vi "Main.vi"(11 "Module Admin":refnum<class "Delacor_lib_QMH_Module Admin.lvclass">) -> ()   [LabVIEW 2019, in "CML UI.lvlib"]
doc: "This template is based off of the Queued Message Handler design pattern and the Queued Message Handler project template that ships with LabVIEW.\n\nThe main difference is that the queue is private to this module and communication between modules is performed via Broadcast and Request events.\n\nRequest events are wrapped in public API methods and are handled in the Event Handling Loop (EHL) of this VI. Any module can register for Broadcast events sent by this module. The EHL generates messages based on user interface actions.\n\nThe Message Handling Loop (MHL) processes messages generated by the EHL, or by other messages. The messages are string values, so new messages can be added easily to the Message Cases case structure in the MHL. Each message cluster can also provide an optional value for Message Data, which is a variant that can be converted to whatever message-specific data is required.\n_____\nBased on Delacor QMH Project Template 4.0.0.47.\n_____\nBased on DQMH Project Template 6.1.0.94.\n\n<b>Note:</b> This VI was modified by the <b>Validate DQMH Module</b> tool to add a call to the Error Reported VI at the end of the 'Exit' MHL frame."
uses:
  CML UI.lvlib
  <vilib>/Delacor/Delacor QMH/Libraries/Module Admin_class/Delacor_lib_QMH_Module Admin.lvclass
  Module Data--cluster.ctl
  Acquisition State.ctl
  Measurement UI Displays.ctl
  CNV demo Helper Loop Data--cluster.ctl
  Stop Argument--cluster.ctl
  <vilib>/Delacor/Delacor QMH/Libraries/Message Queue_class/Delacor_lib_QMH_Message Queue.lvclass/Delacor_lib_QMH_Message Queue.ctl
  <vilib>/event_ctls.llb/eventvkey.ctl
  STOP_GUI Argument--cluster.ctl
  Clear All Charts Argument--cluster.ctl
  Update Data Status UI Argument--cluster.ctl
  Update Packet Loss (%) Argument--cluster.ctl
  <vilib>/Utility/sysdir.llb/System Directory Type.ctl
  <vilib>/Delacor/Delacor QMH/Libraries/Module Admin_class/Delacor_lib_QMH_Module Admin.lvclass/Delacor_lib_QMH_Module Admin.ctl
  UI Tab Select.ctl
  Acquisition/WiBCI16T_Data.ctl
  Acquisition/WiBCI16T_Status.ctl
  Acquisition/Reg_Map.ctl
  <vilib>/Analysis/3filter.llb/Filter Passband Type.ctl
  Settings Editor/Settings--cluster.ctl
  Acquisition/Signal Type--enum.ctl
  Acquisition/Calibration Values--cluster.ctl
  CML Shared/EEG Channel Settings.ctl
  <vilib>/Delacor/Delacor QMH/Libraries/Message Queue_class/Delacor_lib_QMH_Enqueue Message (Single).vi
  <vilib>/Delacor/Delacor QMH/Libraries/Module Admin_class/Delacor_lib_QMH_Get External Launch.vi
  <vilib>/Analysis/baseanly.llb/Mean (DBL).vi
  <userlib>/_MGI/Timing/MGI Wait/MGI Wait (U32).vi
  <vilib>/addons/Biomedical/Biosignal Measurements/EEG/EEG FFT Spectrum (Waveform).vi
  <vilib>/Utility/error.llb/Error Cluster From Error Code.vi
  <vilib>/ErrorRing/Error Ring.xnode
  <vilib>/Delacor/Delacor QMH/Libraries/Message Queue_class/Delacor_lib_QMH_Message Queue.lvclass
  Settings Editor/Settings Editor.lvlib
  Acquisition/Acquisition.lvlib
  Logger/Logger.lvlib
  CML Shared/CML Shared.lvlib
  <vilib>/Analysis/NI_AALBase.lvlib
  <vilib>/addons/Biomedical/NI_BMTK_Measurements.lvlib
  DemoData Generator/DemoData Generator.lvlib
  Lab Streaming Layer/Lab Streaming Layer.lvlib
  <vilib>/ptbypt/NI_PtbyPt.lvlib
panel:
  out "Packet Loss (%)":dbl format="%#_3g"
  out "LSL Listeners":string
  out "En/Dis Trig":string
  in  "Settings":bool
  in  "Ref":bool
  out "Data Status":bool=TRUE
  out "Battery":u8(slide) scale=0.0..100.0
  in  "UI Page":T1(tab)
  out "Data Trig":i8(graph)
  out "Data 16":dbl(graph)
  out "Data 15":dbl(graph)
  out "Data 14":dbl(graph)
  out "Data 13":dbl(graph)
  out "Data 12":dbl(graph)
  out "Data 11":dbl(graph)
  out "Data 10":dbl(graph)
  out "Data 9":dbl(graph)
  out "Data 8":dbl(graph)
  out "Data 7":dbl(graph)
  out "Data 6":dbl(graph)
  out "Data 5":dbl(graph)
  out "Data 4":dbl(graph)
  out "Data 3":dbl(graph)
  out "Data 2":dbl(graph)
  out "Data 1":dbl(graph)
  in  "Stop":bool
  in  "Start":bool
  in  "Record Button":bool
  in  "Data Select":string(combo)="Live Data"
  out "Status":string
  out "G.Ch Name 1":string
  out "G.Ch Name 2":string
  out "G.Ch Name 3":string
  out "G.Ch Name 4":string
  out "G.Ch Name 5":string
  out "G.Ch Name 6":string
  out "G.Ch Name 7":string
  out "G.Ch Name 8":string
  out "G.Ch Name 9":string
  out "G.Ch Name 10":string
  out "G.Ch Name 11":string
  out "G.Ch Name 12":string
  out "G.Ch Name 13":string
  out "G.Ch Name 14":string
  out "G.Ch Name 15":string
  out "G.Ch Name 16":string
  in  "imp mode":bool
  out "ch 11":string
  out "ch 12":string
  out "ch 13":string
  out "ch 14":string
  out "ch 15":string
  out "ch 16":string
  out "ch 10":string
  out "ch 9":string
  out "ch 8":string
  out "ch 7":string
  out "ch 6":string
  out "ch 5":string
  out "ch 4":string
  out "ch 3":string
  out "ch 2":string
  out "ch 1":string
  in  "Stop Imped":bool
  in  "Start Imped":bool
  out "Imp Ch 16":bool
  out "Imp Ch 15":bool
  out "Imp Ch 14":bool
  out "Imp Ch 13":bool
  out "Imp Ch 12":bool
  out "Imp Ch 11":bool
  out "Imp Ch 10":bool
  out "Imp Ch 9":bool
  out "Imp Ch 8":bool
  out "Imp Ch 7":bool
  out "Imp Ch 6":bool
  out "Imp Ch 5":bool
  out "Imp Ch 4":bool
  out "Imp Ch 3":bool
  out "Imp Ch 2":bool
  out "Imp Ch 1":bool
  in  "Round Color Box 1":u32(colorbox)=16777215
  in  "Round Color Box 2":u32(colorbox)=3381759
  in  "Round Color Box 3":u32(colorbox)=6618880
  in  "Round Color Box 4":u32(colorbox)=16749312
  in  "Round Color Box 5":u32(colorbox)=16731714
  out "Ch Name 1":string
  out "Ch Name 2":string
  out "Ch Name 3":string
  out "Ch Name 4":string
  out "Ch Name 5":string
  out "Ch Name 6":string
  out "Ch Name 7":string
  out "Ch Name 8":string
  out "Ch Name 9":string
  out "Ch Name 10":string
  out "Ch Name 11":string
  out "Ch Name 12":string
  out "Ch Name 13":string
  out "Ch Name 14":string
  out "Ch Name 15":string
  out "Ch Name 16":string
  out "Single Chart":dbl(graph)
  in  "Visual Cue Tab":enum32{"Visual Cue Graph", "Ready", "Rest"}(tab)
  out "Visual Cue":i32[][](graph)
  in  "Display CNV Tab":enum32{"Empty", "Graph"}(tab)
  out "CNV Graph":dbl[][](graph)
  in  "Start CNV":bool
  in  "Stop CNV":bool
  in  "Record CNV":bool
  in  "Record EOC":bool
  in  "Stop EOC":bool
  in  "Start EOC":bool
  out "Theta":u8(slide) scale=10.0..90.0
  out "Alpha":u8(slide) scale=10.0..90.0
  out "Beta":u8(slide) scale=10.0..90.0
  out "Display Label EOC":string
  in  "About DQMH":bool
  out "Logger Running?":bool
  out "Settings Editor Running?":bool
  out "Acquisition Running?":bool
  out "Calibrated?":bool
  in  "Calibrate":bool
  out "error out":errorcluster
  out "version":string
  # "Connection"
  # "TRIG"
  # "Ch. 1"
  # "Ch. 9"
  # "Ch. 2"
  # "Ch. 10"
  # "Legend"
  # "Unknown"
  # "Ch. 3"
  # "Ch. 11"
  # "Excellent"
  # "Ch. 4"
  # "Ch. 12"
  # "Good"
  # "Average"
  # "Ch. 5"
  # "Ch. 13"
  # "Bad"
  # "Ch. 6"
  # "Ch. 14"
  # "Ch. 7"
  # "Ch. 15"
  # "Ch. 8"
  # "Ch. 16"
  # "Ready !"
  # "Rest"
  # "Theta"
  # "Alpha"
  # "Beta"
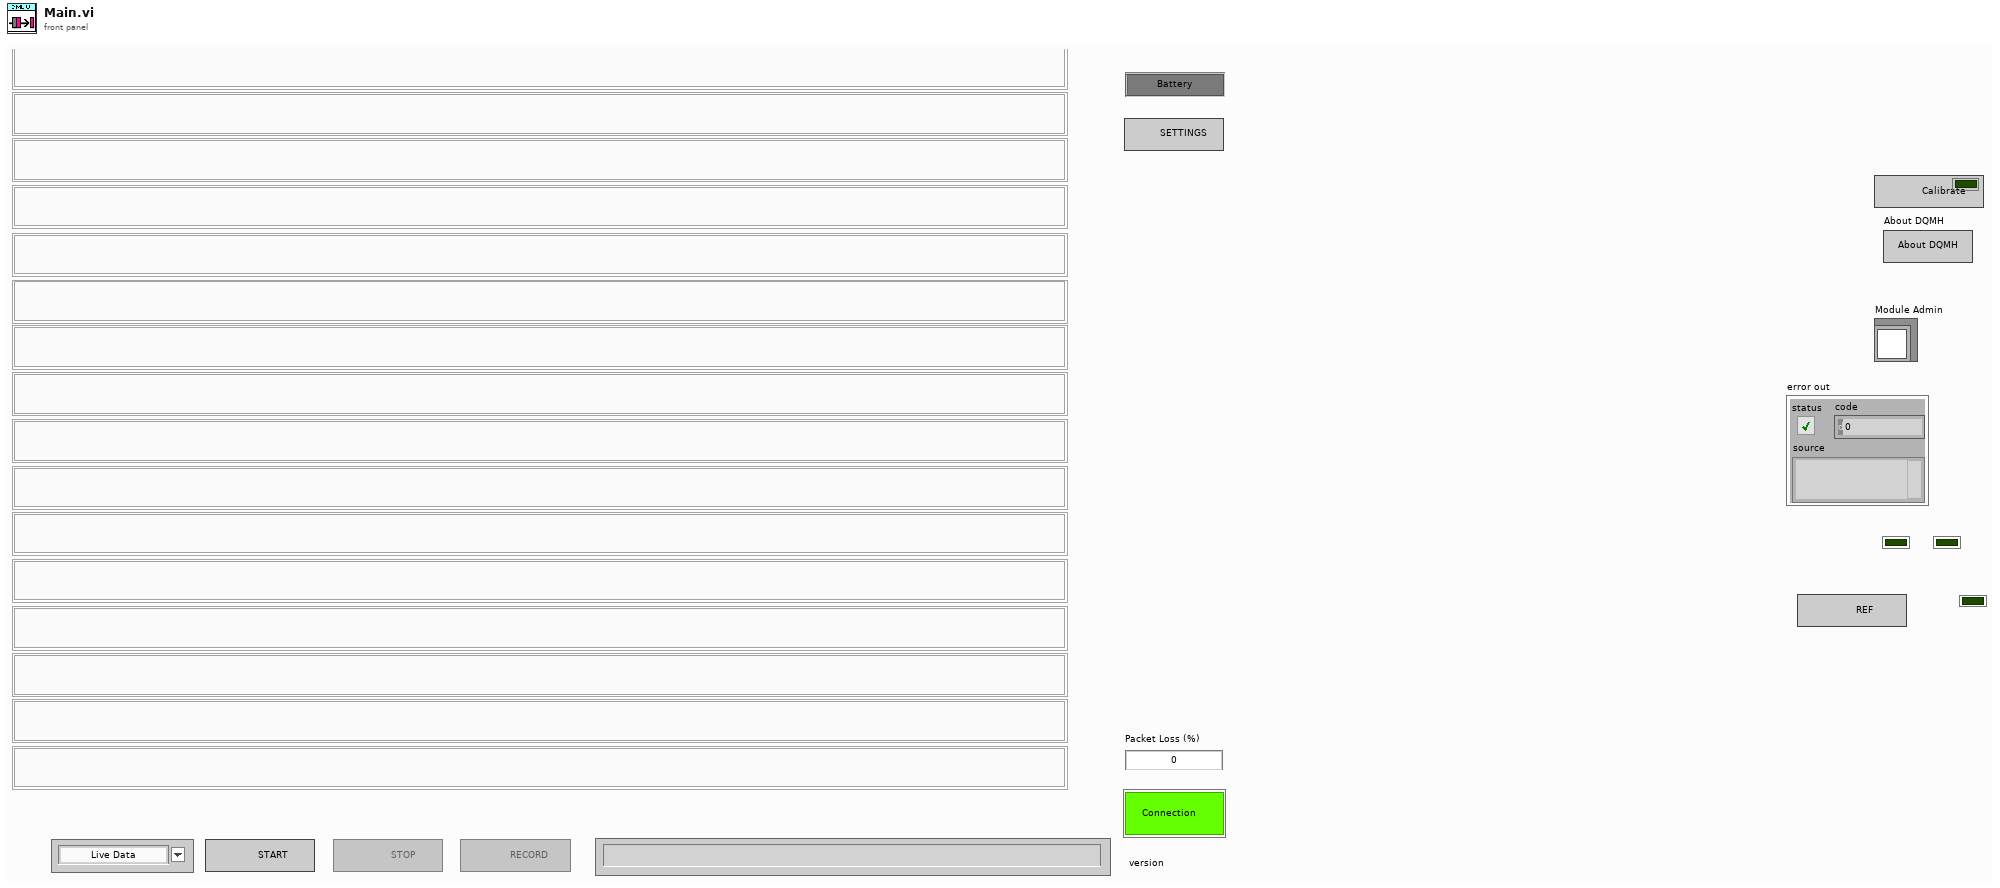
[diagram p1: front panel]
types:
  T1 = enum32{"Graph", "Impedance", "More Options", "Single Graph", "CNV Demo", "Eyes O/C Demo"}
  T2 = typedef "Settings Editor.lvlib/Broadcast Events--cluster.ctl" = cluster{"Module Did Init":refnum<user-event>, "Status Updated":refnum<user-event>, "Error Reported":refnum<user-event>, "Module Did Stop":refnum<user-event>, "Update Module Execution Status":refnum<user-event>, "Application Settings Updated":refnum<user-event>}
  T3 = typedef "Acquisition.lvlib/Broadcast Events--cluster.ctl" = cluster{"Module Did Init":refnum<user-event>, "Status Updated":refnum<user-event>, "Error Reported":refnum<user-event>, "Module Did Stop":refnum<user-event>, "Update Module Execution Status":refnum<user-event>, "Acquisition Started":refnum<user-event>, "Acquisition Stopped":refnum<user-event>, "Data Updated":refnum<user-event>, "Device Calibrated":refnum<user-event>, "Impedance Data Updated":refnum<user-event>, "CNV Data Updated":refnum<user-event>, "EOC Data Updated":refnum<user-event>}
  T4 = typedef "Logger.lvlib/Broadcast Events--cluster.ctl" = cluster{"Module Did Init":refnum<user-event>, "Status Updated":refnum<user-event>, "Error Reported":refnum<user-event>, "Module Did Stop":refnum<user-event>, "Update Module Execution Status":refnum<user-event>, "Logging Stopped":refnum<user-event>, "File Initialized":refnum<user-event>}
  T5 = typedef "DemoData Generator.lvlib/Broadcast Events--cluster.ctl" = cluster{"Module Did Init":refnum<user-event>, "Status Updated":refnum<user-event>, "Error Reported":refnum<user-event>, "Module Did Stop":refnum<user-event>, "Update Module Execution Status":refnum<user-event>, "Demo Data Generated":refnum<user-event>}
  T6 = typedef "Lab Streaming Layer.lvlib/Broadcast Events--cluster.ctl" = cluster{"Module Did Init":refnum<user-event>, "Status Updated":refnum<user-event>, "Error Reported":refnum<user-event>, "Module Did Stop":refnum<user-event>, "Update Module Execution Status":refnum<user-event>}
  T7 = typedef "CML UI.lvlib/Request Events--cluster.ctl" = cluster{"Stop Module":refnum<user-event>, "Show Panel":refnum<user-event>, "Hide Panel":refnum<user-event>, "Get Module Execution Status":refnum<user-event>, "Show Diagram":refnum<user-event>, "STOP_GUI":refnum<user-event>, "Clear All Charts":refnum<user-event>, "Update Data Status UI":refnum<user-event>, "Private":cluster{"Wake-Up File Name Query Loop":refnum<user-event>, "Wake-up CNV Demo Loop":refnum<user-event>, "Sleep CNV Demo Loop":refnum<user-event>, "Menu -- About Display Box":refnum<user-event>, "Wake-Up Copy MATLAB files":refnum<user-event>}, "Update Packet Loss (%)":refnum<user-event>}
  T8 = typedef "CML UI.lvlib/CNV demo Helper Loop Data--cluster.ctl" = cluster{"Visual Cue Tab":refnum<vi>, "Display CNV Tab":refnum<vi>, "Visual Cue Graph":refnum<vi>, "CNV Runner":cluster{"fixed array":i32[], "Loop Counter":i32}, "CNV Graph":refnum<vi>}
  T9 = typedef "CML UI.lvlib/Module Data--cluster.ctl" = cluster{"Status":string, "Measurement UI Controls":cluster{"Start Ref":refnum<vi>, "Stop Ref":refnum<vi>, "Settings Ref":refnum<vi>, "Status Ref":refnum<vi>, "Data Ref":refnum<vi>, "Rec Ref":refnum<vi>, "Soft Trig":refnum<vi>, "Imp Start Ref":refnum<vi>, "Imp Stop Ref":refnum<vi>, "CNV Start Ref":refnum<vi>, "CNV Stop Ref":refnum<vi>, "CNV Rec":refnum<vi>, "Recording State CNV":refnum<vi>, "EOC Start Ref":refnum<vi>, "EOC Stop Ref":refnum<vi>, "EOC Rec Ref":refnum<vi>, "CNV Rec state":refnum<vi>, "Recording State EOC":refnum<vi>}, "Recording State":bool, "Impedance":cluster{"Ch 1":dbl, "Ch 2":dbl, "Ch 3":dbl, "Ch 4":dbl, "Ch 5":dbl, "Ch 6":dbl, "Ch 7":dbl, "Ch 8":dbl, "Ch 9":dbl, "Ch 10":dbl, "Ch 11":dbl, "Ch 12":dbl, "Ch 13":dbl, "Ch 14":dbl, "Ch 15":dbl, "Ch 16":dbl}, "menu reference ":refnum<k9>, "Acq State":T10, "En/Dis Trig":refnum<vi>, "Soft Trigger En?":bool, "Display  cnt":u8, "UI Page":refnum<vi>, "CNV Demo Data":cluster{"Rebuild Vector":dbl[][], "CNV Buffer Action":enum16{"Stop Buffer Fill", "Start Buffer Fill", "Analyze Buffer"}, "Index of R.Array":u16, "Run Sum CNV":dbl[], "CNV Iter":u16}, "EOC Demo Data":cluster{"Running Buffer":dbl[], "Index of R.Buffer":u8}, "Measurement UI Displays":T11, "Recording State CNV":bool, "Recording State EOC":bool, "LSL En?":bool, "LSL Listeners":refnum<vi>, "Imp Mode":bool}
  T10 = typedef "CML UI.lvlib/Acquisition State.ctl" = enum16{"RUNNING", "IDLE"}
  T11 = typedef "CML UI.lvlib/Measurement UI Displays.ctl" = cluster{"Graph 1":refnum<vi>, "Graph 2":refnum<vi>, "Graph 3":refnum<vi>, "Graph 4":refnum<vi>, "Graph 5":refnum<vi>, "Graph 6":refnum<vi>, "Graph 7":refnum<vi>, "Graph 8":refnum<vi>, "Graph 9":refnum<vi>, "Graph 10":refnum<vi>, "Graph 11":refnum<vi>, "Graph 12":refnum<vi>, "Graph 13":refnum<vi>, "Graph 14":refnum<vi>, "Graph 15":refnum<vi>, "Graph 16":refnum<vi>, "Battery 2":refnum<vi>, "Data Trig":refnum<vi>, "Data Connection Status":refnum<vi>, "Graph Sel":u8, "En MAP":u16, "Single Chart":refnum<vi>, "G.Ch Name 1":refnum<vi>, "G.Ch Name 2":refnum<vi>, "G.Ch Name 3":refnum<vi>, "G.Ch Name 4":refnum<vi>, "G.Ch Name 5":refnum<vi>, "G.Ch Name 6":refnum<vi>, "G.Ch Name 7":refnum<vi>, "G.Ch Name 8":refnum<vi>, "G.Ch Name 9":refnum<vi>, "G.Ch Name 10":refnum<vi>, "G.Ch Name 11":refnum<vi>, "G.Ch Name 12":refnum<vi>, "G.Ch Name 13":refnum<vi>, "G.Ch Name 14":refnum<vi>, "G.Ch Name 15":refnum<vi>, "G.Ch Name 16":refnum<vi>, "imp mode sel":refnum<vi>}
  T12 = enum32{"invalid lock state", "Not Locked", "Locked (No Password)", "Password-protected"}
  T13 = typedef "CML UI.lvlib/Stop Argument--cluster.ctl" = cluster{"Origin":string, "Exit via Stop Module Req?":bool, "Wait for Module to stop?":bool}
  T14 = typedef "eventvkey.ctl" = enum16{"ASCII", "Enter", "Return", "Shift", "Ctrl", "Alt", "Cmd", "Opt", "Caps", "NumLock", "Clear", "Break", "Up", "Down", "Left", "Right", "Insert", "Delete", "Home", "End", "PageUp", "PageDown", "Escape", "Help", "Pause", "ScrollLock", "F1", "F2", "F3", "F4", "F5", "F6", "F7", "F8", "F9", "F10", "F11", "F12", "F13", "F14", "F15", "F16", "F17", "F18", "F19", "F20", "F21", "F22", "F23", "F24", "Play", "VolumeUp", "VolumeDown", "Mute", "Two Byte Char"}
  T15 = typedef "CML UI.lvlib/STOP_GUI Argument--cluster.ctl" = cluster{"Message for the Request":string}
  T16 = typedef "CML UI.lvlib/Clear All Charts Argument--cluster.ctl" = cluster{"Boolean":bool}
  T17 = typedef "CML UI.lvlib/Update Data Status UI Argument--cluster.ctl" = cluster{"status":bool}
  T18 = typedef "CML UI.lvlib/Update Packet Loss (%) Argument--cluster.ctl" = cluster{"Paket Loss":dbl}
  T19 = enum32{"Invalid", "Standard", "Closed", "Hidden", "Minimized", "Maximized"}
  T20 = typedef "CML UI.lvlib/UI Tab Select.ctl" = enum32{"Graph", "Impedance", "More Options", "Single Graph", "CNV Demo", "Eyes O/C Demo"}
  T21 = typedef "Acquisition.lvlib/WiBCI16T_Data.ctl" = cluster{"EEG Ch 1":dbl, "EEG Ch 2":dbl, "EEG Ch 3":dbl, "EEG Ch 4":dbl, "EEG Ch 5":dbl, "EEG Ch 6":dbl, "EEG Ch 7":dbl, "EEG Ch 8":dbl, "EEG Ch 9":dbl, "EEG Ch 10":dbl, "EEG Ch 11":dbl, "EEG Ch 12":dbl, "EEG Ch 13":dbl, "EEG Ch 14":dbl, "EEG Ch 15":dbl, "EEG Ch 16":dbl, "X-Accel":i16, "Y-Accel":i16, "Z-Accel":i16, "X-Gyro":i16, "Y-Gyro":i16, "Z-Gyro":i16, "Timer":u32, "Packet ID":u32, "HW Trig1":u8, "SW Trig1":i8, "HW Trig2":u8, "SW Trig2":i8, "WiBCI Status":T22, "Reg Map":T23}
  T22 = typedef "Acquisition.lvlib/WiBCI16T_Status.ctl" = cluster{"Mode Byte":u8, "Ch Config":u8, "Ch Ref Map":u16, "Ch Enable Map":u16, "Temperature":sgl, "Battery":u8, "Version":string}
  T23 = typedef "Acquisition.lvlib/Reg_Map.ctl" = cluster{"ADS1":u8[], "ADS2":u8[]}
  T24 = typedef "NI_AALBase.lvlib/Filter Passband Type.ctl" = enum32{"Lowpass", "Highpass", "Bandpass", "Bandstop"}
  T25 = enum16{"Stop Buffer Fill", "Start Buffer Fill", "Analyze Buffer"}
  T26 = typedef "Settings Editor.lvlib/Settings--cluster.ctl" = cluster{"Signal Type":T27, "Calibration Array":T28[], "Log File Base Path":path, "EEG Channels":T29, "Soft Trig enum":enum16{"Disable Soft Trigger", "Enable Soft Trigger"}, "Montage selection":cluster{"Montages Ref":refnum<vi>, "Selected Montage Number":u8, "Montages Names":string[]}, "LSL En enum":enum16{"LSL Disabled", "LSL Enabled"}}
  T27 = typedef "Acquisition.lvlib/Signal Type--enum.ctl" = enum16{"Sine Wave", "Square with Noise"}
  T28 = typedef "Acquisition.lvlib/Calibration Values--cluster.ctl" = cluster{"Slope":dbl, "Offset":dbl}
  T29 = typedef "CML Shared.lvlib/EEG Channel Settings.ctl" = cluster{"16 EEG Channels":cluster{"Channel Name":string, "Channel No":u8, "Channel Enabled":bool, "Channel Referenced":bool}[], "Gain":u8}
  T30 = typedef "Settings Editor.lvlib/Update Application Settings (Reply Payload)--cluster.ctl" = cluster{"Settings":T26, "error":errorcluster}
  T31 = cluster{"Channel Name":string, "Channel No":u8, "Channel Enabled":bool, "Channel Referenced":bool}[]
  T32 = typedef "NI_BMTK_Measurements.lvlib/bmt_EEG Frequency-domain Measures.ctl" = cluster{"delta power":dbl, "theta power":dbl, "alpha power":dbl, "beta power":dbl, "delta [%]":dbl, "theta [%]":dbl, "alpha [%]":dbl, "beta [%]":dbl}
  T33 = enum16{"Disable Soft Trigger", "Enable Soft Trigger"}
  T34 = typedef "System Directory Type.ctl" = i32
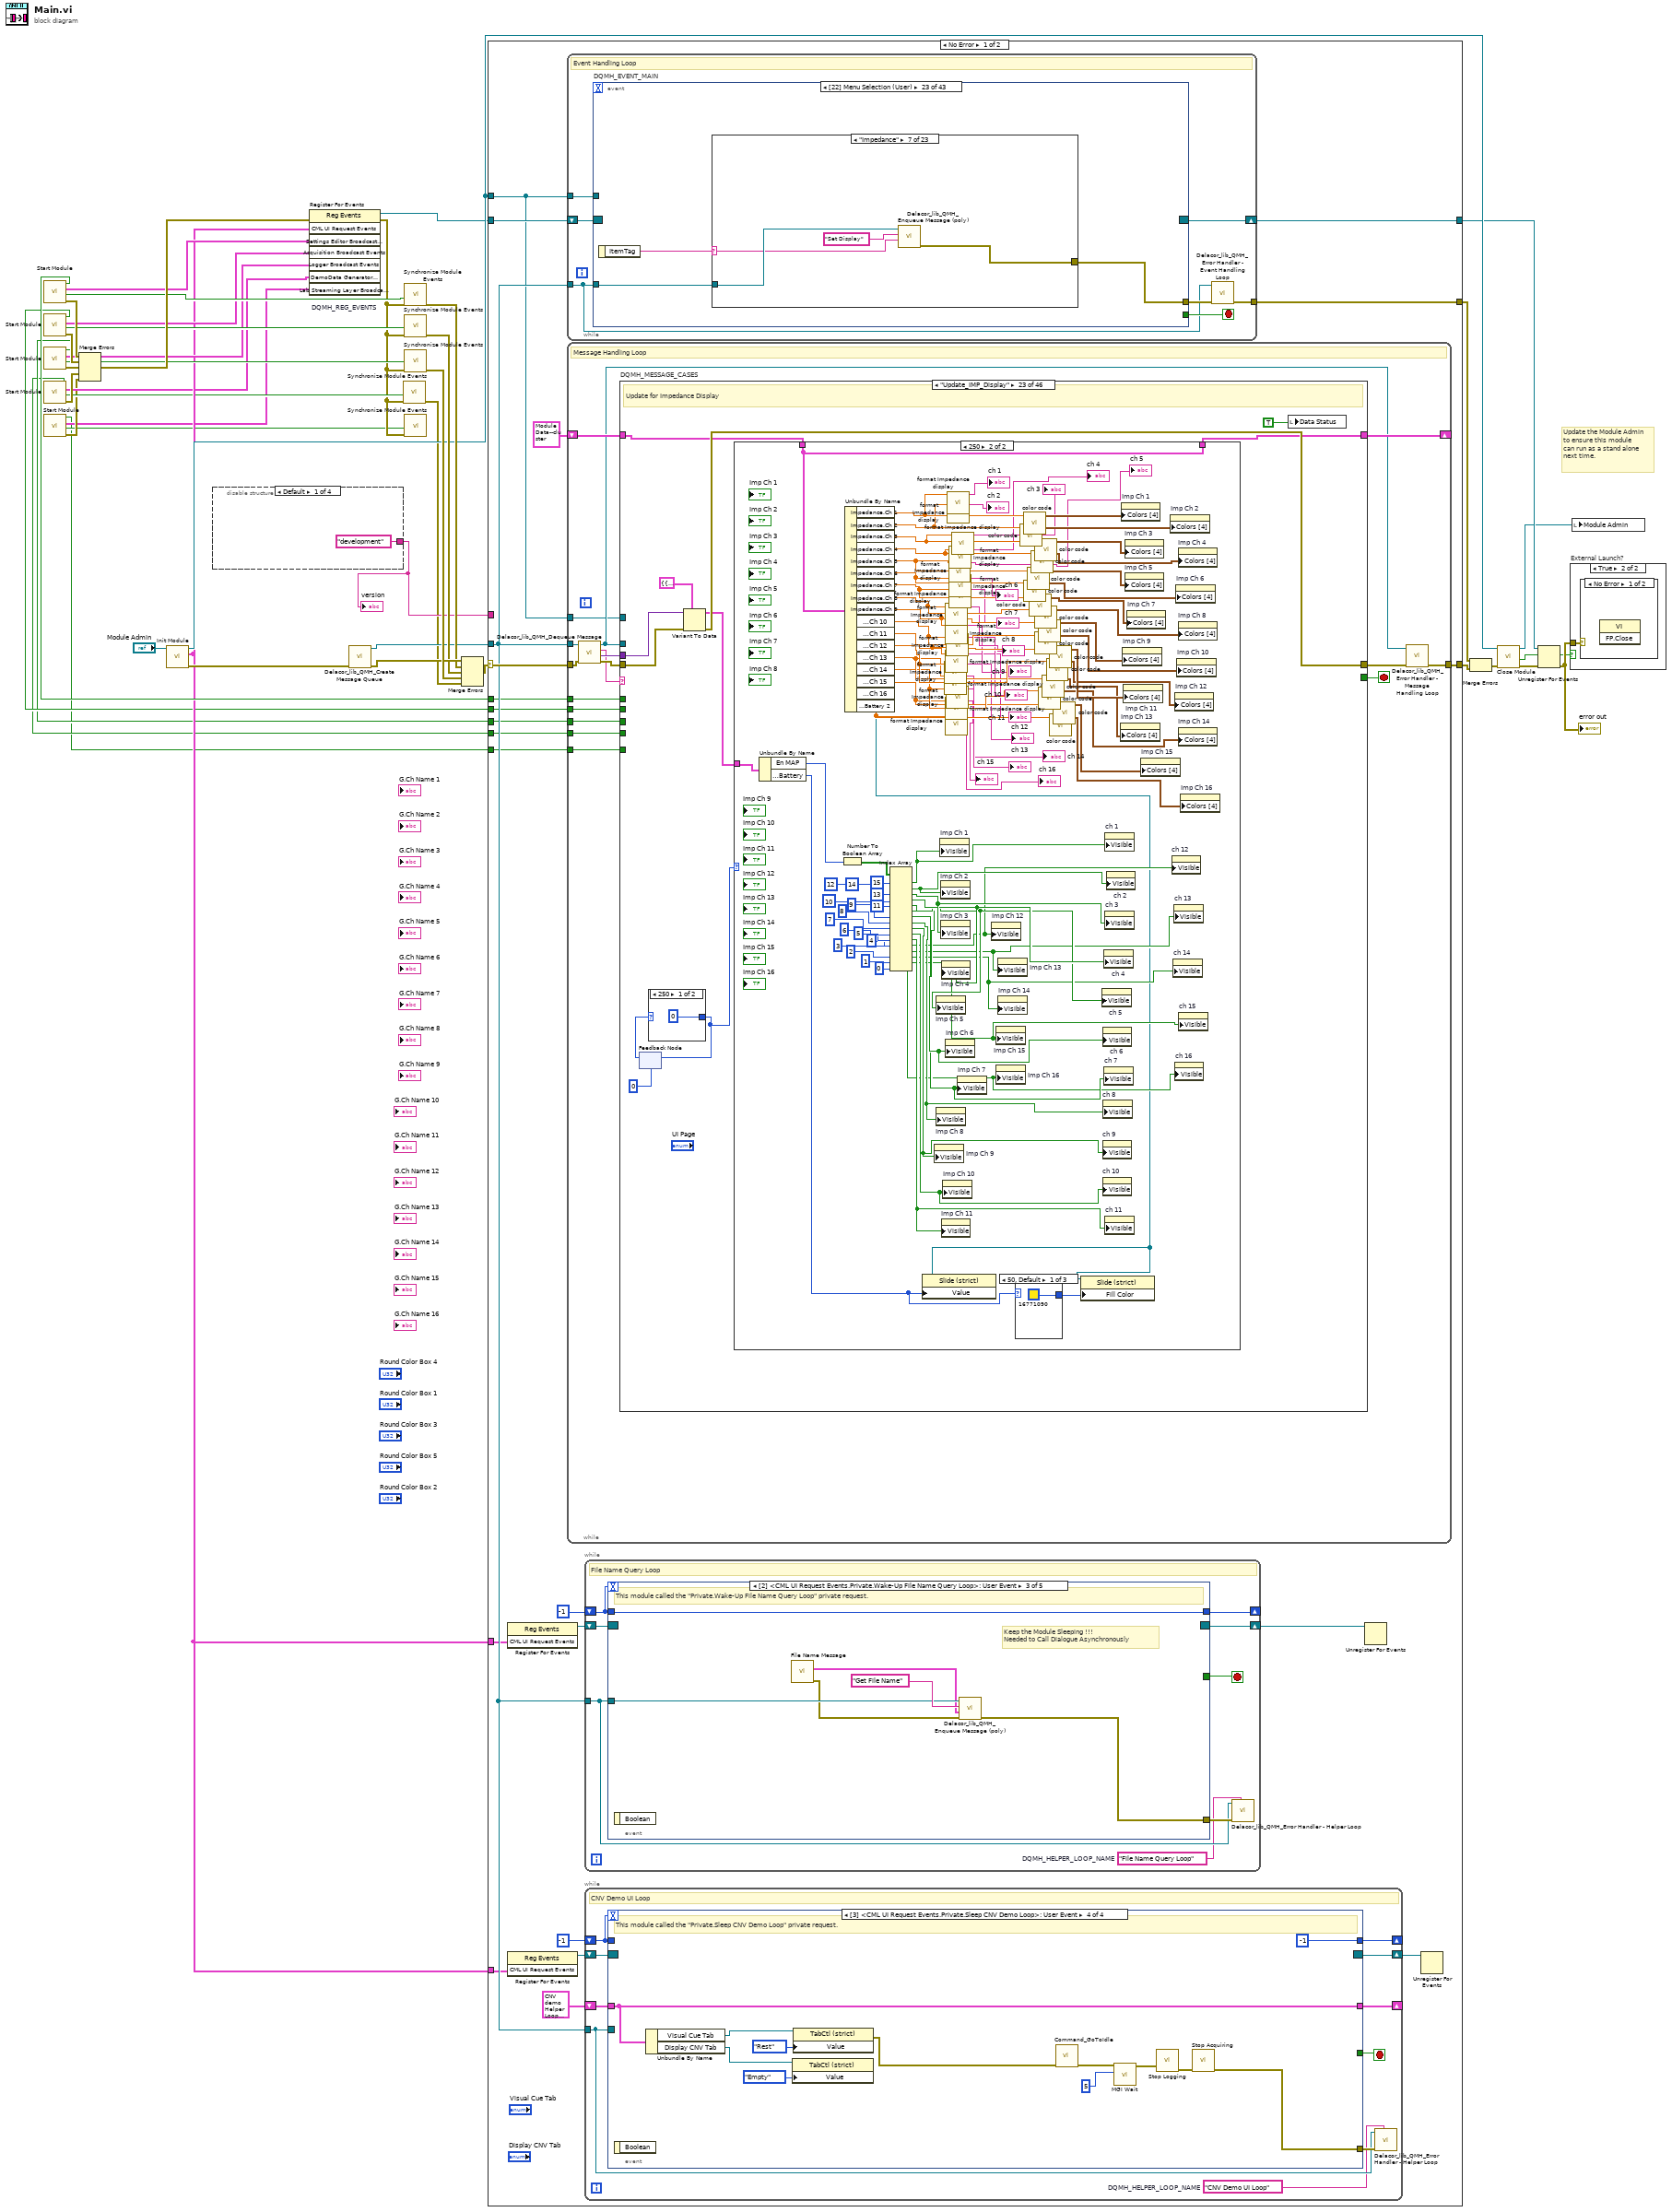
[diagram p0: block diagram]
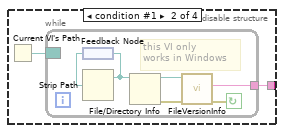
[diagram p2: hidden frame]
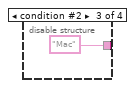
[diagram p3: hidden frame]
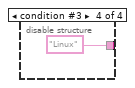
[diagram p4: hidden frame]
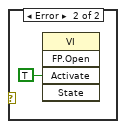
[diagram p6: hidden frame]
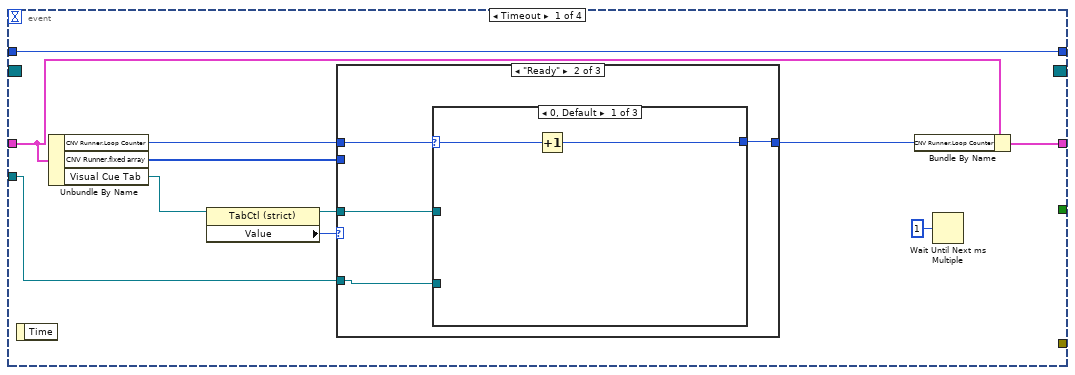
[diagram p7: hidden frame]
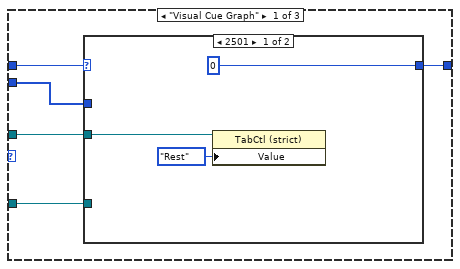
[diagram p8: hidden frame]
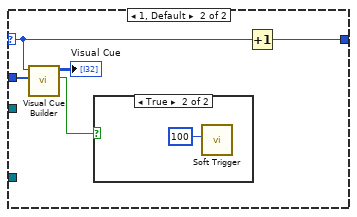
[diagram p9: hidden frame]
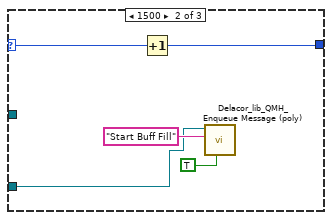
[diagram p11: hidden frame]
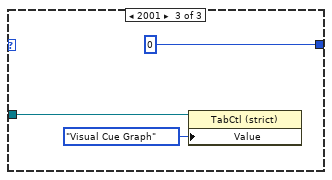
[diagram p12: hidden frame]
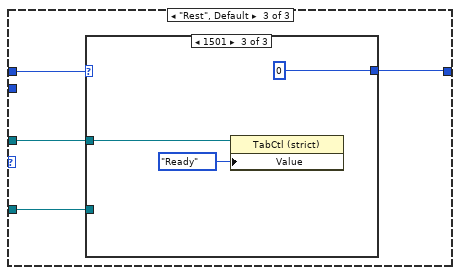
[diagram p13: hidden frame]
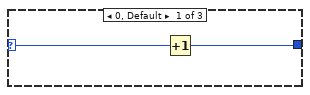
[diagram p14: hidden frame]
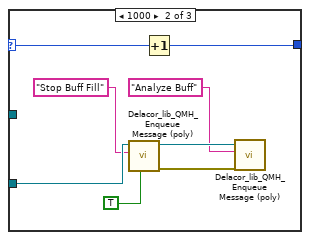
[diagram p15: hidden frame]
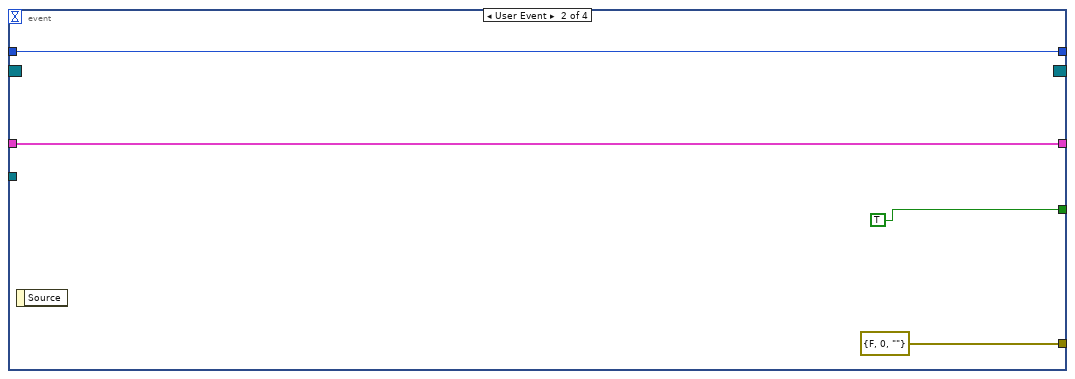
[diagram p16: hidden frame]
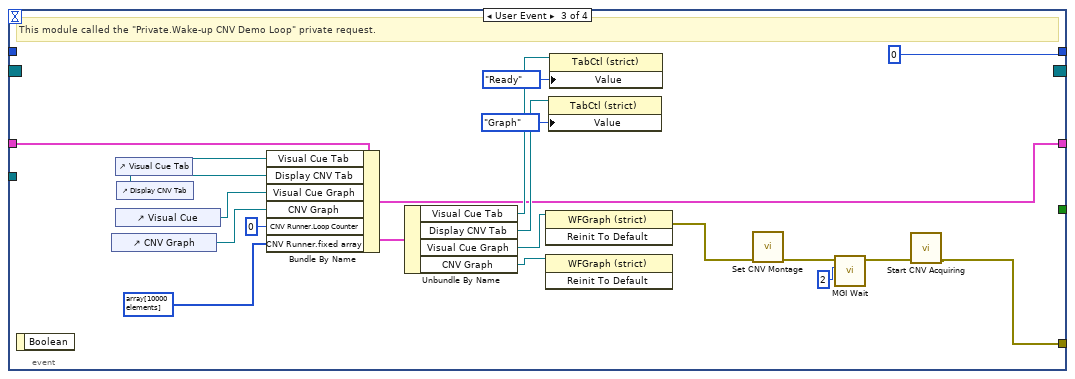
[diagram p17: hidden frame]
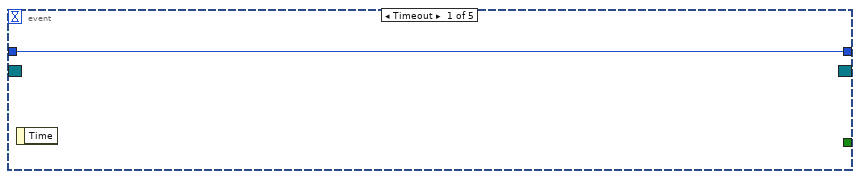
[diagram p18: hidden frame]
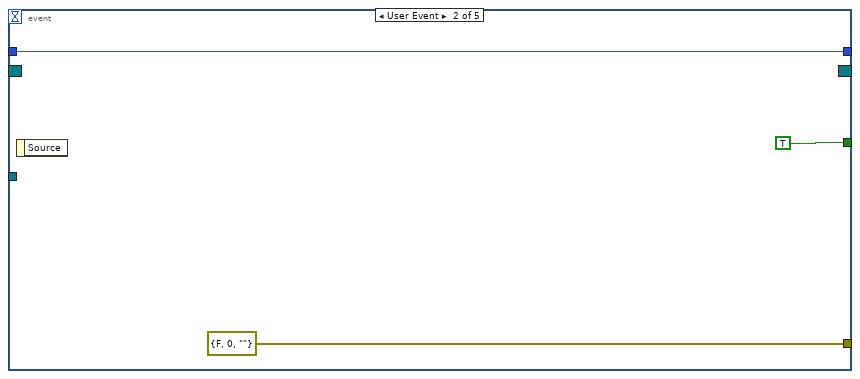
[diagram p19: hidden frame]
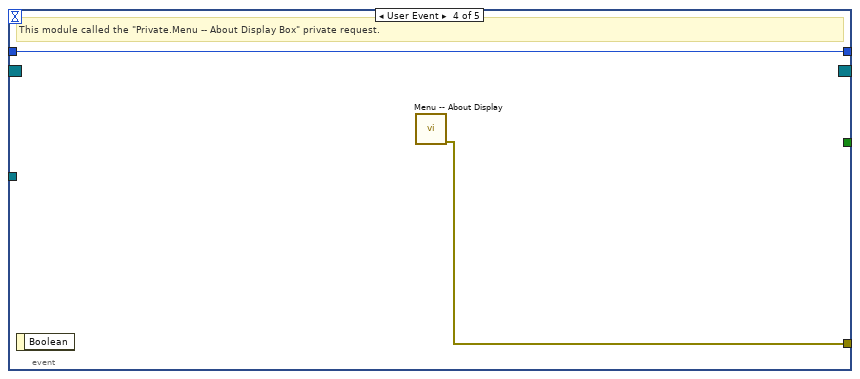
[diagram p20: hidden frame]
diagram:
  # "Update the Module Admin to ensure this module can run as a stand alone next time."
  n1 = call "Start Module.vi"() -> ("error out"=w32:errorcluster, "Wait for Event Sync?"=w21:bool, "Settings Editor Broadcast Events"=w20:T2, "Module Was Already Running?"=w14:bool)  [unwired: 8 in]
  n2 = call "Start Module.vi"() -> ("error out"=w31:errorcluster, "Wait for Event Sync?"=w18:bool, "Acquisition Broadcast Events"=w19:T3, "Module Was Already Running?"=w4:bool)  [unwired: 8 in]
  n3 = call "Start Module.vi"() -> ("error out"=w30:errorcluster, "Wait for Event Sync?"=w16:bool, "Logger Broadcast Events"=w17:T4, "Module Was Already Running?"=w3:bool)  [unwired: 8 in]
  n4 = call "Start Module.vi"() -> ("error out"=w12:errorcluster, "Wait for Event Sync?"=w10:bool, "DemoData Generator Broadcast Events"=w11:T5, "Module Was Already Running?"=w2:bool)  [unwired: 8 in]
  n5 = call "Start Module.vi"() -> ("error out"=w8:errorcluster, "Wait for Event Sync?"=w6:bool, "Lab Streaming Layer Broadcast Events"=w5:T6, "Module Was Already Running?"=w1:bool)  [unwired: 8 in]
  n6 = Merge Errors(w32, w31, w30, w12, w8) -> (w29:errorcluster)
  n7 = call "Init Module.vi"("Singleton Module Admin in"="Module Admin") -> ("error out"=w41:errorcluster, "CML UI Request Events"=w13:T7, "Singleton Module Admin out"=w28:refnum<class "Delacor_lib_QMH_Module Admin.lvclass">)  [unwired: 8 in]
  n8 = disable-structure "Conditional Disable Structure" shown="Default" {
    disable-tunnel: ["development" w45 "Mac" "Linux"] -> w15
    frame condition #0 (active) {
    }
    frame condition #1 {
      n9 = Current VI's Path() -> (path=w46:path)
      n10 = while {
        border: w46 -> [_]
        tunnel: [w47] -> w45
        stop <- w51 continue-if-true
        # "this VI only \nworks in Windows"
        n11 = feedback #1() -> (w50:path)
        n12 = Strip Path(path=w50) -> (stripped path=w49:path)  [unwired: 1 out]
        n13 = feedback-in #1(w49) -> ()
        n14 = File/Directory Info(path=w49) -> (path out=w48:path, error out=w52:errorcluster)  [unwired: 1 in, 5 out]
        n15 = call <vilib>:"FileVersionInfo.vi"("error in (no error)"=w52, "Application Path in"=w48) -> ("error out"=w51:errorcluster, "File Version Info"=w47:string)  [unwired: 6 in, 2 out]
      }
    }
    frame condition #2 {
    }
    frame condition #3 {
    }
  }
  "version" <- w15
  n16 = register-events "DQMH_REG_EVENTS"(error in=w29, w13, w20, w19, w17, w11, w5) -> (reference out=w26:refnum<event-registration>, error out=w7:errorcluster)  [unwired: 1 in]
  n17 = call <vilib>:"Delacor_lib_QMH_Create Message Queue.vi"("error in"=w41) -> ("error out"=w36:errorcluster, "Message Queue"=w25:refnum<class "Delacor_lib_QMH_Message Queue.lvclass">)  [unwired: 9 in]
  n18 = call "Synchronize Module Events.vi"("error in"=w7, "Wait for Event Sync?"=w10) -> ("error out"=w9:errorcluster)  [unwired: 9 in]
  n19 = call "Synchronize Module Events.vi"("error in (no error)"=w7, "Wait for Event Sync?"=w21) -> ("error out"=w34:errorcluster)  [unwired: 9 in]
  n20 = call "Synchronize Module Events.vi"("error in (no error)"=w7, "Wait for Event Sync?"=w18) -> ("error out"=w33:errorcluster)  [unwired: 9 in]
  n21 = call "Synchronize Module Events.vi"("error in (no error)"=w7, "Wait for Event Sync?"=w16) -> ("error out"=w43:errorcluster)  [unwired: 9 in]
  n22 = call "Synchronize Module Events.vi"("error in"=w7, "Wait for Event Sync?"=w6) -> ()  [unwired: 9 in, 1 out]
  n23 = Merge Errors(w36, w34, w33, w43, w9) -> (w35:errorcluster)
  n24 = case shown="No Error" w35 {
    selector: w35 -> [w74 w1637]
    tunnel: [w76 w1636] -> w42
    tunnel: [w73 w1645] -> w27
    tunnel: w26 -> [w71 w1645]
    tunnel: w25 -> [w70 w1638]
    tunnel: [w75 _] -> w39
    tunnel: w28 -> [w69 w1641]
    tunnel: w15 -> [_ _]
    tunnel: w14 -> [w68 _]
    tunnel: w13 -> [w67 _]
    tunnel: w13 -> [w63 _]
    tunnel: w4 -> [w58 _]
    tunnel: w3 -> [w57 _]
    tunnel: w2 -> [w56 _]
    tunnel: w1 -> [w55 _]
    frame No Error {
      n25 = register-events ("DQMH_HELPER_REGFOREVENTS")(w67) -> (reference out=w65:refnum<event-registration>)  [unwired: 2 in, 1 out]
      n26 = register-events ("DQMH_HELPER_REGFOREVENTS")(w63) -> (reference out=w61:refnum<event-registration>)  [unwired: 2 in, 1 out]
      n27 = while {
        tunnel: w70 -> [w220]
        shift-right: [w223] -> w73
        shift-left: w71 -> [w224]
        tunnel: [w225] -> w75
        tunnel: w69 -> [w221]
        stop <- w222 stop-if-true
        # "Event Handling Loop"
        n28 = event "DQMH_EVENT_MAIN" shown="[22] Menu Selection (User)" {
          selector: w224 -> [_ _ _ _ _ _ _ _ _ _ _ _ _ _ _ _ _ _ _ _ _ _ _ _ _ _ w417 _ _ _ _ _ _ _ _ _ _ _ _ _ _ _ _]
          dyn-events: [_ _ _ _ _ _ _ _ _ _ _ _ _ _ _ _ _ _ _ _ _ _ _ _ _ _ w417 _ _ _ _ _ _ _ _ _ _ _ _ _ _ _ _] -> w223
          timeout: _ -> [_ _ _ _ _ _ _ _ _ _ _ _ _ _ _ _ _ _ _ _ _ _ _ _ _ _ _ _ _ _ _ _ _ _ _ _ _ _ _ _ _ _ _]
          tunnel: [_ _ _ _ TRUE ("Discard?") _ _ _ _ _ _ _ _ _ _ _ _ _ _ _ _ _ _ _ _ _ _ _ _ _ _ _ _ _ _ _ _ _ _ _ _ _ _] -> w222
          tunnel: w220 -> [_ _ _ _ w249 w255 w259 w264 w269 w271 w274 w277 w280 w285 w289 w293 w296 w308 w318 w321 w324 _ w329 _ _ w406 _ _ _ _ w429 _ w434 w440 w446 w452 w458 _ _ w467 w474 _ w484]
          tunnel: [_ _ w232 _ w252 w257 w261 w263 w268 w270 w273 w278 w281 w284 w288 w292 w295 w310 w320 w323 w326 w327 w328 w400 _ w405 _ _ _ w427 _ _ w433 w439 w445 w451 w457 _ w461 w462 w469 _ w479] -> w226
          tunnel: w221 -> [_ _ _ _ _ _ _ _ _ _ _ _ _ _ _ _ _ _ _ _ _ _ _ _ _ _ _ _ _ _ _ _ _ _ _ _ _ _ _ _ _ _ _]
          event User Event {
            # "Show the panel of this VI, and send a status updated message to let listeners know."
            # "Another Module called the \"Show Panel\" API Method."
            n29 = event-data() -> ()  [unwired: 1 in, 1 out]
            n30 = control-ref of="This VI"() -> (w228:refnum<vi>)
            n31 = call "Open VI Panel.vi"("VI"=w228) -> ()  [unwired: 10 in, 1 out]
            n32 = call "Status Updated.vi"("Status"="Panel shown." ("format string")) -> ()  [unwired: 10 in, 1 out]
          }
          event User Event {
            # "Hide the panel of this VI, and send a status updated message to let listeners know."
            # "Another Module called the \"Hide Panel\" API Method."
            n33 = event-data() -> ()  [unwired: 1 in, 1 out]
            n34 = control-ref of="This VI"() -> (w230:refnum<vi>)
            n35 = call "Hide VI Panel.vi"("VI"=w230) -> ()  [unwired: 10 in, 1 out]
            n36 = call "Status Updated.vi"("Status"="Panel hidden." ("format string")) -> ()  [unwired: 10 in, 1 out]
          }
          event User Event {
            # "Another Module called the \"Get Module Execution Status\" API Method."
            n37 = event-data() -> ()  [unwired: 1 in, 1 out]
            n38 = call "Update Module Execution Status.vi"("Running?"=TRUE) -> ("error out"=w232:errorcluster)  [unwired: 10 in]
          }
          event User Event {
            # "Another Module called the \"Show Diagram\" API Method. This event is used for debugging."
            n39 = event-data() -> ()  [unwired: 1 in, 1 out]
            n40 = disable-structure shown="RUN_TIME_ENGINE==False" {
              frame condition #0 (active) {
                # "functionality not available in exe"
                n41 = invoke on="Invoke Node" class="VI" method="Lock State.Get"() -> (error out=w238:errorcluster, "Get Lock State"=w237:T12, "pwd in cache"=w234:bool)  [unwired: 4 in, 1 out]
                n42 = Equal?(x=T12."Password-protected", y=w237) -> (x = y?=w235:bool)
                n43 = Compound Arithmetic op=AND(w235, invert w234) -> (w233:bool)
                n44 = case shown="False" w233 {
                  tunnel: w238 -> [w241 _]
                  frame False {
                    n45 = property on="Property Node" class="VI"(error in=w241, "BDWin.Open"=TRUE ("Block Diagram Window:Open")) -> ()  [unwired: 1 in, 2 out]
                    n46 = call "Status Updated.vi"("Status"="Block Diagram shown." ("format string")) -> ()  [unwired: 10 in, 1 out]
                  }
                  frame True {
                    # "Password-protected VI, and the password is not in the cache. Do not show the diagram."
                  }
                }
              }
              frame condition #1 {
              }
            }
          }
          event User Event {
            # "The Stop Module Event can get fired from the Exit message in the MHL. The queue gets destroyed in that case. If the queue no longer exists, the Enqueue Exit as a priority message will return error 1. It is safe to ignore, because the module is already exiting."
            # "Another Module called the \"Stop Module\" API Method  or the Message Handling Loop below."
            n47 = event-data() -> ("Origin"=w248:string, "Exit via Stop Module Req?"=w244:bool, "Wait for Module to stop?"=w243:bool)  [unwired: 1 in]
            n48 = local write "Status"(w248) -> ()
            n49 = Bundle By Name(cluster=T13 {"Origin"="", "Exit via Stop Module Req?"=FALSE, "Wait for Module to stop?"=FALSE} ("Stop Argument"), "Exit via Stop Module Req?"=w244, "Wait for Module to stop?"=w243) -> (w242:T13)
            n50 = call-poly <vilib>:"Delacor_lib_QMH_Enqueue Message (poly).vi"("Priority Message? (F)"=TRUE, "Message Data"=w242, "Message"="Exit", "Message Queue in"=w249) -> ("error out"=w253:errorcluster)  [unwired: 6 in, 1 out]
            n51 = call <vilib>:"Clear Errors.vi"("error in (no error)"=w253, "specific error code to clear (0: all)"=1) -> ("error out"=w252:errorcluster)  [unwired: 4 in, 1 out]
          }
          event Panel Close? {
            w256 = TRUE  # Discard the event, the MHL is responsible for closing and stopping this VI.
            # "this is the top level application, it always exits"
            # "Hide the panel or send the 'Exit' message if the user clicks the 'X' on the module main VI panel."
            n52 = event-data() -> ()  [unwired: 1 in, 1 out]
            n53 = call-poly <vilib>:"Delacor_lib_QMH_Enqueue Message (poly).vi"("Message"="Exit", "Message Queue in"=w255) -> ("error out"=w257:errorcluster)  [unwired: 8 in, 1 out]
            n54 = event-data ("Event Filter Node")("Discard?"=w256) -> ()  [unwired: 1 in, 1 out]
          }
          event "Start": Value Change {
            n55 = event-data() -> ()  [unwired: 1 in, 1 out]
            n56 = call-poly <vilib>:"Delacor_lib_QMH_Enqueue Message (poly).vi"("Message Data"="Data Select", "Message"="Start", "Message Queue in"=w259) -> ("error out"=w261:errorcluster)  [unwired: 7 in, 1 out]
          }
          event "Start Imped": Value Change {
            n57 = event-data() -> ()  [unwired: 1 in, 1 out]
            n58 = call-poly <vilib>:"Delacor_lib_QMH_Enqueue Message (poly).vi"("Message Data"=TRUE, "Message"="Impedance Start", "Message Queue in"=w264) -> ("error out"=w263:errorcluster)  [unwired: 7 in, 1 out]
          }
          event "imp mode": Value Change {
            n59 = event-data() -> ("NewVal"=w266:bool)  [unwired: 1 in]
            n60 = call-poly <vilib>:"Delacor_lib_QMH_Enqueue Message (poly).vi"("Message Data"=w266, "Message"="Gnd Imp to Imp mode", "Message Queue in"=w269) -> ("error out"=w268:errorcluster)  [unwired: 7 in, 1 out]
          }
          event "Start CNV": Value Change {
            n61 = event-data() -> ()  [unwired: 1 in, 1 out]
            n62 = call-poly <vilib>:"Delacor_lib_QMH_Enqueue Message (poly).vi"("Message"="Start CNV Demo", "Message Queue in"=w271) -> ("error out"=w270:errorcluster)  [unwired: 8 in, 1 out]
          }
          event "Start EOC": Value Change {
            n63 = event-data() -> ()  [unwired: 1 in, 1 out]
            n64 = call-poly <vilib>:"Delacor_lib_QMH_Enqueue Message (poly).vi"("Message"="Start EOC Demo", "Message Queue in"=w274) -> ("error out"=w273:errorcluster)  [unwired: 8 in, 1 out]
          }
          event "Ref": Value Change {
            n65 = event-data() -> ()  [unwired: 1 in, 1 out]
            n66 = call-poly <vilib>:"Delacor_lib_QMH_Enqueue Message (poly).vi"("Message Data"="Ref", "Message"="Start Rec Impedance", "Message Queue in"=w277) -> ("error out"=w278:errorcluster)  [unwired: 7 in, 1 out]
          }
          event "Stop Imped": Value Change {
            n67 = event-data() -> ()  [unwired: 1 in, 1 out]
            n68 = call-poly <vilib>:"Delacor_lib_QMH_Enqueue Message (poly).vi"("Message"="Impedance Stop", "Message Queue in"=w280) -> ("error out"=w281:errorcluster)  [unwired: 8 in, 1 out]
          }
          event "Record Button": Value Change {
            n69 = event-data() -> ()  [unwired: 1 in, 1 out]
            n70 = call-poly <vilib>:"Delacor_lib_QMH_Enqueue Message (poly).vi"("Priority Message? (F)"=TRUE, "Message"="Record Action", "Message Queue in"=w285) -> ("error out"=w284:errorcluster)  [unwired: 7 in, 1 out]
          }
          event "Record CNV": Value Change {
            n71 = event-data() -> ()  [unwired: 1 in, 1 out]
            n72 = call-poly <vilib>:"Delacor_lib_QMH_Enqueue Message (poly).vi"("Priority Message? (F)"=TRUE, "Message"="Record Action CNV", "Message Queue in"=w289) -> ("error out"=w288:errorcluster)  [unwired: 7 in, 1 out]
          }
          event "Record EOC": Value Change {
            n73 = event-data() -> ()  [unwired: 1 in, 1 out]
            n74 = call-poly <vilib>:"Delacor_lib_QMH_Enqueue Message (poly).vi"("Priority Message? (F)"=TRUE, "Message"="Record Action EOC", "Message Queue in"=w293) -> ("error out"=w292:errorcluster)  [unwired: 7 in, 1 out]
          }
          event Key Down {
            n75 = event-data() -> ("Char"=w297:i16, "VKey"=w300:T14)  [unwired: 1 in]
            n76 = Equal?(x=w300, y=eventvkey."ASCII" ("VKey")) -> (x = y?=w298:bool)
            n77 = case shown="True" w298 {
              tunnel: w297 -> [_ w303]
              tunnel: w296 -> [_ w302]
              tunnel: [_ w301] -> w295
              frame False {
              }
              frame True {
                n78 = case shown="48..57, 65..90, 97..122" w303 {
                  selector: w303 -> [_ w305]
                  tunnel: w302 -> [_ w306]
                  tunnel: [_ w304] -> w301
                  frame 0, Default {
                  }
                  frame 48..57, 65..90, 97..122 {
                    n79 = call-poly <vilib>:"Delacor_lib_QMH_Enqueue Message (poly).vi"("Message Data"=w305, "Message"="Trigger Action", "Message Queue in"=w306) -> ("error out"=w304:errorcluster)  [unwired: 7 in, 1 out]
                  }
                }
              }
            }
          }
          event "Data 1", "Data 2", "Data 3", "Data 4", "Data 5", "Data 6", "Data 7", "Data 8", "Data 9", "Data 10", "Data 11", "Data 12", "Data 13", "Data 14", "Data 15", "Data 16", "Single Chart": Mouse Down {
            n80 = event-data() -> ("CtlRef"=w309:refnum<vi>, "Button"=w311:u16)  [unwired: 1 in, 1 out]
            n81 = case shown="1" w311 {
              tunnel: [_ w315] -> w310
              tunnel: w309 -> [_ w314]
              tunnel: w308 -> [_ w312]
              frame 0, Default {
              }
              frame 1 {
                n82 = property class="WFChart (strict)"(reference=w314) -> ("Label.Text"=w313:string)  [unwired: 1 in, 2 out]
                n83 = call-poly <vilib>:"Delacor_lib_QMH_Enqueue Message (poly).vi"("Message Data"=w313, "Message"="Graph Mouse Action", "Message Queue in"=w312) -> ("error out"=w315:errorcluster)  [unwired: 7 in, 1 out]
              }
            }
          }
          event "Stop": Value Change {
            # "Send \"Go to IDLE\" also"
            n84 = event-data() -> ()  [unwired: 1 in, 1 out]
            n85 = local read "Data Select"() -> (w317:string)
            n86 = call-poly <vilib>:"Delacor_lib_QMH_Enqueue Message (poly).vi"("Message Data"=w317, "Message"="Stop", "Message Queue in"=w318) -> ("error out"=w320:errorcluster)  [unwired: 7 in, 1 out]
          }
          event "Stop CNV": Value Change {
            n87 = event-data() -> ()  [unwired: 1 in, 1 out]
            n88 = call-poly <vilib>:"Delacor_lib_QMH_Enqueue Message (poly).vi"("Message"="Stop CNV Demo", "Message Queue in"=w321) -> ("error out"=w323:errorcluster)  [unwired: 8 in, 1 out]
          }
          event "Stop EOC": Value Change {
            n89 = event-data() -> ()  [unwired: 1 in, 1 out]
            n90 = call-poly <vilib>:"Delacor_lib_QMH_Enqueue Message (poly).vi"("Message"="Stop EOC Demo", "Message Queue in"=w324) -> ("error out"=w326:errorcluster)  [unwired: 8 in, 1 out]
          }
          event "Settings": Value Change {
            n91 = event-data() -> ()  [unwired: 1 in, 1 out]
            n92 = call "Show Panel.vi"() -> ("error out"=w327:errorcluster)  [unwired: 11 in]
          }
          event Menu Selection (User) {
            n93 = event-data() -> ("ItemTag"=w330:string)  [unwired: 1 in]
            n94 = case shown="\"Impedance\"" w330 {
              selector: w330 -> [_ _ _ _ _ w338 w343 w346 w350 _ _ _ _ _ _ _ _ _ _ _ _ _ _]
              tunnel: w329 -> [_ _ _ _ w335 w340 w344 w348 w352 w356 w360 w364 w368 w371 w374 w377 w380 w383 w386 w389 w392 w395 w398]
              tunnel: [_ w331 w332 w333 w334 w339 w342 w347 w351 w355 w359 w363 w367 w370 w373 w376 w379 w382 w385 w388 w391 w394 w397] -> w328
              frame "False", Default {
              }
              frame "Launch Settings" {
                n95 = call "Show Panel.vi"() -> ("error out"=w331:errorcluster)  [unwired: 11 in]
              }
              frame "About" {
                n96 = call "Menu -- About Display Box.vi"() -> ("error out"=w332:errorcluster)  [unwired: 11 in]
              }
              frame "Download MATLAB files" {
                n97 = call "Wake-Up Copy MATLAB files.vi"() -> ("error out"=w333:errorcluster)  [unwired: 11 in]
              }
              frame "Exit" {
                n98 = call-poly <vilib>:"Delacor_lib_QMH_Enqueue Message (poly).vi"("Priority Message? (F)"=TRUE, "Message"="Exit", "Message Queue in"=w335) -> ("error out"=w334:errorcluster)  [unwired: 7 in, 1 out]
              }
              frame "Graph" {
                n99 = call-poly <vilib>:"Delacor_lib_QMH_Enqueue Message (poly).vi"("Message Data"=w338, "Message"="Set Display", "Message Queue in"=w340) -> ("error out"=w339:errorcluster)  [unwired: 7 in, 1 out]
              }
              frame "Impedance" {
                n100 = call-poly <vilib>:"Delacor_lib_QMH_Enqueue Message (poly).vi"("Message Data"=w343, "Message"="Set Display", "Message Queue in"=w344) -> ("error out"=w342:errorcluster)  [unwired: 7 in, 1 out]
              }
              frame "CNV Demo" {
                n101 = call-poly <vilib>:"Delacor_lib_QMH_Enqueue Message (poly).vi"("Message Data"=w346, "Message"="Set Display", "Message Queue in"=w348) -> ("error out"=w347:errorcluster)  [unwired: 7 in, 1 out]
              }
              frame "Eyes OC Demo" {
                n102 = call-poly <vilib>:"Delacor_lib_QMH_Enqueue Message (poly).vi"("Message Data"=w350, "Message"="Set Display", "Message Queue in"=w352) -> ("error out"=w351:errorcluster)  [unwired: 7 in, 1 out]
              }
              frame "Start Acquiring" {
                n103 = local read "Data Select"() -> (w354:string)
                n104 = call-poly <vilib>:"Delacor_lib_QMH_Enqueue Message (poly).vi"("Message Data"=w354, "Message"="Start", "Message Queue in"=w356) -> ("error out"=w355:errorcluster)  [unwired: 7 in, 1 out]
              }
              frame "Stop Acquiring" {
                n105 = local read "Data Select"() -> (w358:string)
                n106 = call-poly <vilib>:"Delacor_lib_QMH_Enqueue Message (poly).vi"("Message Data"=w358, "Message"="Stop", "Message Queue in"=w360) -> ("error out"=w359:errorcluster)  [unwired: 7 in, 1 out]
              }
              frame "Start Logging" {
                n107 = call-poly <vilib>:"Delacor_lib_QMH_Enqueue Message (poly).vi"("Priority Message? (F)"=TRUE, "Message"="Record Action", "Message Queue in"=w364) -> ("error out"=w363:errorcluster)  [unwired: 7 in, 1 out]
              }
              frame "Stop Logging" {
                n108 = call-poly <vilib>:"Delacor_lib_QMH_Enqueue Message (poly).vi"("Priority Message? (F)"=TRUE, "Message"="Record Action", "Message Queue in"=w368) -> ("error out"=w367:errorcluster)  [unwired: 7 in, 1 out]
              }
              frame "Start Impedance" {
                n109 = call-poly <vilib>:"Delacor_lib_QMH_Enqueue Message (poly).vi"("Message"="Impedance Start", "Message Queue in"=w371) -> ("error out"=w370:errorcluster)  [unwired: 8 in, 1 out]
              }
              frame "Stop Impedance" {
                n110 = call-poly <vilib>:"Delacor_lib_QMH_Enqueue Message (poly).vi"("Message"="Impedance Stop", "Message Queue in"=w374) -> ("error out"=w373:errorcluster)  [unwired: 8 in, 1 out]
              }
              frame "Start CNV Acquiring" {
                n111 = call-poly <vilib>:"Delacor_lib_QMH_Enqueue Message (poly).vi"("Message"="Start CNV Demo", "Message Queue in"=w377) -> ("error out"=w376:errorcluster)  [unwired: 8 in, 1 out]
              }
              frame "Stop CNV Acquiring" {
                n112 = call-poly <vilib>:"Delacor_lib_QMH_Enqueue Message (poly).vi"("Message"="Stop CNV Demo", "Message Queue in"=w380) -> ("error out"=w379:errorcluster)  [unwired: 8 in, 1 out]
              }
              frame "Start CNV Logging" {
                n113 = call-poly <vilib>:"Delacor_lib_QMH_Enqueue Message (poly).vi"("Message"="Record Action CNV", "Message Queue in"=w383) -> ("error out"=w382:errorcluster)  [unwired: 8 in, 1 out]
              }
              frame "Stop CNV Logging" {
                n114 = call-poly <vilib>:"Delacor_lib_QMH_Enqueue Message (poly).vi"("Message"="Record Action CNV", "Message Queue in"=w386) -> ("error out"=w385:errorcluster)  [unwired: 8 in, 1 out]
              }
              frame "Start EOC Acquiring" {
                n115 = call-poly <vilib>:"Delacor_lib_QMH_Enqueue Message (poly).vi"("Message"="Start EOC Demo", "Message Queue in"=w389) -> ("error out"=w388:errorcluster)  [unwired: 8 in, 1 out]
              }
              frame "Stop EOC Acquiring" {
                n116 = call-poly <vilib>:"Delacor_lib_QMH_Enqueue Message (poly).vi"("Message"="Stop EOC Demo", "Message Queue in"=w392) -> ("error out"=w391:errorcluster)  [unwired: 8 in, 1 out]
              }
              frame "Start EOC Logging" {
                n117 = call-poly <vilib>:"Delacor_lib_QMH_Enqueue Message (poly).vi"("Message"="Record Action EOC", "Message Queue in"=w395) -> ("error out"=w394:errorcluster)  [unwired: 8 in, 1 out]
              }
              frame "Stop EOC Logging" {
                n118 = call-poly <vilib>:"Delacor_lib_QMH_Enqueue Message (poly).vi"("Message"="Record Action EOC", "Message Queue in"=w398) -> ("error out"=w397:errorcluster)  [unwired: 8 in, 1 out]
              }
            }
          }
          event "Calibrate": Value Change {
            n119 = event-data() -> ()  [unwired: 1 in, 1 out]
            n120 = call "Calibrate DAQ.vi"() -> ("error out"=w400:errorcluster)  [unwired: 11 in]
          }
          event User Event {
            w402 = TRUE ("Settings Editor Running?")
            n121 = event-data() -> ()  [unwired: 1 in, 1 out]
            n122 = local read "Acquisition Running?"() -> (w404:bool)
            n123 = local read "Logger Running?"() -> (w403:bool)
            n124 = call "Is UI Ready.vi"("Logger Running?"=w403, "Acquisition Running?"=w404, "Settings Editor Running?"=w402) -> ("Status"=w401:string)  [unwired: 8 in]
            n125 = local write "Status"(w401) -> ()
            "Settings Editor Running?" <- w402
          }
          event User Event {
            n126 = event-data() -> ("Settings"=w407:T26, "error"=w408:errorcluster)  [unwired: 1 in, 4 out]
            n127 = case shown="No Error" w408 {
              tunnel: w407 -> [w409 _]
              tunnel: w406 -> [w410 _]
              tunnel: [w411 _] -> w405
              frame No Error {
                n128 = call-poly <vilib>:"Delacor_lib_QMH_Enqueue Message (poly).vi"("Message Data"=w409, "Message"="Settings Updated", "Message Queue in"=w410) -> ("error out"=w411:errorcluster)  [unwired: 7 in, 1 out]
              }
              frame Error {
              }
            }
          }
          event User Event {
            w415 = TRUE ("Acquisition Running?")
            n129 = event-data() -> ()  [unwired: 1 in, 1 out]
            n130 = local read "Settings Editor Running?"() -> (w414:bool)
            n131 = local read "Logger Running?"() -> (w413:bool)
            n132 = call "Is UI Ready.vi"("Logger Running?"=w413, "Acquisition Running?"=w415, "Settings Editor Running?"=w414) -> ("Status"=w416:string)  [unwired: 8 in]
            n133 = local write "Status"(w416) -> ()
            "Acquisition Running?" <- w415
          }
          event User Event {
            w420 = TRUE ("Logger Running?")
            n134 = event-data() -> ()  [unwired: 1 in, 1 out]
            n135 = local read "Settings Editor Running?"() -> (w419:bool)
            n136 = local read "Acquisition Running?"() -> (w418:bool)
            n137 = call "Is UI Ready.vi"("Logger Running?"=w420, "Acquisition Running?"=w418, "Settings Editor Running?"=w419) -> ("Status"=w421:string)  [unwired: 8 in]
            n138 = local write "Status"(w421) -> ()
            "Logger Running?" <- w420
          }
          event User Event {
            n139 = event-data() -> ("Status"=w422:string)  [unwired: 1 in]
            "Status" <- w422
            n140 = call "Status Updated.vi"("Status"=w422) -> ()  [unwired: 10 in, 1 out]
          }
          event User Event {
            n141 = event-data() -> ("Error"=w427:errorcluster, "Module Name"=w425:string)  [unwired: 1 in, 1 out]
            n142 = Unbundle By Name(w427) -> ("code"=w426:i32)
            n143 = Format Into String(format string="Error %d at %s", w426, w425) -> (resulting string=w424:string)  [unwired: 2 in, 1 out]
            n144 = local write "Status"(w424) -> ()
          }
          event User Event {
            n145 = event-data() -> ()  [unwired: 1 in, 1 out]
            n146 = call-poly <vilib>:"Delacor_lib_QMH_Enqueue Message (poly).vi"("Message"="Acquisition Started Interlocks", "Message Queue in"=w429) -> ()  [unwired: 8 in, 2 out]
          }
          event User Event {
            n147 = event-data() -> ()  [unwired: 1 in, 1 out]
          }
          event User Event {
            n148 = event-data() -> ("WiBCI16T Data out"=w432:T21, "En MAP"=w431:u16)  [unwired: 1 in]
            n149 = Bundle("WiBCI16T Data out"=w432, "En MAP"=w431) -> (w430:cluster{"WiBCI16T Data out":T21, "En MAP":u16})  [unwired: 1 in]
            n150 = call-poly <vilib>:"Delacor_lib_QMH_Enqueue Message (poly).vi"("Message Data"=w430, "Message"="Update_Display", "Message Queue in"=w434) -> ("error out"=w433:errorcluster)  [unwired: 7 in, 1 out]
          }
          event User Event {
            n151 = event-data() -> ("WiBCI16T Data"=w438:T21, "En Map"=w437:u16)  [unwired: 1 in]
            n152 = Bundle("WiBCI16T Data"=w438, "En Map"=w437) -> (w436:cluster{"WiBCI16T Data":T21, "En Map":u16})  [unwired: 1 in]
            n153 = call-poly <vilib>:"Delacor_lib_QMH_Enqueue Message (poly).vi"("Message Data"=w436, "Message"="Update_Display", "Message Queue in"=w440) -> ("error out"=w439:errorcluster)  [unwired: 7 in, 1 out]
          }
          event User Event {
            n154 = event-data() -> ("WiBCI16T Data"=w444:T21, "En MAP"=w443:u16)  [unwired: 1 in]
            n155 = Bundle("WiBCI16T Data"=w444, "En MAP"=w443) -> (w442:cluster{"WiBCI16T Data":T21, "En MAP":u16})  [unwired: 1 in]
            n156 = call-poly <vilib>:"Delacor_lib_QMH_Enqueue Message (poly).vi"("Message Data"=w442, "Message"="Update_IMP_Display", "Message Queue in"=w446) -> ("error out"=w445:errorcluster)  [unwired: 7 in, 1 out]
          }
          event User Event {
            n157 = event-data() -> ("WiBCI16T Data"=w450:T21, "En MAP"=w449:u16)  [unwired: 1 in]
            n158 = Bundle("WiBCI16T Data"=w450, "En MAP"=w449) -> (w448:cluster{"WiBCI16T Data":T21, "En MAP":u16})  [unwired: 1 in]
            n159 = call-poly <vilib>:"Delacor_lib_QMH_Enqueue Message (poly).vi"("Message Data"=w448, "Message"="Update_CNV_Display", "Message Queue in"=w452) -> ("error out"=w451:errorcluster)  [unwired: 7 in, 1 out]
          }
          event User Event {
            n160 = event-data() -> ("WiBCI16T Data"=w456:T21, "En MAP"=w455:u16)  [unwired: 1 in]
            n161 = Bundle("WiBCI16T Data"=w456, "En MAP"=w455) -> (w454:cluster{"WiBCI16T Data":T21, "En MAP":u16})  [unwired: 1 in]
            n162 = call-poly <vilib>:"Delacor_lib_QMH_Enqueue Message (poly).vi"("Message Data"=w454, "Message"="Update_EOC_Display", "Message Queue in"=w458) -> ("error out"=w457:errorcluster)  [unwired: 7 in, 1 out]
          }
          event User Event {
            n163 = event-data() -> ()  [unwired: 1 in, 1 out]
            "Calibrated?" <- TRUE ("Calibrated?")
          }
          event "About DQMH": Value Change {
            # "Display the About DQMH box"
            n164 = event-data() -> ()  [unwired: 1 in, 1 out]
            n165 = call <vilib>:"DQMH_About Box.vi"() -> ("error out"=w461:errorcluster)  [unwired: 11 in]
          }
          event User Event {
            # "Another Module called the \"STOP_GUI\" API Method."
            n166 = event-data() -> ("Message for the Request"=w463:string)  [unwired: 1 in]
            n167 = Bundle(cluster=T15 {"Message for the Request"=""} ("STOP_GUI Argument"), "Message for the Request"=w463) -> (w464:T15)
            n168 = call-poly <vilib>:"Delacor_lib_QMH_Enqueue Message (poly).vi"("Message Data"=w464, "Message"="STOP_GUI", "Message Queue in"=w467) -> ("error out"=w462:errorcluster)  [unwired: 7 in, 1 out]
          }
          event User Event {
            # "Another Module called the \"Clear All Charts\" API Method."
            n169 = event-data() -> ("Boolean"=w470:bool)  [unwired: 1 in]
            n170 = Bundle(cluster=T16 {"Boolean"=FALSE} ("Clear All Charts Argument"), "Boolean"=w470) -> (w471:T16)
            n171 = call-poly <vilib>:"Delacor_lib_QMH_Enqueue Message (poly).vi"("Priority Message? (F)"=TRUE, "Message Data"=w471, "Message"="Clear All Charts", "Message Queue in"=w474) -> ("error out"=w469:errorcluster)  [unwired: 6 in, 1 out]
          }
          event User Event {
            # "Another Module called the \"Update Data Status UI\" API Method."
            n172 = event-data() -> ("status"=w477:bool)  [unwired: 1 in]
            n173 = Bundle(cluster=T17 {"status"=FALSE} ("Update Data Status UI Argument"), "status"=w477) -> (w476:T17)
            n174 = Unbundle By Name(w476) -> ("status"=w475:bool)
            n175 = local write "Data Status"(w475) -> ()
          }
          event User Event {
            # "Another Module called the \"Update Packet Loss (%)\" API Method."
            n176 = event-data() -> ("Paket Loss"=w480:dbl)  [unwired: 1 in]
            n177 = Bundle(cluster=T18 {"Paket Loss"=0.0} ("Update Packet Loss (%) Argument"), "Paket Loss"=w480) -> (w481:T18)
            n178 = call-poly <vilib>:"Delacor_lib_QMH_Enqueue Message (poly).vi"("Message Data"=w481, "Message"="Update Packet Loss (%)", "Message Queue in"=w484) -> ("error out"=w479:errorcluster)  [unwired: 7 in, 1 out]
          }
        }
        n179 = call-dynamic "Delacor_lib_QMH_Error Handler - Event Handling Loop.vi"("error in"=w226, "Message Queue in"=w220) -> ("dup error in"=w225:errorcluster)  [unwired: 8 in, 1 out]
      }
      n180 = while {
        tunnel: w70 -> [w493]
        shift-right: [w496] -> _
        shift-left: T9 {"Status"="", "Measurement UI Controls"={"Start Ref"=refnum, "Stop Ref"=refnum, "Settings Ref"=refnum, "Status Ref"=refnum, "Data Ref"=refnum, "Rec Ref"=refnum, "Soft Trig"=refnum, "Imp Start Ref"=refnum, "Imp Stop Ref"=refnum, "CNV Start Ref"=refnum, "CNV Stop Ref"=refnum, "CNV Rec"=refnum, "Recording State CNV"=refnum, "EOC Start Ref"=refnum, "EOC Stop Ref"=refnum, "EOC Rec Ref"=refnum, "CNV Rec state"=refnum, "Recording State EOC"=refnum}, "Recording State"=FALSE, "Impedance"={"Ch 1"=0.0, "Ch 2"=0.0, "Ch 3"=0.0, "Ch 4"=0.0, "Ch 5"=0.0, "Ch 6"=0.0, "Ch 7"=0.0, "Ch 8"=0.0, "Ch 9"=0.0, "Ch 10"=0.0, "Ch 11"=0.0, "Ch 12"=0.0, "Ch 13"=0.0, "Ch 14"=0.0, "Ch 15"=0.0, "Ch 16"=0.0}, "menu reference "=refnum, "Acq State"=enum."RUNNING", "En/Dis Trig"=refnum, "Soft Trigger En?"=FALSE, "Display  cnt"=0, "UI Page"=refnum, "CNV Demo Data"={"Rebuild Vector"=[], "CNV Buffer Action"=enum."Stop Buffer Fill", "Index of R.Array"=0, "Run Sum CNV"=[], "CNV Iter"=0}, "EOC Demo Data"={"Running Buffer"=[], "Index of R.Buffer"=0}, "Measurement UI Displays"={"Graph 1"=refnum, "Graph 2"=refnum, "Graph 3"=refnum, "Graph 4"=refnum, "Graph 5"=refnum, "Graph 6"=refnum, "Graph 7"=refnum, "Graph 8"=refnum, "Graph 9"=refnum, "Graph 10"=refnum, "Graph 11"=refnum, "Graph 12"=refnum, "Graph 13"=refnum, "Graph 14"=refnum, "Graph 15"=refnum, "Graph 16"=refnum, "Battery 2"=refnum, "Data Trig"=refnum, "Data Connection Status"=refnum, "Graph Sel"=0, "En MAP"=0, "Single Chart"=refnum, "G.Ch Name 1"=refnum, "G.Ch Name 2"=refnum, "G.Ch Name 3"=refnum, "G.Ch Name 4"=refnum, "G.Ch Name 5"=refnum, "G.Ch Name 6"=refnum, "G.Ch Name 7"=refnum, "G.Ch Name 8"=refnum, "G.Ch Name 9"=refnum, "G.Ch Name 10"=refnum, "G.Ch Name 11"=refnum, "G.Ch Name 12"=refnum, "G.Ch Name 13"=refnum, "G.Ch Name 14"=refnum, "G.Ch Name 15"=refnum, "G.Ch Name 16"=refnum, "imp mode sel"=refnum}, "Recording State CNV"=FALSE, "Recording State EOC"=FALSE, "LSL En?"=FALSE, "LSL Listeners"=refnum, "Imp Mode"=FALSE} ("Data Cluster") -> [w497]
        tunnel: w74 -> [w500]
        tunnel: [w498] -> w76
        tunnel: w69 -> [w491]
        tunnel: w68 -> [w490]
        tunnel: w58 -> [w488]
        tunnel: w57 -> [w487]
        tunnel: w56 -> [w486]
        tunnel: w55 -> [w485]
        stop <- w495 stop-if-true
        # "Message Handling Loop"
        n181 = call-dynamic "Delacor_lib_QMH_Dequeue Message.vi"("error in"=w500, "Message Queue in"=w493) -> ("error out"=w499:errorcluster, "Message Data"=w494:variant, "Message"=w489:string, "Message Queue out"=w492:refnum<class "Delacor_lib_QMH_Message Queue.lvclass">)  [unwired: 6 in]
        n182 = case "DQMH_MESSAGE_CASES" shown="\"Update_IMP_Display\"" w489 {
          selector: w489 -> [_ _ _ _ _ _ _ _ _ _ _ _ _ _ _ _ _ _ _ _ _ _ _ _ _ _ _ _ _ _ _ _ _ _ _ _ _ _ _ _ _ _ _ _ _ w1623]
          tunnel: w492 -> [w556 _ w629 w662 _ _ _ _ _ _ _ _ _ _ _ _ w920 w950 w961 _ w980 _ _ _ _ _ _ _ _ _ _ _ w1410 _ w1447 _ w1475 w1487 w1496 _ _ w1540 _ w1556 w1584 _]
          tunnel: w499 -> [w563 w593 w630 w658 w711 w737 w761 w778 w795 w809 w823 w837 w851 w853 w863 w881 w925 w946 w957 w968 w993 w1007 w1151 w1256 w1319 w1378 w1385 w1388 w1395 w1400 w1405 w1406 w1418 w1441 w1443 w1455 w1468 w1483 w1492 w1505 w1521 w1546 w1553 w1563 w1587 w1625]
          tunnel: [w555 w593 w606 w664 w710 w736 w760 w777 w795 w809 w823 w837 w845 w853 w863 w877 w918 w951 w962 w968 w979 w1005 w1149 w1254 w1311 w1378 w1383 w1387 w1394 w1399 w1404 w1409 w1420 w1432 w1450 w1460 w1478 w1490 w1499 w1507 w1515 w1538 w1553 w1559 w1578 w1626] -> w501
          tunnel: w497 -> [w569 w592 w628 w653 w713 w727 w750 w775 w793 w807 w822 w836 w848 w854 w864 w874 w932 w945 w956 w969 w992 w994 w1142 w1252 w1314 w1357 w1384 w1386 w1393 w1398 w1403 w1408 w1419 w1433 w1446 w1459 w1474 w1486 w1495 w1506 w1518 w1541 w1552 w1558 w1576 w1624]
          tunnel: [w520 w592 w628 w656 w712 w726 w749 w775 w793 w807 w822 w836 w848 w854 w864 w873 w931 w944 w955 w969 w992 w995 w1144 w1251 w1312 w1377 w1384 w1386 w1392 w1397 w1402 w1408 w1419 w1430 w1444 w1457 w1472 w1484 w1493 w1506 w1518 w1543 w1552 w1558 w1576 w1624] -> w496
          tunnel: [_ _ _ _ _ _ _ _ _ _ _ _ _ _ _ _ _ _ _ _ _ _ _ _ _ _ _ _ _ _ _ _ _ _ _ _ _ _ _ _ _ _ _ _ w1574 _] -> w495
          tunnel: w494 -> [_ _ _ w668 _ _ _ _ _ _ _ _ w850 _ _ _ w924 _ _ _ w991 w1006 w1150 w1257 w1320 _ w1382 _ _ _ _ _ w1417 w1440 _ w1452 _ _ _ w1504 w1520 w1545 _ w1557 w1583 _]
          tunnel: w491 -> [w581 _ _ _ _ _ _ _ _ _ _ _ _ _ _ _ _ _ _ _ _ _ _ _ _ _ _ _ _ _ _ _ _ _ _ _ _ _ _ _ _ _ _ w1555 w1579 _]
          tunnel: w490 -> [_ _ _ _ _ _ _ _ _ _ _ _ _ _ _ _ _ _ _ _ _ _ _ _ _ _ _ _ _ _ _ _ _ _ _ _ _ _ _ _ _ _ _ _ w1577 _]
          tunnel: w488 -> [_ _ _ _ _ _ _ _ _ _ _ _ _ _ _ _ _ _ _ _ _ _ _ _ _ _ _ _ _ _ _ _ _ _ _ _ _ _ _ _ _ _ _ _ w1573 _]
          tunnel: w487 -> [_ _ _ _ _ _ _ _ _ _ _ _ _ _ _ _ _ _ _ _ _ _ _ _ _ _ _ _ _ _ _ _ _ _ _ _ _ _ _ _ _ _ _ _ w1572 _]
          tunnel: w486 -> [_ _ _ _ _ _ _ _ _ _ _ _ _ _ _ _ _ _ _ _ _ _ _ _ _ _ _ _ _ _ _ _ _ _ _ _ _ _ _ _ _ _ _ _ w1571 _]
          tunnel: w485 -> [_ _ _ _ _ _ _ _ _ _ _ _ _ _ _ _ _ _ _ _ _ _ _ _ _ _ _ _ _ _ _ _ _ _ _ _ _ _ _ _ _ _ _ _ w1570 _]
          frame "Initialize" {
            w527 = FALSE ("Recording State")
            w577 = "Initial Message" ("Initial Message")
            # "Graph Displays"
            # "Channel Names Display"
            # "Initialize - Any operation that needs to be done before the module can receive messages. Synchronize Caller Events.vi will inform Start Module.vi that the module has launched and is ready to receive messages. Module Did Init.vi will broadcast that the module initialized."
            n183 = flat-sequence {
              tunnel: w569 -> [w591]
              tunnel: [w591] -> w568
              frame #0 {
                n184 = invoke on="Record Button" class="Bool (strict)" method="Reinit To Default"() -> ()  [unwired: 3 in, 3 out]
              }
            }
            n185 = Current VI's Menubar() -> (w564:refnum<k9>)
            n186 = call "Synchronize Caller Events.vi"("error in (no error)"=w563, "Singleton Module Admin in"=w581) -> ("error out"=w588:errorcluster, "Singleton Module Admin out"=w578:refnum<class "Delacor_lib_QMH_Module Admin.lvclass">)  [unwired: 8 in]
            n187 = call "Set Init Menu.vi"("error in (no error)"=w563, "Menu in"=w564) -> ("Menu out"=w562:refnum<k9>)  [unwired: 9 in]
            n188 = property on="Property Node" class="Module Admin"(reference=w578) -> ("Accessors:External Launch"=w585:bool)  [unwired: 1 in, 2 out]
            n189 = local write "Calibrated?"(FALSE ("Calibrated?")) -> ()
            n190 = control-ref of="Data 1"() -> (w546:refnum<vi>)
            n191 = control-ref of="Data 2"() -> (w545:refnum<vi>)
            n192 = control-ref of="Data 3"() -> (w544:refnum<vi>)
            n193 = control-ref of="Data 4"() -> (w543:refnum<vi>)
            n194 = control-ref of="Data 5"() -> (w542:refnum<vi>)
            n195 = control-ref of="Data 6"() -> (w541:refnum<vi>)
            n196 = control-ref of="Data 7"() -> (w540:refnum<vi>)
            n197 = control-ref of="Data 8"() -> (w539:refnum<vi>)
            n198 = control-ref of="Data 9"() -> (w538:refnum<vi>)
            n199 = control-ref of="imp mode"() -> (w503:refnum<vi>)
            n200 = control-ref of="Single Chart"() -> (w522:refnum<vi>)
            n201 = control-ref of="Data 10"() -> (w537:refnum<vi>)
            n202 = control-ref of="Data 11"() -> (w536:refnum<vi>)
            n203 = control-ref of="Data 12"() -> (w535:refnum<vi>)
            n204 = control-ref of="Data 13"() -> (w534:refnum<vi>)
            n205 = control-ref of="Data 14"() -> (w533:refnum<vi>)
            n206 = control-ref of="Data 15"() -> (w532:refnum<vi>)
            n207 = control-ref of="Data 16"() -> (w531:refnum<vi>)
            n208 = local write "Status"(w577) -> ()
            n209 = control-ref of="Start EOC"() -> (w549:refnum<vi>)
            n210 = control-ref of="Stop EOC"() -> (w548:refnum<vi>)
            n211 = control-ref of="Record EOC"() -> (w547:refnum<vi>)
            n212 = control-ref of="LSL Listeners"() -> (w525:refnum<vi>)
            n213 = control-ref of="Start CNV"() -> (w552:refnum<vi>)
            n214 = control-ref of="Stop CNV"() -> (w551:refnum<vi>)
            n215 = control-ref of="Record CNV"() -> (w550:refnum<vi>)
            n216 = Select(t=T19."Hidden" ("State"), s=w585, f=T19."Standard" ("State")) -> (s? t:f=w582:T19)
            n217 = control-ref of="UI Page"() -> (w553:refnum<vi>)
            n218 = control-ref of="Start"() -> (w576:refnum<vi>)
            n219 = control-ref of="Stop"() -> (w575:refnum<vi>)
            n220 = control-ref of="Settings"() -> (w574:refnum<vi>)
            n221 = control-ref of="Record Button"() -> (w570:refnum<vi>)
            n222 = control-ref of="Start Imped"() -> (w567:refnum<vi>)
            n223 = control-ref of="Stop Imped"() -> (w566:refnum<vi>)
            n224 = control-ref of="Status"() -> (w573:refnum<vi>)
            n225 = property on="Property Node" class="VI"("Front Panel.Title"="The Application" ("Front Panel Window:Title")) -> (reference out=w587:refnum<vi>, error out=w590:errorcluster)  [unwired: 2 in]
            n226 = control-ref of="Data Trig"() -> (w530:refnum<vi>)
            n227 = control-ref of="En/Dis Trig"() -> (w560:refnum<vi>)
            n228 = call "Module Name--constant.vi"() -> ("Module Name"=w579:string)  [unwired: 11 in]
            n229 = control-ref of="Data Status"() -> (w528:refnum<vi>)
            n230 = invoke on="Invoke Node" class="VI" method="FP.Open"(reference=w587, error in=w590, "State"=w582) -> (reference out=w586:refnum<vi>, error out=w589:errorcluster)  [unwired: 2 in, 3 out]
            n231 = control-ref of="Battery"() -> (w529:refnum<vi>)
            n232 = call "Module Did Init.vi"("error in (no error)"=w588, "Initialized?"=TRUE, "Origin"=w579) -> ("error out"=w571:errorcluster)  [unwired: 8 in]
            n233 = Bundle By Name(cluster=w568, "Measurement UI Controls.Start Ref"=w576, "Measurement UI Controls.Stop Ref"=w575, "Measurement UI Controls.Settings Ref"=w574, "Measurement UI Controls.Status Ref"=w573, "Status"=w577, "Recording State"=w527, "Recording State CNV"=w527, "Recording State EOC"=w527, "Measurement UI Controls.Rec Ref"=w570, "Measurement UI Controls.Imp Start Ref"=w567, "Measurement UI Controls.Imp Stop Ref"=w566, "menu reference"=w562, "UI Page"=w553, "Acq State"=Acquisition_State."IDLE" ("Enum"), "En/Dis Trig"=w560, "Soft Trigger En?"=FALSE, "Display  cnt"=u8 0 ("Display Update Counter"), "Measurement UI Controls.CNV Start Ref"=w552, "Measurement UI Controls.CNV Stop Ref"=w551, "Measurement UI Controls.CNV Rec"=w550, "Measurement UI Controls.EOC Start Ref"=w549, "Measurement UI Controls.EOC Stop Ref"=w548, "Measurement UI Controls.EOC Rec Ref"=w547, "Measurement UI Displays.Graph 1"=w546, "Measurement UI Displays.Graph 2"=w545, "Measurement UI Displays.Graph 3"=w544, "Measurement UI Displays.Graph 4"=w543, "Measurement UI Displays.Graph 5"=w542, "Measurement UI Displays.Graph 6"=w541, "Measurement UI Displays.Graph 7"=w540, "Measurement UI Displays.Graph 8"=w539, "Measurement UI Displays.Graph 9"=w538, "Measurement UI Displays.Graph 10"=w537, "Measurement UI Displays.Graph 11"=w536, "Measurement UI Displays.Graph 12"=w535, "Measurement UI Displays.Graph 13"=w534, "Measurement UI Displays.Graph 14"=w533, "Measurement UI Displays.Graph 15"=w532, "Measurement UI Displays.Graph 16"=w531, "Measurement UI Displays.Single Chart"=w522, "Measurement UI Displays.Data Trig"=w530, "Measurement UI Displays.Battery 2"=w529, "Measurement UI Displays.Data Connection Status"=w528, "LSL En?"=FALSE, "LSL Listeners"=w525, "Measurement UI Displays.Graph Sel"=u8 0, "Measurement UI Displays.En MAP"=u16 65535, "Measurement UI Displays.imp mode sel"=w503, "Imp Mode"=FALSE) -> (w521:T9)
            n234 = invoke on="Invoke Node" class="VI" method="FP.Center"(reference=w586, error in=w589) -> ()  [unwired: 1 in, 3 out]
            n235 = control-ref of="G.Ch Name 1"() -> (w519:refnum<vi>)
            n236 = control-ref of="G.Ch Name 2"() -> (w518:refnum<vi>)
            n237 = control-ref of="G.Ch Name 3"() -> (w517:refnum<vi>)
            n238 = control-ref of="G.Ch Name 4"() -> (w516:refnum<vi>)
            n239 = control-ref of="G.Ch Name 5"() -> (w515:refnum<vi>)
            n240 = control-ref of="G.Ch Name 6"() -> (w514:refnum<vi>)
            n241 = control-ref of="G.Ch Name 7"() -> (w513:refnum<vi>)
            n242 = control-ref of="G.Ch Name 8"() -> (w512:refnum<vi>)
            n243 = control-ref of="G.Ch Name 9"() -> (w511:refnum<vi>)
            n244 = Merge Errors(w571) -> (w557:errorcluster)
            n245 = control-ref of="G.Ch Name 10"() -> (w510:refnum<vi>)
            n246 = control-ref of="G.Ch Name 11"() -> (w509:refnum<vi>)
            n247 = control-ref of="G.Ch Name 12"() -> (w508:refnum<vi>)
            n248 = control-ref of="G.Ch Name 13"() -> (w507:refnum<vi>)
            n249 = control-ref of="G.Ch Name 14"() -> (w506:refnum<vi>)
            n250 = control-ref of="G.Ch Name 15"() -> (w505:refnum<vi>)
            n251 = control-ref of="G.Ch Name 16"() -> (w504:refnum<vi>)
            n252 = Bundle By Name(cluster=w521, "Measurement UI Displays.G.Ch Name 1"=w519, "Measurement UI Displays.G.Ch Name 2"=w518, "Measurement UI Displays.G.Ch Name 3"=w517, "Measurement UI Displays.G.Ch Name 4"=w516, "Measurement UI Displays.G.Ch Name 5"=w515, "Measurement UI Displays.G.Ch Name 6"=w514, "Measurement UI Displays.G.Ch Name 7"=w513, "Measurement UI Displays.G.Ch Name 8"=w512, "Measurement UI Displays.G.Ch Name 9"=w511, "Measurement UI Displays.G.Ch Name 10"=w510, "Measurement UI Displays.G.Ch Name 11"=w509, "Measurement UI Displays.G.Ch Name 12"=w508, "Measurement UI Displays.G.Ch Name 13"=w507, "Measurement UI Displays.G.Ch Name 14"=w506, "Measurement UI Displays.G.Ch Name 15"=w505, "Measurement UI Displays.G.Ch Name 16"=w504) -> (w520:T9)
            n253 = call-poly <vilib>:"Delacor_lib_QMH_Enqueue Message (poly).vi"("error in"=w557, "Message"="Initialize UI", "Message Queue in"=w556) -> ("error out"=w555:errorcluster)  [unwired: 7 in, 1 out]
          }
          frame "---Module Specific---" {
            # "Separator -- The following cases handle messages specific to this Module."
          }
          frame "Initialize UI" {
            # "Initializes UI Controls and Indicators"
            n254 = Unbundle By Name(w628) -> ("Measurement UI Controls.Start Ref"=w651:refnum<vi>, "Measurement UI Controls.Settings Ref"=w650:refnum<vi>, "Measurement UI Controls.Stop Ref"=w647:refnum<vi>, "Measurement UI Controls.Rec Ref"=w644:refnum<vi>, "Measurement UI Controls.Soft Trig"=w643:refnum<vi>, "Measurement UI Controls.Imp Start Ref"=w642:refnum<vi>, "Measurement UI Controls.Imp Stop Ref"=w641:refnum<vi>, "En/Dis Trig"=w639:refnum<vi>, "Measurement UI Controls.CNV Start Ref"=w638:refnum<vi>, "Measurement UI Controls.CNV Stop Ref"=w637:refnum<vi>, "Measurement UI Controls.CNV Rec"=w636:refnum<vi>, "Measurement UI Controls.EOC Start Ref"=w635:refnum<vi>, "Measurement UI Controls.EOC Stop Ref"=w634:refnum<vi>, "Measurement UI Controls.EOC Rec Ref"=w633:refnum<vi>, "UI Page"=w632:refnum<vi>, "LSL Listeners"=w603:refnum<vi>, "LSL En?"=w602:bool, "Measurement UI Displays.imp mode sel"=w594:refnum<vi>)
            n255 = call-poly <vilib>:"Delacor_lib_QMH_Enqueue Message (poly).vi"("error in"=w630, "Message"="Check WiFi AP", "Message Queue in"=w629) -> ("error out"=w606:errorcluster)  [unwired: 7 in, 1 out]
            n256 = property class="Str"(reference=w603, "Visible"=w602) -> (reference out=w600:refnum<vi>, error out=w601:errorcluster)  [unwired: 1 in]
            n257 = Build Array(w651, w650, w642, w638, w635) -> (w649:refnum<vi>[])
            n258 = Build Array(w644, w647, w643, w641, w637, w636, w634, w633, w594) -> (w646:refnum<vi>[])
            n259 = property class="TabCtl (strict)"(reference=w632, "Value"=UI_Tab_Select."Graph") -> ()  [unwired: 1 in, 2 out]
            n260 = Concatenate Strings("LSL Listeners" ("string"), "\n", "0" ("string")) -> (w596:string)
            n261 = property class="Str"(reference=w600, error in=w601, "Value"=w596) -> ()  [unwired: 2 out]
            n262 = property class="Str"(reference=w639, "Visible"=FALSE) -> ()  [unwired: 1 in, 2 out]
            n263 = call "Set Enable State on Multiple Controls.vi"("Enable?"=TRUE, "Controls"=w649) -> ()  [unwired: 10 in]
            n264 = call "Set Enable State on Multiple Controls.vi"("Enable?"=FALSE, "Controls"=w646) -> ()  [unwired: 10 in]
            n265 = Unbundle By Name(w628) -> ("Measurement UI Displays.Graph 1"=w627:refnum<vi>, "Measurement UI Displays.Graph 2"=w626:refnum<vi>, "Measurement UI Displays.Graph 3"=w625:refnum<vi>, "Measurement UI Displays.Graph 4"=w624:refnum<vi>, "Measurement UI Displays.Graph 5"=w623:refnum<vi>, "Measurement UI Displays.Graph 6"=w622:refnum<vi>, "Measurement UI Displays.Graph 7"=w621:refnum<vi>, "Measurement UI Displays.Graph 8"=w620:refnum<vi>, "Measurement UI Displays.Graph 9"=w619:refnum<vi>, "Measurement UI Displays.Graph 10"=w618:refnum<vi>, "Measurement UI Displays.Graph 11"=w617:refnum<vi>, "Measurement UI Displays.Graph 12"=w616:refnum<vi>, "Measurement UI Displays.Graph 13"=w615:refnum<vi>, "Measurement UI Displays.Graph 14"=w614:refnum<vi>, "Measurement UI Displays.Graph 15"=w613:refnum<vi>, "Measurement UI Displays.Graph 16"=w612:refnum<vi>, "Measurement UI Displays.Battery 2"=w610:refnum<vi>, "Measurement UI Displays.Data Trig"=w608:refnum<vi>, "Measurement UI Displays.Data Connection Status"=w605:refnum<vi>)
            n266 = Build Array(w627, w626, w625, w624, w623, w622, w621, w620, w619, w618, w617, w616, w615, w614, w613, w612) -> (w611:refnum<vi>[])
            n267 = call "Set Graphs to Default.vi"("Array"=w611) -> ()  [unwired: 11 in]
            n268 = property class="WFChart (strict)"(reference=w608, error in=w606, "History Data"=u8[] []) -> ()  [unwired: 2 out]
            n269 = property class="Slide (strict)"(reference=w610, error in=w606, "Value"=u8 0) -> ()  [unwired: 2 out]
            n270 = property class="Bool (strict)"(reference=w605, error in=w606, "Value"=TRUE) -> ()  [unwired: 2 out]
          }
          frame "Start" {
            # "End user pressed Start button. Need to request for Acquisition to start acquiring."
            n271 = Variant To Data(error in=w658, type="Test Data" ("Data Select 2"), Variant=w668) -> (data=w666:string, error out=w657:errorcluster)
            n272 = call-poly <vilib>:"Delacor_lib_QMH_Enqueue Message (poly).vi"("error in"=w657, "Message"="Clear All Charts", "Message Queue in"=w662) -> ("error out"=w659:errorcluster, "Message Queue out"=w660:refnum<class "Delacor_lib_QMH_Message Queue.lvclass">)  [unwired: 7 in]
            n273 = Unbundle By Name(w653) -> ("LSL En?"=w652:bool)
            n274 = case shown="\"Impedance Data\"" w666 {
              tunnel: w659 -> [w669 w673 w680 w687 w694 w699]
              tunnel: [w669 w670 w678 w684 w691 w698] -> w663
              tunnel: w652 -> [_ w672 w677 w686 w693 _]
              frame "False", Default {
              }
              frame "Test Data" {
                n275 = call "Command_TestData.vi"("error in"=w673) -> ("error out"=w671:errorcluster)  [unwired: 10 in]
                n276 = case shown="True" w672 {
                  tunnel: w671 -> [w674 w676]
                  tunnel: [w674 w675] -> w670
                  frame False {
                  }
                  frame True {
                    n277 = call "Init LSL Metadata.vi"("error in"=w676) -> ("error out"=w675:errorcluster)  [unwired: 10 in]
                  }
                }
              }
              frame "Live Data" {
                n278 = call "Command_LiveData.vi"("error in"=w680) -> ("error out"=w679:errorcluster)  [unwired: 10 in]
                n279 = case shown="True" w677 {
                  tunnel: w679 -> [w681 w683]
                  tunnel: [w681 w682] -> w678
                  frame False {
                  }
                  frame True {
                    n280 = call "Init LSL Metadata.vi"("error in"=w683) -> ("error out"=w682:errorcluster)  [unwired: 10 in]
                  }
                }
              }
              frame "Noise Data" {
                n281 = call "Command_NoiseData.vi"("error in"=w687) -> ("error out"=w685:errorcluster)  [unwired: 10 in]
                n282 = case shown="True" w686 {
                  tunnel: w685 -> [w688 w690]
                  tunnel: [w688 w689] -> w684
                  frame False {
                  }
                  frame True {
                    n283 = call "Init LSL Metadata.vi"("error in"=w690) -> ("error out"=w689:errorcluster)  [unwired: 10 in]
                  }
                }
              }
              frame "Impedance Data" {
                n284 = call "Command_ImpedanceData.vi"("error in"=w694) -> ("error out"=w692:errorcluster)  [unwired: 10 in]
                n285 = case shown="True" w693 {
                  tunnel: w692 -> [w695 w697]
                  tunnel: [w695 w696] -> w691
                  frame False {
                  }
                  frame True {
                    n286 = call "Init LSL Metadata.vi"("error in"=w697) -> ("error out"=w696:errorcluster)  [unwired: 10 in]
                  }
                }
              }
              frame "Demo Data" {
                n287 = call "Start Demo Data.vi"("error in"=w699) -> ("error out"=w698:errorcluster)  [unwired: 10 in]
              }
            }
            n288 = Bundle By Name(cluster=w653, "Acq State"=Acquisition_State."RUNNING", "Recording State"=FALSE) -> (w656:T9)
            n289 = call-poly <vilib>:"Delacor_lib_QMH_Enqueue Message (poly).vi"("error in"=w663, "Message"="Acquisition Started Interlocks", "Message Queue in"=w660) -> ("error out"=w664:errorcluster)  [unwired: 7 in, 1 out]
          }
          frame "Record Action" {
            # "End user pressed Record button. Need to request for Recording to start/stop."
            n290 = Unbundle By Name(w713) -> ("Recording State"=w709:bool, "Measurement UI Controls.Soft Trig"=w706:refnum<vi>, "menu reference"=w704:refnum<k9>, "En/Dis Trig"=w703:refnum<vi>, "Measurement UI Controls.Rec Ref"=w701:refnum<vi>)
            n291 = case shown="True" w709 {
              tunnel: w711 -> [w716 w721]
              tunnel: [w715 w723] -> w710
              tunnel: [w714 w719] -> w705
              tunnel: w704 -> [w718 w722]
              tunnel: w703 -> [w717 w720]
              tunnel: [w714 w719] -> w700
              frame False {
                w714 = TRUE
                # "Show Panel to acquire File Name"
                n292 = call "Menu-Start Log.vi"("error in"=w716, "Menu in"=w718) -> ()  [unwired: 10 in]
                n293 = property class="Str"(reference=w717, "Visible"=w714) -> ()  [unwired: 1 in, 2 out]
                n294 = call "Wake-Up File Name Query Loop.vi"("error in"=w716) -> ("error out"=w715:errorcluster)  [unwired: 10 in]
              }
              frame True {
                w719 = FALSE
                n295 = call "Menu-Stop Log.vi"("error in"=w721, "Menu in"=w722) -> ()  [unwired: 10 in]
                n296 = property class="Str"(reference=w720, "Visible"=w719) -> ()  [unwired: 1 in, 2 out]
                n297 = call "Stop Logging.vi"("error in (no error)"=w721) -> ("error out"=w723:errorcluster)  [unwired: 10 in]
              }
            }
            n298 = Not(x=w709) -> (.not. x?=w708:bool)
            n299 = Bundle By Name(cluster=w713, "Recording State"=w708) -> (w712:T9)
            n300 = Build Array(w706) -> (w707:refnum<vi>[])
            n301 = Build Array(w701) -> (w702:refnum<vi>[])
            n302 = call "Set Enable State on Multiple Controls.vi"("Enable?"=w705, "Controls"=w707) -> ()  [unwired: 10 in]
            n303 = call "Set Value on Multiple Controls.vi"("Enable?"=w700, "Controls"=w702) -> ()  [unwired: 10 in]
          }
          frame "Record Action CNV" {
            # "End user pressed Record button. Need to request for Recording to start/stop for CNV"
            n304 = Unbundle By Name(w727) -> ("Recording State CNV"=w724:bool, "menu reference"=w728:refnum<k9>, "Measurement UI Controls.CNV Rec"=w730:refnum<vi>)
            n305 = Format Date/Time String(time format string (%c)="%Y_%m_%d_%H_%M_%S") -> (date/time string=w734:string)  [unwired: 2 in]
            n306 = Not(x=w724) -> (.not. x?=w725:bool)
            n307 = Concatenate Strings(w734, "_CNV" ("string")) -> (w732:string)
            n308 = case shown="True" w724 {
              tunnel: w737 -> [w742 w746]
              tunnel: [w741 w747] -> w736
              tunnel: w732 -> [w740 _]
              tunnel: [TRUE ("Enable?") FALSE] -> w729
              tunnel: w728 -> [w738 w744]
              frame False {
                n309 = call "Menu-Start Log CNV.vi"("Menu in"=w738) -> ()  [unwired: 11 in]
                n310 = call "Initialize File.vi"("wait for reply (T)"=FALSE, "error in"=w742, "file name"=w740) -> ("error out"=w741:errorcluster)  [unwired: 6 in, 2 out]
              }
              frame True {
                n311 = call "Menu-Stop Log CNV.vi"("Menu in"=w744) -> ()  [unwired: 11 in]
                n312 = call "Stop Logging.vi"("error in (no error)"=w746) -> ("error out"=w747:errorcluster)  [unwired: 10 in]
              }
            }
            n313 = Bundle By Name(cluster=w727, "Recording State CNV"=w725) -> (w726:T9)
            n314 = Build Array(w730) -> (w731:refnum<vi>[])
            n315 = call "Set Value on Multiple Controls.vi"("Enable?"=w729, "Controls"=w731) -> ()  [unwired: 10 in]
          }
          frame "Record Action EOC" {
            # "End user pressed Record button. Need to request for Recording to start/stop for EOC"
            n316 = Unbundle By Name(w750) -> ("Recording State EOC"=w759:bool, "Measurement UI Controls.EOC Rec Ref"=w753:refnum<vi>, "menu reference"=w751:refnum<k9>)
            n317 = Format Date/Time String(time format string (%c)="%Y_%m_%d_%H_%M_%S") -> (date/time string=w757:string)  [unwired: 2 in]
            n318 = Not(x=w759) -> (.not. x?=w748:bool)
            n319 = Concatenate Strings(w757, "_EOC" ("string")) -> (w755:string)
            n320 = case shown="True" w759 {
              tunnel: w761 -> [w766 w770]
              tunnel: [w765 w771] -> w760
              tunnel: w755 -> [w764 _]
              tunnel: [TRUE ("Enable?") FALSE] -> w752
              tunnel: w751 -> [w762 w768]
              frame False {
                n321 = call "Menu-Start Log EOC.vi"("Menu in"=w762) -> ()  [unwired: 11 in]
                n322 = call "Initialize File.vi"("wait for reply (T)"=FALSE, "error in"=w766, "file name"=w764) -> ("error out"=w765:errorcluster)  [unwired: 6 in, 2 out]
              }
              frame True {
                n323 = call "Menu-Stop Log EOC.vi"("Menu in"=w768) -> ()  [unwired: 11 in]
                n324 = call "Stop Logging.vi"("error in (no error)"=w770) -> ("error out"=w771:errorcluster)  [unwired: 10 in]
              }
            }
            n325 = Bundle By Name(cluster=w750, "Recording State EOC"=w748) -> (w749:T9)
            n326 = Build Array(w753) -> (w754:refnum<vi>[])
            n327 = call "Set Value on Multiple Controls.vi"("Enable?"=w752, "Controls"=w754) -> ()  [unwired: 10 in]
          }
          frame "Acquisition Started Interlocks" {
            # "UI control state for acquisition in progress"
            n328 = Unbundle By Name(w775) -> ("Measurement UI Controls.Rec Ref"=w774:refnum<vi>, "Measurement UI Controls.Stop Ref"=w785:refnum<vi>, "Measurement UI Controls.Start Ref"=w780:refnum<vi>, "Measurement UI Controls.Settings Ref"=w779:refnum<vi>)
            n329 = Build Array(w785, w774) -> (w784:refnum<vi>[])
            n330 = Build Array(w780, w779) -> (w781:refnum<vi>[])
            n331 = Build Array(w774) -> (w773:refnum<vi>[])
            n332 = call "Set Enable State on Multiple Controls.vi"("Enable?"=TRUE, "Controls"=w784) -> ()  [unwired: 10 in]
            n333 = call "Set Enable State on Multiple Controls.vi"("Enable?"=FALSE, "Controls"=w781) -> ()  [unwired: 10 in]
            n334 = call "Set Value on Multiple Controls.vi"("Enable?"=FALSE, "Controls"=w773) -> ()  [unwired: 10 in]
            n335 = call "Clear All Charts.vi"("error in"=w778) -> ("error out"=w777:errorcluster)  [unwired: 10 in]
            n336 = Unbundle By Name(w775) -> ("menu reference"=w776:refnum<k9>)
            n337 = call "Menu-Start Acq.vi"("Menu in"=w776) -> ()  [unwired: 11 in]
          }
          frame "CNV Started Interlocks" {
            # "UI control state for CNV in progress"
            n338 = Unbundle By Name(w793) -> ("Measurement UI Controls.CNV Rec"=w794:refnum<vi>, "Measurement UI Controls.CNV Stop Ref"=w799:refnum<vi>, "Measurement UI Controls.CNV Start Ref"=w792:refnum<vi>, "Measurement UI Controls.Settings Ref"=w790:refnum<vi>)  [unwired: 1 out]
            n339 = Build Array(w799, w794) -> (w798:refnum<vi>[])
            n340 = Build Array(w792, w790) -> (w791:refnum<vi>[])
            n341 = call "Set Enable State on Multiple Controls.vi"("Enable?"=TRUE, "Controls"=w798) -> ()  [unwired: 10 in]
            n342 = call "Set Enable State on Multiple Controls.vi"("Enable?"=FALSE, "Controls"=w791) -> ()  [unwired: 10 in]
            n343 = Unbundle By Name(w793) -> ("menu reference"=w789:refnum<k9>, "Measurement UI Controls.CNV Rec"=w786:refnum<vi>)
            n344 = call "Menu-Start Acq CNV.vi"("Menu in"=w789) -> ()  [unwired: 11 in]
            n345 = Build Array(w786) -> (w788:refnum<vi>[])
            n346 = call "Set Value on Multiple Controls.vi"("Enable?"=FALSE, "Controls"=w788) -> ()  [unwired: 10 in]
          }
          frame "EOC Started Interlocks" {
            # "UI control state for EOC in progress"
            n347 = Unbundle By Name(w807) -> ("Measurement UI Controls.EOC Rec Ref"=w808:refnum<vi>, "Measurement UI Controls.EOC Stop Ref"=w813:refnum<vi>, "Measurement UI Controls.EOC Start Ref"=w806:refnum<vi>, "Measurement UI Controls.Settings Ref"=w804:refnum<vi>)  [unwired: 1 out]
            n348 = Build Array(w813, w808) -> (w812:refnum<vi>[])
            n349 = Build Array(w806, w804) -> (w805:refnum<vi>[])
            n350 = call "Set Enable State on Multiple Controls.vi"("Enable?"=TRUE, "Controls"=w812) -> ()  [unwired: 10 in]
            n351 = call "Set Enable State on Multiple Controls.vi"("Enable?"=FALSE, "Controls"=w805) -> ()  [unwired: 10 in]
            n352 = Unbundle By Name(w807) -> ("menu reference"=w803:refnum<k9>, "Measurement UI Controls.EOC Rec Ref"=w800:refnum<vi>)
            n353 = Build Array(w800) -> (w802:refnum<vi>[])
            n354 = call "Menu-Start Acq EOC.vi"("Menu in"=w803) -> ()  [unwired: 11 in]
            n355 = call "Set Value on Multiple Controls.vi"("Enable?"=FALSE, "Controls"=w802) -> ()  [unwired: 10 in]
          }
          frame "CNV Stopped Interlocks" {
            # "UI control state for CNV in rest"
            n356 = Unbundle By Name(w822) -> ("Measurement UI Controls.CNV Rec"=w819:refnum<vi>, "Measurement UI Controls.CNV Stop Ref"=w827:refnum<vi>, "Measurement UI Controls.CNV Start Ref"=w821:refnum<vi>, "Measurement UI Controls.Settings Ref"=w818:refnum<vi>)  [unwired: 1 out]
            n357 = Build Array(w827, w819) -> (w826:refnum<vi>[])
            n358 = Build Array(w821, w818) -> (w820:refnum<vi>[])
            n359 = call "Set Enable State on Multiple Controls.vi"("Enable?"=FALSE, "Controls"=w826) -> ()  [unwired: 10 in]
            n360 = call "Set Enable State on Multiple Controls.vi"("Enable?"=TRUE, "Controls"=w820) -> ()  [unwired: 10 in]
            n361 = Unbundle By Name(w822) -> ("menu reference"=w817:refnum<k9>, "Measurement UI Controls.CNV Rec"=w814:refnum<vi>)
            n362 = Build Array(w814) -> (w816:refnum<vi>[])
            n363 = call "Menu-Stop Acq CNV.vi"("Menu in"=w817) -> ()  [unwired: 11 in]
            n364 = call "Set Value on Multiple Controls.vi"("Enable?"=FALSE, "Controls"=w816) -> ()  [unwired: 10 in]
          }
          frame "EOC Stopped Interlocks" {
            # "UI control state for EOC in rest"
            n365 = Unbundle By Name(w836) -> ("Measurement UI Controls.EOC Rec Ref"=w833:refnum<vi>, "Measurement UI Controls.EOC Stop Ref"=w841:refnum<vi>, "Measurement UI Controls.EOC Start Ref"=w835:refnum<vi>, "Measurement UI Controls.Settings Ref"=w832:refnum<vi>)  [unwired: 1 out]
            n366 = Build Array(w841, w833) -> (w840:refnum<vi>[])
            n367 = Build Array(w835, w832) -> (w834:refnum<vi>[])
            n368 = call "Set Enable State on Multiple Controls.vi"("Enable?"=FALSE, "Controls"=w840) -> ()  [unwired: 10 in]
            n369 = call "Set Enable State on Multiple Controls.vi"("Enable?"=TRUE, "Controls"=w834) -> ()  [unwired: 10 in]
            n370 = Unbundle By Name(w836) -> ("menu reference"=w831:refnum<k9>, "Measurement UI Controls.EOC Rec Ref"=w828:refnum<vi>)
            n371 = call "Menu-Stop Acq EOC.vi"("Menu in"=w831) -> ()  [unwired: 11 in]
            n372 = Build Array(w828) -> (w830:refnum<vi>[])
            n373 = call "Set Value on Multiple Controls.vi"("Enable?"=FALSE, "Controls"=w830) -> ()  [unwired: 10 in]
          }
          frame "Set Display" {
            # "Displays Requested Page"
            n374 = Variant To Data(error in=w851, type="", Variant=w850) -> (data=w846:string, error out=w843:errorcluster)
            n375 = Unbundle By Name(w848) -> ("UI Page"=w847:refnum<vi>, "menu reference"=w844:refnum<k9>)
            n376 = call "Set Menu for View Selection.vi"("error in"=w843, "String"=w846, "Menu in"=w844) -> ("Value"=w842:T20)  [unwired: 8 in]
            n377 = property class="TabCtl (strict)"(reference=w847, "Value"=w842) -> (error out=w845:errorcluster)  [unwired: 1 in, 1 out]
          }
          frame "Imp Gnd Loop Locks" {
            # "Enable: Stop\nDisable: Start, Settings"
            n378 = Unbundle By Name(w854) -> ("Measurement UI Controls.Rec Ref"=w852:refnum<vi>, "Measurement UI Controls.Stop Ref"=w861:refnum<vi>, "Measurement UI Controls.Start Ref"=w856:refnum<vi>, "Measurement UI Controls.Settings Ref"=w855:refnum<vi>)
            n379 = Build Array(w861, w852) -> (w860:refnum<vi>[])
            n380 = Build Array(w856, w855) -> (w857:refnum<vi>[])
            n381 = call "Set Enable State on Multiple Controls.vi"("Enable?"=TRUE, "Controls"=w860) -> ()  [unwired: 10 in]
            n382 = call "Set Enable State on Multiple Controls.vi"("Enable?"=FALSE, "Controls"=w857) -> ()  [unwired: 10 in]
          }
          frame "Impedance Stopped Interlocks" {
            n383 = Unbundle By Name(w864) -> ("Measurement UI Controls.Imp Start Ref"=w867:refnum<vi>, "Measurement UI Controls.Imp Stop Ref"=w868:refnum<vi>, "Measurement UI Controls.Settings Ref"=w866:refnum<vi>, "Measurement UI Displays.imp mode sel"=w862:refnum<vi>)
            n384 = Build Array(w867, w866) -> (w872:refnum<vi>[])
            n385 = Build Array(w868, w862) -> (w869:refnum<vi>[])
            n386 = call "Set Enable State on Multiple Controls.vi"("Enable?"=TRUE, "Controls"=w872) -> ()  [unwired: 10 in]
            n387 = call "Set Enable State on Multiple Controls.vi"("Enable?"=FALSE, "Controls"=w869) -> ()  [unwired: 10 in]
            n388 = Unbundle By Name(w864) -> ("menu reference"=w865:refnum<k9>)
            n389 = call "Menu-Stop Imp.vi"("error in"=w863, "Menu in"=w865) -> ()  [unwired: 10 in]
          }
          frame "Impedance Started Interlocks" {
            n390 = Unbundle By Name(w874) -> ("Measurement UI Controls.Imp Start Ref"=w883:refnum<vi>, "Measurement UI Controls.Imp Stop Ref"=w884:refnum<vi>, "Measurement UI Controls.Settings Ref"=w882:refnum<vi>, "Measurement UI Displays.imp mode sel"=w875:refnum<vi>)
            n391 = call "Update Application Settings.vi"("error in"=w881) -> ("error out"=w878:errorcluster, "timed out?"=w880:bool, "Reply Payload"=w879:T30)  [unwired: 8 in]
            n392 = Build Array(w883, w882) -> (w888:refnum<vi>[])
            n393 = Build Array(w884, w875) -> (w885:refnum<vi>[])
            n394 = case shown="False" w880 {
              tunnel: w879 -> [w912 _]
              tunnel: w878 -> [w911 w916]
              tunnel: [w911 w915] -> w877
              frame False {
                n395 = Unbundle By Name(w912) -> ("Settings.EEG Channels.16 EEG Channels"=w910:T31)
                n396 = for {
                  tunnel: w910 -> [w914] mode=indexing
                  tunnel: [w913] -> w909 mode=indexing
                  n397 = Unbundle By Name(w914) -> ("Channel Name"=w913:string)
                }
                n398 = Index Array(array=w909, index #1=0 ("index")) -> (element #1=→"Ch Name 1":string, element #2=→"Ch Name 2":string, element #3=→"Ch Name 3":string, element #4=→"Ch Name 4":string, element #5=→"Ch Name 5":string, element #6=→"Ch Name 6":string, element #7=→"Ch Name 7":string, element #8=→"Ch Name 8":string, element #9=→"Ch Name 9":string, element #10=→"Ch Name 10":string, element #11=→"Ch Name 11":string, element #12=→"Ch Name 12":string, element #13=→"Ch Name 13":string, element #14=→"Ch Name 14":string, element #15=→"Ch Name 15":string, element #16=→"Ch Name 16":string)  [unwired: 15 in]
              }
              frame True {
                n399 = call <vilib>:"Clear Errors.vi"("error in (no error)"=w916) -> ("error out"=w915:errorcluster)  [unwired: 5 in, 1 out]
              }
            }
            n400 = call "Set Enable State on Multiple Controls.vi"("Enable?"=FALSE, "Controls"=w888) -> ()  [unwired: 10 in]
            n401 = call "Set Enable State on Multiple Controls.vi"("Enable?"=TRUE, "Controls"=w885) -> ()  [unwired: 10 in]
            n402 = flat-sequence {
              tunnel: w874 -> [w891]
              tunnel: [w889] -> w873
              frame #0 {
                n403 = invoke on="imp mode" class="Bool (strict)" method="Reinit To Default"() -> ()  [unwired: 3 in, 3 out]
                n404 = Bundle By Name(cluster=w891, "Imp Mode"=FALSE) -> (w889:T9)
              }
            }
            n405 = Unbundle By Name(w873) -> ("menu reference"=w876:refnum<k9>)
            n406 = call "Menu-Start Imp.vi"("Menu in"=w876) -> ()  [unwired: 11 in]
          }
          frame "Stop" {
            # "End user pressed Stop button. Need to request for Acquisition to stop acquiring and for Logger to stop logging."
            n407 = Variant To Data(error in=w925, type="", Variant=w924) -> (data=w922:string, error out=w926:errorcluster)
            n408 = case shown="\"True\", Default" w922 {
              tunnel: [w933 w935] -> w921
              tunnel: w926 -> [w934 w937]
              frame "Demo Data" {
                n409 = call "Stop Demo Data.vi"("error in"=w934) -> ("error out"=w933:errorcluster)  [unwired: 10 in]
              }
              frame "True", Default {
                n410 = call "Command_GoToIdle.vi"("error in"=w937) -> ("error out"=w941:errorcluster)  [unwired: 10 in]
                n411 = call-poly <userlib>:"MGI Wait.vi"("ms"=u32 5, "Error In"=w941) -> ("Error Out"=w939:errorcluster)  [unwired: 5 in]
                n412 = call "Stop Logging.vi"("error in (no error)"=w939) -> ("error out"=w938:errorcluster)  [unwired: 10 in]
                n413 = call "Stop Acquiring.vi"("error in (no error)"=w938) -> ("error out"=w936:errorcluster)  [unwired: 10 in]
                n414 = call "Stop Stream.vi"("error in"=w936) -> ("error out"=w935:errorcluster)  [unwired: 10 in]
              }
            }
            n415 = call-poly <userlib>:"MGI Wait.vi"("ms"=u32 2, "Error In"=w921) -> ("Error Out"=w929:errorcluster)  [unwired: 5 in]
            n416 = flat-sequence {
              tunnel: ["Ready .." ("Status")] -> w930
              tunnel: w929 -> [_]
              frame #0 {
              }
            }
            n417 = local write "Status"(w930) -> ()
            n418 = Bundle By Name(cluster=w932, "Status"=w930, "Acq State"=Acquisition_State."IDLE", "Recording State"=FALSE) -> (w931:T9)
            n419 = call-poly <vilib>:"Delacor_lib_QMH_Enqueue Message (poly).vi"("error in"=w921, "Message"="Acquisition Stopped Interlocks", "Message Queue in"=w920) -> ("error out"=w918:errorcluster)  [unwired: 7 in, 1 out]
          }
          frame "Impedance Stop" {
            # "End user pressed Stop button. Need to request for Acquisition to stop acquiring"
            n420 = call "Command_GoToIdle.vi"("error in"=w946) -> ("error out"=w949:errorcluster)  [unwired: 10 in]
            n421 = call-poly <userlib>:"MGI Wait.vi"("ms"=u32 5, "Error In"=w949) -> ("Error Out"=w948:errorcluster)  [unwired: 5 in]
            n422 = call "Stop IMP acquiring.vi"("error in"=w948) -> ("error out"=w947:errorcluster)  [unwired: 10 in]
            n423 = Bundle By Name(cluster=w945, "Acq State"=Acquisition_State."IDLE") -> (w944:T9)
            n424 = call-poly <vilib>:"Delacor_lib_QMH_Enqueue Message (poly).vi"("error in"=w947, "Message"="Impedance Stopped Interlocks", "Message Queue in"=w950) -> ("error out"=w951:errorcluster)  [unwired: 7 in, 1 out]
          }
          frame "Stop EOC Demo" {
            # "End user pressed EOC Stop"
            n425 = call "Command_GoToIdle.vi"("error in"=w957) -> ("error out"=w960:errorcluster)  [unwired: 10 in]
            n426 = call-poly <userlib>:"MGI Wait.vi"("ms"=u32 5, "Error In"=w960) -> ("Error Out"=w959:errorcluster)  [unwired: 5 in]
            n427 = call "Stop IMP acquiring.vi"("error in"=w959) -> ("error out"=w958:errorcluster)  [unwired: 10 in]
            n428 = Bundle By Name(cluster=w956, "Acq State"=Acquisition_State."IDLE") -> (w955:T9)
            n429 = call-poly <vilib>:"Delacor_lib_QMH_Enqueue Message (poly).vi"("error in"=w958, "Message"="EOC Stopped Interlocks", "Message Queue in"=w961) -> ("error out"=w962:errorcluster)  [unwired: 7 in, 1 out]
          }
          frame "Acquisition Stopped Interlocks" {
            n430 = Unbundle By Name(w969) -> ("Measurement UI Controls.Rec Ref"=w965:refnum<vi>, "Measurement UI Controls.Stop Ref"=w976:refnum<vi>, "Measurement UI Controls.Start Ref"=w975:refnum<vi>, "Measurement UI Controls.Settings Ref"=w974:refnum<vi>, "Measurement UI Controls.Soft Trig"=w971:refnum<vi>)
            n431 = Unbundle By Name(w969) -> ("menu reference"=w970:refnum<k9>)
            n432 = Build Array(w965) -> (w967:refnum<vi>[])
            n433 = Build Array(w971, w976, w965) -> (w978:refnum<vi>[])
            n434 = Build Array(w975, w974) -> (w973:refnum<vi>[])
            n435 = call "Menu-Stop Acq.vi"("error in"=w968, "Menu in"=w970) -> ()  [unwired: 10 in]
            n436 = call "Set Value on Multiple Controls.vi"("Enable?"=FALSE, "Controls"=w967) -> ()  [unwired: 10 in]
            n437 = call "Set Enable State on Multiple Controls.vi"("Enable?"=FALSE, "Controls"=w978) -> ()  [unwired: 10 in]
            n438 = call "Set Enable State on Multiple Controls.vi"("Enable?"=TRUE, "Controls"=w973) -> ()  [unwired: 10 in]
          }
          frame "STOP_GUI" {
            # "Call to close GUI from another modules"
            n439 = Variant To Data(error in=w993, type=T15 {"Message for the Request"=""} ("STOP_GUI Argument"), Variant=w991) -> (data=w989:T15, error out=w985:errorcluster)
            n440 = Unbundle By Name(w989) -> ("Message for the Request"=w986:string)
            n441 = call "User Message.vi"("error in"=w985, "String in"=w986) -> ("error out"=w984:errorcluster)  [unwired: 9 in]
            n442 = call "Stop Acquiring.vi"("error in (no error)"=w984) -> ("error out"=w988:errorcluster)  [unwired: 10 in]
            n443 = call "Stop Logging.vi"("error in (no error)"=w988) -> ("error out"=w987:errorcluster)  [unwired: 10 in]
            n444 = call-poly <userlib>:"MGI Wait.vi"("ms"=u32 100, "Error In"=w987) -> ("Error Out"=w981:errorcluster)  [unwired: 5 in]
            n445 = call-poly <vilib>:"Delacor_lib_QMH_Enqueue Message (poly).vi"("error in"=w981, "Message"="Exit", "Message Queue in"=w980) -> ("error out"=w979:errorcluster)  [unwired: 7 in, 1 out]
          }
          frame "Update_Display" {
            (unwired) u8 100
            # "#Change"
            # "Call to close GUI from another modules"
            n446 = Unbundle By Name(w994) -> ("Display  cnt"=w997:u8)
            n447 = Variant To Data(error in=w1007, type=cluster{"WiBCI16T Data out":T21, "En MAP":u16} {"WiBCI16T Data out"={"EEG Ch 1"=0.0, "EEG Ch 2"=0.0, "EEG Ch 3"=0.0, "EEG Ch 4"=0.0, "EEG Ch 5"=0.0, "EEG Ch 6"=0.0, "EEG Ch 7"=0.0, "EEG Ch 8"=0.0, "EEG Ch 9"=0.0, "EEG Ch 10"=0.0, "EEG Ch 11"=0.0, "EEG Ch 12"=0.0, "EEG Ch 13"=0.0, "EEG Ch 14"=0.0, "EEG Ch 15"=0.0, "EEG Ch 16"=0.0, "X-Accel"=0, "Y-Accel"=0, "Z-Accel"=0, "X-Gyro"=0, "Y-Gyro"=0, "Z-Gyro"=0, "Timer"=0, "Packet ID"=0, "HW Trig1"=0, "SW Trig1"=0, "HW Trig2"=0, "SW Trig2"=0, "WiBCI Status"={"Mode Byte"=0, "Ch Config"=0, "Ch Ref Map"=0, "Ch Enable Map"=0, "Temperature"=0.0, "Battery"=0, "Version"=""}, "Reg Map"={"ADS1"=[], "ADS2"=[]}}, "En MAP"=0}, Variant=w1006) -> (data=w1002:cluster{"WiBCI16T Data out":T21, "En MAP":u16}, error out=w1005:errorcluster)
            n448 = case shown="103" w997 {
              selector: w997 -> [w1012 w1018 _]
              tunnel: w1002 -> [_ w1016 w1025]
              tunnel: [w1011 w1017 u8 102] -> w996
              tunnel: w994 -> [_ _ w1023]
              frame 0, Default {
                n449 = Increment(x=w1012) -> (x+1=w1011:u8)
              }
              frame 100..102 {
                n450 = Unbundle By Name(w1016) -> ("WiBCI16T Data out.SW Trig1"=w1013:i8)
                n451 = Increment(x=w1018) -> (x+1=w1017:u8)
                n452 = Greater Or Equal?(x=w1013, y=i8 45) -> (x >= y?=w1014:bool)
                n453 = case shown="True" w1014 {
                  tunnel: w1013 -> [_ w1019]
                  frame False {
                  }
                  frame True {
                    n454 = local write "Data Trig"(w1019) -> ()
                  }
                }
              }
              frame 103 {
                n455 = Unbundle By Name(w1023) -> ("Measurement UI Displays.Graph Sel"=w1020:u8, "LSL En?"=w1022:bool, "LSL Listeners"=w1021:refnum<vi>)
                n456 = case shown="1..16" w1020 {
                  selector: w1020 -> [w1052 _]
                  tunnel: w1025 -> [w1053 w1107]
                  frame 1..16 {
                    n457 = Unbundle By Name(w1053) -> ("WiBCI16T Data out.EEG Ch 1"=w1051:dbl, "WiBCI16T Data out.EEG Ch 2"=w1050:dbl, "WiBCI16T Data out.EEG Ch 3"=w1049:dbl, "WiBCI16T Data out.EEG Ch 4"=w1048:dbl, "WiBCI16T Data out.EEG Ch 5"=w1047:dbl, "WiBCI16T Data out.EEG Ch 6"=w1046:dbl, "WiBCI16T Data out.EEG Ch 7"=w1045:dbl, "WiBCI16T Data out.EEG Ch 8"=w1044:dbl, "WiBCI16T Data out.EEG Ch 9"=w1043:dbl, "WiBCI16T Data out.EEG Ch 10"=w1042:dbl, "WiBCI16T Data out.EEG Ch 11"=w1041:dbl, "WiBCI16T Data out.EEG Ch 12"=w1040:dbl, "WiBCI16T Data out.EEG Ch 13"=w1039:dbl, "WiBCI16T Data out.EEG Ch 14"=w1038:dbl, "WiBCI16T Data out.EEG Ch 15"=w1037:dbl, "WiBCI16T Data out.EEG Ch 16"=w1036:dbl)
                    n458 = case shown="4" w1052 {
                      tunnel: w1051 -> [_ w1055 _ _ _ _ _ _ _ _ _ _ _ _ _ _ _]
                      tunnel: w1050 -> [_ _ w1056 _ _ _ _ _ _ _ _ _ _ _ _ _ _]
                      tunnel: w1049 -> [_ _ _ w1057 _ _ _ _ _ _ _ _ _ _ _ _ _]
                      tunnel: w1048 -> [_ _ _ _ w1058 _ _ _ _ _ _ _ _ _ _ _ _]
                      tunnel: w1047 -> [_ _ _ _ _ w1059 _ _ _ _ _ _ _ _ _ _ _]
                      tunnel: w1046 -> [_ _ _ _ _ _ w1060 _ _ _ _ _ _ _ _ _ _]
                      tunnel: w1045 -> [_ _ _ _ _ _ _ w1061 _ _ _ _ _ _ _ _ _]
                      tunnel: w1044 -> [_ _ _ _ _ _ _ _ w1062 _ _ _ _ _ _ _ _]
                      tunnel: w1043 -> [_ _ _ _ _ _ _ _ _ w1063 _ _ _ _ _ _ _]
                      tunnel: w1042 -> [_ _ _ _ _ _ _ _ _ _ w1064 _ _ _ _ _ _]
                      tunnel: w1041 -> [_ _ _ _ _ _ _ _ _ _ _ w1065 _ _ _ _ _]
                      tunnel: w1040 -> [_ _ _ _ _ _ _ _ _ _ _ _ w1066 _ _ _ _]
                      tunnel: w1039 -> [_ _ _ _ _ _ _ _ _ _ _ _ _ w1067 _ _ _]
                      tunnel: w1038 -> [_ _ _ _ _ _ _ _ _ _ _ _ _ _ w1068 _ _]
                      tunnel: w1037 -> [_ _ _ _ _ _ _ _ _ _ _ _ _ _ _ w1069 _]
                      tunnel: w1036 -> [_ _ _ _ _ _ _ _ _ _ _ _ _ _ _ _ w1070]
                      tunnel: [0.0 w1055 w1056 w1057 w1058 w1059 w1060 w1061 w1062 w1063 w1064 w1065 w1066 w1067 w1068 w1069 w1070] -> w1035
                      frame 0, Default {
                      }
                      frame 1 {
                      }
                      frame 2 {
                      }
                      frame 3 {
                      }
                      frame 4 {
                      }
                      frame 5 {
                      }
                      frame 6 {
                      }
                      frame 7 {
                      }
                      frame 8 {
                      }
                      frame 9 {
                      }
                      frame 10 {
                      }
                      frame 11 {
                      }
                      frame 12 {
                      }
                      frame 13 {
                      }
                      frame 14 {
                      }
                      frame 15 {
                      }
                      frame 16 {
                      }
                    }
                    n459 = Multiply(x=w1035, y=1000000.0) -> (x*y=w1033:dbl)
                    n460 = call <vilib>:"Butterworth Filter PtByPt.vi"("initialize"=FALSE, "order"=2, "filter type"=Filter_Passband_Type."Bandpass", "low cutoff freq: fl"=0.125, "high cutoff freq: fh"=45.0, "sampling freq: fs"=250.0, "x"=w1033) -> ("Filtered x"=→"Single Chart":dbl)  [unwired: 2 in, 1 out]
                  }
                  frame 0, 17, Default {
                    # "Decimate display\nby a factor of 4"
                    n461 = Unbundle By Name(w1107) -> ("WiBCI16T Data out.EEG Ch 1"=w1106:dbl, "WiBCI16T Data out.EEG Ch 2"=w1104:dbl, "WiBCI16T Data out.EEG Ch 3"=w1105:dbl, "WiBCI16T Data out.EEG Ch 4"=w1103:dbl, "WiBCI16T Data out.EEG Ch 5"=w1102:dbl, "WiBCI16T Data out.EEG Ch 6"=w1101:dbl, "WiBCI16T Data out.EEG Ch 7"=w1100:dbl, "WiBCI16T Data out.EEG Ch 8"=w1099:dbl, "WiBCI16T Data out.EEG Ch 9"=w1098:dbl, "WiBCI16T Data out.EEG Ch 10"=w1097:dbl, "WiBCI16T Data out.EEG Ch 11"=w1096:dbl, "WiBCI16T Data out.EEG Ch 12"=w1095:dbl, "WiBCI16T Data out.EEG Ch 13"=w1094:dbl, "WiBCI16T Data out.EEG Ch 14"=w1093:dbl, "WiBCI16T Data out.EEG Ch 15"=w1092:dbl, "WiBCI16T Data out.EEG Ch 16"=w1091:dbl, "En MAP"=w1090:u16, "WiBCI16T Data out.SW Trig1"=→"Data Trig":i8)
                    n462 = Number To Boolean Array(number=w1090) -> (Boolean array=w1089:bool[])
                    n463 = Index Array(array=w1089, index #1=0 ("index")) -> (element #1=w1087:bool, element #2=w1086:bool, element #3=w1085:bool, element #4=w1084:bool, element #5=w1083:bool, element #6=w1082:bool, element #7=w1081:bool, element #8=w1080:bool, element #9=w1079:bool, element #10=w1078:bool, element #11=w1077:bool, element #12=w1076:bool, element #13=w1075:bool, element #14=w1074:bool, element #15=w1073:bool, element #16=w1072:bool)  [unwired: 15 in]
                    n464 = case shown="True" w1078 {
                      tunnel: w1100 -> [_ w1117]
                      frame False {
                      }
                      frame True {
                        "Data 7" <- w1117
                      }
                    }
                    n465 = case shown="True" w1077 {
                      tunnel: w1101 -> [_ w1118]
                      frame False {
                      }
                      frame True {
                        "Data 6" <- w1118
                      }
                    }
                    n466 = case shown="True" w1079 {
                      tunnel: w1099 -> [_ w1116]
                      frame False {
                      }
                      frame True {
                        "Data 8" <- w1116
                      }
                    }
                    n467 = case shown="True" w1072 {
                      tunnel: w1106 -> [_ w1123]
                      frame False {
                      }
                      frame True {
                        "Data 1" <- w1123
                      }
                    }
                    n468 = case shown="True" w1074 {
                      tunnel: w1105 -> [_ w1121]
                      frame False {
                      }
                      frame True {
                        "Data 3" <- w1121
                      }
                    }
                    n469 = case shown="True" w1080 {
                      tunnel: w1098 -> [_ w1115]
                      frame False {
                      }
                      frame True {
                        "Data 9" <- w1115
                      }
                    }
                    n470 = case shown="True" w1081 {
                      tunnel: w1097 -> [_ w1114]
                      frame False {
                      }
                      frame True {
                        "Data 10" <- w1114
                      }
                    }
                    n471 = case shown="True" w1087 {
                      tunnel: w1091 -> [_ w1108]
                      frame False {
                      }
                      frame True {
                        "Data 16" <- w1108
                      }
                    }
                    n472 = case shown="True" w1082 {
                      tunnel: w1096 -> [_ w1113]
                      frame False {
                      }
                      frame True {
                        "Data 11" <- w1113
                      }
                    }
                    n473 = case shown="True" w1086 {
                      tunnel: w1092 -> [_ w1109]
                      frame False {
                      }
                      frame True {
                        "Data 15" <- w1109
                      }
                    }
                    n474 = case shown="True" w1073 {
                      tunnel: w1104 -> [_ w1122]
                      frame False {
                      }
                      frame True {
                        "Data 2" <- w1122
                      }
                    }
                    n475 = case shown="True" w1083 {
                      tunnel: w1095 -> [_ w1112]
                      frame False {
                      }
                      frame True {
                        "Data 12" <- w1112
                      }
                    }
                    n476 = case shown="True" w1085 {
                      tunnel: w1093 -> [_ w1110]
                      frame False {
                      }
                      frame True {
                        "Data 14" <- w1110
                      }
                    }
                    n477 = case shown="True" w1084 {
                      tunnel: w1094 -> [_ w1111]
                      frame False {
                      }
                      frame True {
                        "Data 13" <- w1111
                      }
                    }
                    n478 = case shown="True" w1076 {
                      tunnel: w1102 -> [_ w1119]
                      frame False {
                      }
                      frame True {
                        "Data 5" <- w1119
                      }
                    }
                    n479 = case shown="True" w1075 {
                      tunnel: w1103 -> [_ w1120]
                      frame False {
                      }
                      frame True {
                        "Data 4" <- w1120
                      }
                    }
                  }
                }
                n480 = case shown="True" w1022 {
                  tunnel: w1021 -> [_ w1127]
                  frame False {
                  }
                  frame True {
                    n481 = feedback #2(u8 0) -> (w1125:u8)
                    n482 = case shown="250" w1125 {
                      selector: w1125 -> [w1129 _]
                      tunnel: w1127 -> [_ w1140]
                      tunnel: [w1128 u8 0] -> w1124
                      frame 0, Default {
                        n483 = Increment(x=w1129) -> (x+1=w1128:u8)
                      }
                      frame 250 {
                        n484 = call "Get Listeners count.vi"() -> ("error out"=w1138:errorcluster, "timed out?"=w1135:bool, "Listeners"=w1133:i32)  [unwired: 9 in]
                        n485 = Select(t=0, s=w1135, f=w1133) -> (s? t:f=w1132:i32)
                        n486 = Number To Decimal String(number=w1132) -> (decimal integer string=w1131:string)  [unwired: 1 in]
                        n487 = Concatenate Strings("LSL Listeners" ("string"), "\n", w1131) -> (w1139:string)
                        n488 = property class="Str"(reference=w1140, error in=w1138, "Value"=w1139) -> ()  [unwired: 2 out]
                      }
                    }
                    n489 = feedback-in #2(w1124) -> ()
                  }
                }
              }
            }
            n490 = Unbundle By Name(w1002) -> ("WiBCI16T Data out.WiBCI Status.Battery"=w1000:u8)
            n491 = Add(x=u8 20, y=w1000) -> (x+y=w998:u8)
            "Battery" <- w998
            n492 = case shown="..30" w998 {
              tunnel: [u32 16771090 u32 16723218 u32 6618880] -> w999
              frame 50, Default {
              }
              frame ..30 {
              }
              frame 70.. {
              }
            }
            n493 = property on="Battery" class="Slide (strict)"("Fill Color"=w999) -> ()  [unwired: 2 in, 2 out]
            n494 = Bundle By Name(cluster=w994, "Display  cnt"=w996) -> (w995:T9)
            "Data Status" <- TRUE
          }
          frame "Update_IMP_Display" {
            # "Update for Impedance Display"
            n495 = feedback #3(u8 0) -> (w1146:u8)
            n496 = case shown="250" w1146 {
              selector: w1146 -> [_ w1154]
              tunnel: [u8 0 w1153] -> w1145
              frame 250 {
              }
              frame 1, Default {
                n497 = Increment(x=w1154) -> (x+1=w1153:u8)
              }
            }
            n498 = feedback-in #3(w1145) -> ()
            n499 = Variant To Data(error in=w1151, type=cluster{"WiBCI16T Data out":T21, "En MAP":u16} {"WiBCI16T Data out"={"EEG Ch 1"=0.0, "EEG Ch 2"=0.0, "EEG Ch 3"=0.0, "EEG Ch 4"=0.0, "EEG Ch 5"=0.0, "EEG Ch 6"=0.0, "EEG Ch 7"=0.0, "EEG Ch 8"=0.0, "EEG Ch 9"=0.0, "EEG Ch 10"=0.0, "EEG Ch 11"=0.0, "EEG Ch 12"=0.0, "EEG Ch 13"=0.0, "EEG Ch 14"=0.0, "EEG Ch 15"=0.0, "EEG Ch 16"=0.0, "X-Accel"=0, "Y-Accel"=0, "Z-Accel"=0, "X-Gyro"=0, "Y-Gyro"=0, "Z-Gyro"=0, "Timer"=0, "Packet ID"=0, "HW Trig1"=0, "SW Trig1"=0, "HW Trig2"=0, "SW Trig2"=0, "WiBCI Status"={"Mode Byte"=0, "Ch Config"=0, "Ch Ref Map"=0, "Ch Enable Map"=0, "Temperature"=0.0, "Battery"=0, "Version"=""}, "Reg Map"={"ADS1"=[], "ADS2"=[]}}, "En MAP"=0}, Variant=w1150) -> (data=w1141:cluster{"WiBCI16T Data out":T21, "En MAP":u16}, error out=w1149:errorcluster)
            n500 = case shown="250" w1145 {
              selector: w1145 -> [w1157 _]
              tunnel: w1141 -> [w1155 w1159]
              tunnel: w1142 -> [w1158 w1242]
              tunnel: [w1156 w1242] -> w1144
              frame 0, Default {
                n501 = call "Update Impedance.vi"("EEG Data"=w1155, "Numeric"=w1157, "Data Cluster in"=w1158) -> ("Data Cluster out"=w1156:T9)  [unwired: 8 in]
              }
              frame 250 {
                n502 = Unbundle By Name(w1159) -> ("En MAP"=w1245:u16, "WiBCI16T Data out.WiBCI Status.Battery"=w1160:u8)
                n503 = Number To Boolean Array(number=w1245) -> (Boolean array=w1244:bool[])
                n504 = Unbundle By Name(w1242) -> ("Impedance.Ch 1"=w1225:dbl, "Impedance.Ch 2"=w1223:dbl, "Impedance.Ch 3"=w1222:dbl, "Impedance.Ch 4"=w1221:dbl, "Impedance.Ch 5"=w1220:dbl, "Impedance.Ch 6"=w1219:dbl, "Impedance.Ch 7"=w1218:dbl, "Impedance.Ch 8"=w1217:dbl, "Impedance.Ch 9"=w1216:dbl, "Impedance.Ch 10"=w1215:dbl, "Impedance.Ch 11"=w1214:dbl, "Impedance.Ch 12"=w1213:dbl, "Impedance.Ch 13"=w1212:dbl, "Impedance.Ch 14"=w1211:dbl, "Impedance.Ch 15"=w1210:dbl, "Impedance.Ch 16"=w1209:dbl, "Measurement UI Displays.Battery 2"=w1161:refnum<vi>)
                n505 = Index Array(array=w1244, index #1=15 ("index"), index #2=14 ("index"), index #3=13 ("index"), index #4=12 ("index"), index #5=11 ("index"), index #6=10 ("index"), index #7=9 ("index"), index #8=8 ("index"), index #9=7 ("index"), index #10=6 ("index"), index #11=5 ("index"), index #12=4 ("index"), index #13=3 ("index"), index #14=2 ("index"), index #15=1 ("index"), index #16=0 ("index")) -> (element #1=w1193:bool, element #2=w1192:bool, element #3=w1191:bool, element #4=w1190:bool, element #5=w1189:bool, element #6=w1188:bool, element #7=w1187:bool, element #8=w1186:bool, element #9=w1185:bool, element #10=w1184:bool, element #11=w1183:bool, element #12=w1182:bool, element #13=w1181:bool, element #14=w1180:bool, element #15=w1179:bool, element #16=w1178:bool)
                n506 = property class="Slide (strict)"(reference=w1161, "Value"=w1160) -> ()  [unwired: 1 in, 2 out]
                n507 = property on="Imp Ch 9" class="Bool (strict)"("Visible"=w1185) -> ()  [unwired: 2 in, 2 out]
                n508 = property on="Imp Ch 5" class="Bool (strict)"("Visible"=w1189) -> ()  [unwired: 2 in, 2 out]
                n509 = property on="Imp Ch 8" class="Bool (strict)"("Visible"=w1186) -> ()  [unwired: 2 in, 2 out]
                n510 = property on="Imp Ch 1" class="Bool (strict)"("Visible"=w1193) -> ()  [unwired: 2 in, 2 out]
                n511 = property on="Imp Ch 2" class="Bool (strict)"("Visible"=w1192) -> ()  [unwired: 2 in, 2 out]
                n512 = property on="Imp Ch 3" class="Bool (strict)"("Visible"=w1191) -> ()  [unwired: 2 in, 2 out]
                n513 = property on="Imp Ch 4" class="Bool (strict)"("Visible"=w1190) -> ()  [unwired: 2 in, 2 out]
                n514 = property on="Imp Ch 11" class="Bool (strict)"("Visible"=w1183) -> ()  [unwired: 2 in, 2 out]
                n515 = property on="Imp Ch 10" class="Bool (strict)"("Visible"=w1184) -> ()  [unwired: 2 in, 2 out]
                n516 = call "format Impedance display.vi"("Imp Value"=w1213) -> ("decimal integer string"=→"ch 12":string)  [unwired: 10 in]
                n517 = call "format Impedance display.vi"("Imp Value"=w1212) -> ("decimal integer string"=→"ch 13":string)  [unwired: 10 in]
                n518 = call "format Impedance display.vi"("Imp Value"=w1217) -> ("decimal integer string"=→"ch 8":string)  [unwired: 10 in]
                n519 = call "format Impedance display.vi"("Imp Value"=w1214) -> ("decimal integer string"=→"ch 11":string)  [unwired: 10 in]
                n520 = call "format Impedance display.vi"("Imp Value"=w1216) -> ("decimal integer string"=→"ch 9":string)  [unwired: 10 in]
                n521 = call "format Impedance display.vi"("Imp Value"=w1210) -> ("decimal integer string"=→"ch 15":string)  [unwired: 10 in]
                n522 = call "format Impedance display.vi"("Imp Value"=w1209) -> ("decimal integer string"=→"ch 16":string)  [unwired: 10 in]
                n523 = property on="Imp Ch 6" class="Bool (strict)"("Visible"=w1188) -> ()  [unwired: 2 in, 2 out]
                n524 = call "format Impedance display.vi"("Imp Value"=w1215) -> ("decimal integer string"=→"ch 10":string)  [unwired: 10 in]
                n525 = call "format Impedance display.vi"("Imp Value"=w1211) -> ("decimal integer string"=→"ch 14":string)  [unwired: 10 in]
                n526 = call "format Impedance display.vi"("Imp Value"=w1225) -> ("decimal integer string"=→"ch 1":string)  [unwired: 10 in]
                n527 = call "format Impedance display.vi"("Imp Value"=w1223) -> ("decimal integer string"=→"ch 2":string)  [unwired: 10 in]
                n528 = call "format Impedance display.vi"("Imp Value"=w1220) -> ("decimal integer string"=→"ch 5":string)  [unwired: 10 in]
                n529 = call "format Impedance display.vi"("Imp Value"=w1221) -> ("decimal integer string"=→"ch 4":string)  [unwired: 10 in]
                n530 = call "format Impedance display.vi"("Imp Value"=w1219) -> ("decimal integer string"=→"ch 6":string)  [unwired: 10 in]
                n531 = call "format Impedance display.vi"("Imp Value"=w1218) -> ("decimal integer string"=→"ch 7":string)  [unwired: 10 in]
                n532 = call "format Impedance display.vi"("Imp Value"=w1222) -> ("decimal integer string"=→"ch 3":string)  [unwired: 10 in]
                n533 = property on="Imp Ch 7" class="Bool (strict)"("Visible"=w1187) -> ()  [unwired: 2 in, 2 out]
                n534 = property on="Imp Ch 12" class="Bool (strict)"("Visible"=w1182) -> ()  [unwired: 2 in, 2 out]
                n535 = property on="Imp Ch 15" class="Bool (strict)"("Visible"=w1179) -> ()  [unwired: 2 in, 2 out]
                n536 = property on="Imp Ch 16" class="Bool (strict)"("Visible"=w1178) -> ()  [unwired: 2 in, 2 out]
                n537 = property on="Imp Ch 13" class="Bool (strict)"("Visible"=w1181) -> ()  [unwired: 2 in, 2 out]
                n538 = property on="Imp Ch 14" class="Bool (strict)"("Visible"=w1180) -> ()  [unwired: 2 in, 2 out]
                n539 = case shown="50, Default" w1160 {
                  tunnel: [u32 16771090 u32 16723218 u32 6618880] -> w1162
                  frame 50, Default {
                  }
                  frame ..10 {
                  }
                  frame 70.. {
                  }
                }
                n540 = call "color code.vi"("Ch 1"=w1223) -> ("Array"=w1240:cluster{u32, u32}[])  [unwired: 10 in]
                n541 = call "color code.vi"("Ch 1"=w1225) -> ("Array"=w1241:cluster{u32, u32}[])  [unwired: 10 in]
                n542 = call "color code.vi"("Ch 1"=w1219) -> ("Array"=w1236:cluster{u32, u32}[])  [unwired: 10 in]
                n543 = call "color code.vi"("Ch 1"=w1220) -> ("Array"=w1237:cluster{u32, u32}[])  [unwired: 10 in]
                n544 = call "color code.vi"("Ch 1"=w1218) -> ("Array"=w1235:cluster{u32, u32}[])  [unwired: 10 in]
                n545 = call "color code.vi"("Ch 1"=w1221) -> ("Array"=w1238:cluster{u32, u32}[])  [unwired: 10 in]
                n546 = call "color code.vi"("Ch 1"=w1222) -> ("Array"=w1239:cluster{u32, u32}[])  [unwired: 10 in]
                n547 = call "color code.vi"("Ch 1"=w1217) -> ("Array"=w1234:cluster{u32, u32}[])  [unwired: 10 in]
                n548 = call "color code.vi"("Ch 1"=w1215) -> ("Array"=w1232:cluster{u32, u32}[])  [unwired: 10 in]
                n549 = call "color code.vi"("Ch 1"=w1216) -> ("Array"=w1233:cluster{u32, u32}[])  [unwired: 10 in]
                n550 = call "color code.vi"("Ch 1"=w1211) -> ("Array"=w1228:cluster{u32, u32}[])  [unwired: 10 in]
                n551 = call "color code.vi"("Ch 1"=w1212) -> ("Array"=w1229:cluster{u32, u32}[])  [unwired: 10 in]
                n552 = call "color code.vi"("Ch 1"=w1213) -> ("Array"=w1230:cluster{u32, u32}[])  [unwired: 10 in]
                n553 = call "color code.vi"("Ch 1"=w1214) -> ("Array"=w1231:cluster{u32, u32}[])  [unwired: 10 in]
                n554 = call "color code.vi"("Ch 1"=w1209) -> ("Array"=w1226:cluster{u32, u32}[])  [unwired: 10 in]
                n555 = call "color code.vi"("Ch 1"=w1210) -> ("Array"=w1227:cluster{u32, u32}[])  [unwired: 10 in]
                n556 = property on="Property Node" class="Slide (strict)"(reference=w1161, "Fill Color"=w1162) -> ()  [unwired: 1 in, 2 out]
                n557 = property on="ch 5" class="Str"("Visible"=w1189) -> ()  [unwired: 2 in, 2 out]
                n558 = property on="ch 6" class="Str"("Visible"=w1188) -> ()  [unwired: 2 in, 2 out]
                n559 = property on="ch 9" class="Str"("Visible"=w1185) -> ()  [unwired: 2 in, 2 out]
                n560 = property on="ch 10" class="Str"("Visible"=w1184) -> ()  [unwired: 2 in, 2 out]
                n561 = property on="ch 8" class="Str"("Visible"=w1186) -> ()  [unwired: 2 in, 2 out]
                n562 = property on="ch 4" class="Str"("Visible"=w1190) -> ()  [unwired: 2 in, 2 out]
                n563 = property on="ch 7" class="Str"("Visible"=w1187) -> ()  [unwired: 2 in, 2 out]
                n564 = property on="ch 1" class="Str"("Visible"=w1193) -> ()  [unwired: 2 in, 2 out]
                n565 = property on="ch 3" class="Str"("Visible"=w1191) -> ()  [unwired: 2 in, 2 out]
                n566 = property on="ch 11" class="Str"("Visible"=w1183) -> ()  [unwired: 2 in, 2 out]
                n567 = property on="ch 2" class="Str"("Visible"=w1192) -> ()  [unwired: 2 in, 2 out]
                n568 = property on="Imp Ch 13" class="Bool (strict)"("Colors [4]"=w1229) -> ()  [unwired: 2 in, 2 out]
                n569 = property on="Imp Ch 1" class="Bool (strict)"("Colors [4]"=w1241) -> ()  [unwired: 2 in, 2 out]
                n570 = property on="Imp Ch 9" class="Bool (strict)"("Colors [4]"=w1233) -> ()  [unwired: 2 in, 2 out]
                n571 = property on="Imp Ch 11" class="Bool (strict)"("Colors [4]"=w1231) -> ()  [unwired: 2 in, 2 out]
                n572 = property on="Imp Ch 3" class="Bool (strict)"("Colors [4]"=w1239) -> ()  [unwired: 2 in, 2 out]
                n573 = property on="Imp Ch 5" class="Bool (strict)"("Colors [4]"=w1237) -> ()  [unwired: 2 in, 2 out]
                n574 = property on="Imp Ch 7" class="Bool (strict)"("Colors [4]"=w1235) -> ()  [unwired: 2 in, 2 out]
                n575 = property on="Imp Ch 15" class="Bool (strict)"("Colors [4]"=w1227) -> ()  [unwired: 2 in, 2 out]
                n576 = property on="Imp Ch 2" class="Bool (strict)"("Colors [4]"=w1240) -> ()  [unwired: 2 in, 2 out]
                n577 = property on="ch 12" class="Str"("Visible"=w1182) -> ()  [unwired: 2 in, 2 out]
                n578 = property on="ch 14" class="Str"("Visible"=w1180) -> ()  [unwired: 2 in, 2 out]
                n579 = property on="ch 13" class="Str"("Visible"=w1181) -> ()  [unwired: 2 in, 2 out]
                n580 = property on="Imp Ch 12" class="Bool (strict)"("Colors [4]"=w1230) -> ()  [unwired: 2 in, 2 out]
                n581 = property on="ch 16" class="Str"("Visible"=w1178) -> ()  [unwired: 2 in, 2 out]
                n582 = property on="Imp Ch 6" class="Bool (strict)"("Colors [4]"=w1236) -> ()  [unwired: 2 in, 2 out]
                n583 = property on="Imp Ch 10" class="Bool (strict)"("Colors [4]"=w1232) -> ()  [unwired: 2 in, 2 out]
                n584 = property on="Imp Ch 4" class="Bool (strict)"("Colors [4]"=w1238) -> ()  [unwired: 2 in, 2 out]
                n585 = property on="Imp Ch 8" class="Bool (strict)"("Colors [4]"=w1234) -> ()  [unwired: 2 in, 2 out]
                n586 = property on="Imp Ch 14" class="Bool (strict)"("Colors [4]"=w1228) -> ()  [unwired: 2 in, 2 out]
                n587 = property on="ch 15" class="Str"("Visible"=w1179) -> ()  [unwired: 2 in, 2 out]
                n588 = property on="Imp Ch 16" class="Bool (strict)"("Colors [4]"=w1226) -> ()  [unwired: 2 in, 2 out]
              }
            }
            n589 = local write "Data Status"(TRUE) -> ()
          }
          frame "Update_CNV_Display" {
            # "Update CNV Data Display"
            n590 = Variant To Data(error in=w1256, type=cluster{"WiBCI16T Data out":T21, "En MAP":u16} {"WiBCI16T Data out"={"EEG Ch 1"=0.0, "EEG Ch 2"=0.0, "EEG Ch 3"=0.0, "EEG Ch 4"=0.0, "EEG Ch 5"=0.0, "EEG Ch 6"=0.0, "EEG Ch 7"=0.0, "EEG Ch 8"=0.0, "EEG Ch 9"=0.0, "EEG Ch 10"=0.0, "EEG Ch 11"=0.0, "EEG Ch 12"=0.0, "EEG Ch 13"=0.0, "EEG Ch 14"=0.0, "EEG Ch 15"=0.0, "EEG Ch 16"=0.0, "X-Accel"=0, "Y-Accel"=0, "Z-Accel"=0, "X-Gyro"=0, "Y-Gyro"=0, "Z-Gyro"=0, "Timer"=0, "Packet ID"=0, "HW Trig1"=0, "SW Trig1"=0, "HW Trig2"=0, "SW Trig2"=0, "WiBCI Status"={"Mode Byte"=0, "Ch Config"=0, "Ch Ref Map"=0, "Ch Enable Map"=0, "Temperature"=0.0, "Battery"=0, "Version"=""}, "Reg Map"={"ADS1"=[], "ADS2"=[]}}, "En MAP"=0}, Variant=w1257) -> (data=w1255:cluster{"WiBCI16T Data out":T21, "En MAP":u16}, error out=w1254:errorcluster)
            n591 = Unbundle By Name(w1252) -> ("CNV Demo Data.CNV Buffer Action"=w1253:T25, "Measurement UI Displays.Battery 2"=w1249:refnum<vi>)
            n592 = case shown="\"Analyze Buffer\"" w1253 {
              tunnel: w1255 -> [_ w1282 w1287]
              tunnel: w1252 -> [w1259 w1285 w1297]
              tunnel: [w1259 w1283 w1298] -> w1251
              tunnel: w1249 -> [_ _ w1288]
              frame "Stop Buffer Fill", Default {
              }
              frame "Start Buffer Fill" {
                n593 = Unbundle By Name(w1285) -> ("CNV Demo Data.Index of R.Array"=w1280:u16, "CNV Demo Data.Rebuild Vector"=w1281:dbl[][])
                n594 = Unbundle By Name(w1282) -> ("WiBCI16T Data out.EEG Ch 1"=w1279:dbl, "WiBCI16T Data out.EEG Ch 2"=w1278:dbl, "WiBCI16T Data out.EEG Ch 3"=w1277:dbl, "WiBCI16T Data out.EEG Ch 4"=w1276:dbl, "WiBCI16T Data out.EEG Ch 5"=w1275:dbl, "WiBCI16T Data out.EEG Ch 6"=w1274:dbl, "WiBCI16T Data out.EEG Ch 7"=w1273:dbl, "WiBCI16T Data out.EEG Ch 8"=w1272:dbl, "WiBCI16T Data out.EEG Ch 9"=w1271:dbl, "WiBCI16T Data out.EEG Ch 10"=w1270:dbl, "WiBCI16T Data out.EEG Ch 11"=w1269:dbl, "WiBCI16T Data out.EEG Ch 12"=w1268:dbl, "WiBCI16T Data out.EEG Ch 13"=w1267:dbl, "WiBCI16T Data out.EEG Ch 14"=w1266:dbl, "WiBCI16T Data out.EEG Ch 15"=w1265:dbl, "WiBCI16T Data out.EEG Ch 16"=w1264:dbl, "WiBCI16T Data out.SW Trig1"=w1263:i8, "WiBCI16T Data out.Timer"=w1262:u32)
                n595 = Build Array(w1279, w1278, w1277, w1276, w1275, w1274, w1273, w1272, w1271, w1270, w1269, w1268, w1267, w1266, w1265, w1264, w1263, w1262) -> (w1261:dbl[])
                n596 = Insert Into Array(array=w1281, index (row)=w1280, new element=w1261) -> (w1260:dbl[][])  [unwired: 1 in]
                n597 = Increment(x=w1280) -> (x+1=w1284:u16)
                n598 = Bundle By Name(cluster=w1285, "CNV Demo Data.Index of R.Array"=w1284, "CNV Demo Data.Rebuild Vector"=w1260) -> (w1283:T9)
              }
              frame "Analyze Buffer" {
                n599 = Unbundle By Name(w1287) -> ("WiBCI16T Data out.WiBCI Status.Battery"=w1286:u8)
                n600 = Unbundle By Name(w1297) -> ("CNV Demo Data.CNV Iter"=w1296:u16, "CNV Demo Data.Run Sum CNV"=w1294:dbl[])
                n601 = Increment(x=w1296) -> (x+1=w1291:u16)
                n602 = call "Build Draw Vectors.vi"("Data Cluster"=w1297) -> ("Current CNV"=w1293:dbl[])  [unwired: 10 in]
                n603 = Empty Array?(array=w1294) -> (empty?=w1295:bool)
                n604 = property class="Slide (strict)"(reference=w1288, "Value"=w1286) -> (reference out=w1290:refnum<vi>)  [unwired: 1 in, 1 out]
                n605 = case shown="False" w1295 {
                  tunnel: w1294 -> [w1309 _]
                  tunnel: w1293 -> [w1308 w1310]
                  tunnel: [w1306 w1310] -> w1292
                  tunnel: w1291 -> [w1305 _]
                  frame False {
                    n606 = Add(x=w1309, y=w1308) -> (x+y=w1307:dbl[])
                    n607 = Divide(x=w1307, y=w1305) -> (x/y=w1306:dbl[])
                  }
                  frame True {
                  }
                }
                n608 = case shown="50, Default" w1286 {
                  tunnel: [u32 16771090 u32 16723218 u32 6618880] -> w1289
                  frame 50, Default {
                  }
                  frame ..10 {
                  }
                  frame 70.. {
                  }
                }
                n609 = Bundle By Name(cluster=w1297, "CNV Demo Data.CNV Iter"=w1291, "CNV Demo Data.Index of R.Array"=u16 0 ("CNV Demo Controls and Data.Index of R.Array"), "CNV Demo Data.CNV Buffer Action"=T25."Stop Buffer Fill" ("CNV Demo Controls and Data.CNV Buffer Action"), "CNV Demo Data.Run Sum CNV"=w1292) -> (w1298:T9)
                n610 = property on="Property Node" class="Slide (strict)"(reference=w1290, "Fill Color"=w1289) -> ()  [unwired: 1 in, 2 out]
                n611 = Build Array(w1293, w1292) -> (→"CNV Graph":dbl[][])
              }
            }
            n612 = local write "Data Status"(TRUE ("Data Status")) -> ()
          }
          frame "Update_EOC_Display" {
            # "Update CNV Data Display"
            n613 = Variant To Data(error in=w1319, type=cluster{"WiBCI16T Data out":T21, "En MAP":u16} {"WiBCI16T Data out"={"EEG Ch 1"=0.0, "EEG Ch 2"=0.0, "EEG Ch 3"=0.0, "EEG Ch 4"=0.0, "EEG Ch 5"=0.0, "EEG Ch 6"=0.0, "EEG Ch 7"=0.0, "EEG Ch 8"=0.0, "EEG Ch 9"=0.0, "EEG Ch 10"=0.0, "EEG Ch 11"=0.0, "EEG Ch 12"=0.0, "EEG Ch 13"=0.0, "EEG Ch 14"=0.0, "EEG Ch 15"=0.0, "EEG Ch 16"=0.0, "X-Accel"=0, "Y-Accel"=0, "Z-Accel"=0, "X-Gyro"=0, "Y-Gyro"=0, "Z-Gyro"=0, "Timer"=0, "Packet ID"=0, "HW Trig1"=0, "SW Trig1"=0, "HW Trig2"=0, "SW Trig2"=0, "WiBCI Status"={"Mode Byte"=0, "Ch Config"=0, "Ch Ref Map"=0, "Ch Enable Map"=0, "Temperature"=0.0, "Battery"=0, "Version"=""}, "Reg Map"={"ADS1"=[], "ADS2"=[]}}, "En MAP"=0}, Variant=w1320) -> (data=w1313:cluster{"WiBCI16T Data out":T21, "En MAP":u16}, error out=w1311:errorcluster)
            n614 = feedback #4(u8 0) -> (w1316:u8)
            n615 = case shown="10" w1316 {
              selector: w1316 -> [w1323 _]
              tunnel: [w1322 u8 0] -> w1315
              frame 0, Default {
                n616 = Increment(x=w1323) -> (x+1=w1322:u8)
              }
              frame 10 {
              }
            }
            n617 = feedback-in #4(w1315) -> ()
            n618 = case shown="9" w1315 {
              tunnel: w1314 -> [w1340 w1352]
              tunnel: w1313 -> [w1346 w1354]
              tunnel: [w1331 w1348] -> w1312
              frame 9 {
                n619 = Unbundle By Name(w1340) -> ("EOC Demo Data.Running Buffer"=w1341:dbl[], "EOC Demo Data.Index of R.Buffer"=w1336:u8)
                n620 = Unbundle By Name(w1346) -> ("WiBCI16T Data out.EEG Ch 8"=w1339:dbl)
                n621 = Replace Array Subset(array=w1341, new element=w1339, index=w1336) -> (w1337:dbl[])
                n622 = call-poly <vilib>:"Mean.vi"("X"=w1337) -> ("mean"=w1343:dbl)  [unwired: 1 out]
                n623 = Subtract(x=w1337, y=w1343) -> (x-y=w1342:dbl[])
                n624 = Increment(x=w1336) -> (x+1=w1335:u8)
                n625 = Bundle By Name(cluster=waveform(dbl) {"t0"=timestamp(0 s since 1904-01-01), "dt"=1.0, "Y"=[]} ("EEG"), "Y"=w1342, "dt"=0.004) -> (w1338:waveform(dbl))
                n626 = call-poly <vilib>:"EEG FFT Spectrum.vi"("EEG"=w1338) -> ("frequency measurements"=w1334:T32)  [unwired: 8 in, 2 out]
                n627 = Unbundle By Name(w1334) -> ("theta [%]"=→"Theta":dbl, "alpha [%]"=w1330:dbl, "beta [%]"=→"Beta":dbl)
                "Alpha" <- w1330
                n628 = Greater?(x=w1330, y=30.0) -> (0:w1328:bool)
                n629 = Select(t="Eyes Closed", s=w1328, f="Eyes Open") -> (s? t:f=→"Display Label EOC":string)
                n630 = Bundle By Name(cluster=w1340, "EOC Demo Data.Running Buffer"=w1337, "EOC Demo Data.Index of R.Buffer"=w1335) -> (w1331:T9)
              }
              frame 0, Default {
                n631 = Unbundle By Name(w1352) -> ("EOC Demo Data.Running Buffer"=w1353:dbl[], "EOC Demo Data.Index of R.Buffer"=w1350:u8)
                n632 = Unbundle By Name(w1354) -> ("WiBCI16T Data out.EEG Ch 8"=w1351:dbl)
                n633 = Replace Array Subset(array=w1353, new element=w1351, index=w1350) -> (w1347:dbl[])
                n634 = Increment(x=w1350) -> (x+1=w1349:u8)
                n635 = Bundle By Name(cluster=w1352, "EOC Demo Data.Running Buffer"=w1347, "EOC Demo Data.Index of R.Buffer"=w1349) -> (w1348:T9)
              }
            }
            n636 = local write "Data Status"(TRUE ("Data Status")) -> ()
          }
          frame "Clear All Charts" {
            # "All UI Charts are Cleared"
            n637 = Unbundle By Name(w1357) -> ("Measurement UI Displays.Graph 1"=w1356:refnum<vi>, "Measurement UI Displays.Graph 2"=w1375:refnum<vi>, "Measurement UI Displays.Graph 3"=w1374:refnum<vi>, "Measurement UI Displays.Graph 4"=w1373:refnum<vi>, "Measurement UI Displays.Graph 5"=w1372:refnum<vi>, "Measurement UI Displays.Graph 6"=w1371:refnum<vi>, "Measurement UI Displays.Graph 7"=w1370:refnum<vi>, "Measurement UI Displays.Graph 8"=w1369:refnum<vi>, "Measurement UI Displays.Graph 9"=w1368:refnum<vi>, "Measurement UI Displays.Graph 10"=w1367:refnum<vi>, "Measurement UI Displays.Graph 11"=w1366:refnum<vi>, "Measurement UI Displays.Graph 12"=w1365:refnum<vi>, "Measurement UI Displays.Graph 13"=w1364:refnum<vi>, "Measurement UI Displays.Graph 14"=w1363:refnum<vi>, "Measurement UI Displays.Graph 15"=w1362:refnum<vi>, "Measurement UI Displays.Graph 16"=w1361:refnum<vi>, "Measurement UI Displays.Single Chart"=w1355:refnum<vi>, "Measurement UI Displays.Data Trig"=w1359:refnum<vi>)
            n638 = Build Array(w1356, w1375, w1374, w1373, w1372, w1371, w1370, w1369, w1368, w1367, w1366, w1365, w1364, w1363, w1362, w1361, w1355) -> (w1360:refnum<vi>[])
            n639 = property class="WFChart (strict)"(reference=w1359, "History Data"=u8[] []) -> ()  [unwired: 1 in, 2 out]
            n640 = call "Set Graphs to Default.vi"("Array"=w1360) -> ()  [unwired: 11 in]
            n641 = Bundle By Name(cluster=w1357, "Display  cnt"=u8 0) -> (w1377:T9)
          }
          frame "Update Packet Loss (%)" {
            # "Provides Packet Loss in percentage"
            n642 = Variant To Data(error in=w1385, type=T18 {"Paket Loss"=0.0} ("Update Packet Loss (%) Argument"), Variant=w1382) -> (data=w1380:T18, error out=w1383:errorcluster)
            n643 = Unbundle By Name(w1380) -> ("Paket Loss"=→"Packet Loss (%)":dbl)
          }
          frame "---Copy This Frame---" {
            # "Duplicate this frame when creating new messages.  Change this comment in the duplicated frame to describe this message."
            n644 = Merge Errors(w1388) -> (w1387:errorcluster)
          }
          frame "Start Buff Fill" {
            # "Set Conditions to Start Filling Buffer"
            n645 = Merge Errors(w1395) -> (w1394:errorcluster)
            n646 = Bundle By Name(cluster=w1393, "CNV Demo Data.Rebuild Vector"=dbl[][] [] ("CNV Demo Controls and Data.Rebuild Vector"), "CNV Demo Data.CNV Buffer Action"=T25."Start Buffer Fill" ("CNV Demo Controls and Data.CNV Buffer Action"), "CNV Demo Data.Index of R.Array"=u16 0 ("CNV Demo Controls and Data.Index of R.Array")) -> (w1392:T9)
          }
          frame "Stop Buff Fill" {
            # "Set Conditions to Stop Filling Buffer"
            n647 = Merge Errors(w1400) -> (w1399:errorcluster)
            n648 = Bundle By Name(cluster=w1398, "CNV Demo Data.CNV Buffer Action"=T25."Stop Buffer Fill" ("CNV Demo Controls and Data.CNV Buffer Action")) -> (w1397:T9)
          }
          frame "Analyze Buff" {
            # "Set Conditions to Analyze and Graph Buffer"
            n649 = Merge Errors(w1405) -> (w1404:errorcluster)
            n650 = Bundle By Name(cluster=w1403, "CNV Demo Data.CNV Buffer Action"=T25."Analyze Buffer" ("CNV Demo Controls and Data.CNV Buffer Action")) -> (w1402:T9)
          }
          frame "Check WiFi AP" {
            # "Verify the connectivity with the WiFi AP required for this software"
            n651 = call "Check WiFi AP.vi"("error in"=w1406) -> ("error out"=w1407:errorcluster)  [unwired: 10 in]
            n652 = Merge Errors(w1407) -> (w1409:errorcluster)
          }
          frame "Get File Name" {
            # "Gets File Name from Helper Loop (User fed)"
            n653 = Variant To Data(error in=w1418, type=cluster{string, bool} {"", FALSE} ("File Name Out"), Variant=w1417) -> (data=w1413:cluster{string, bool}, error out=w1416:errorcluster)
            n654 = Unbundle(w1413) -> (w1411:string, w1412:bool)
            n655 = case shown="True" w1412 {
              tunnel: w1416 -> [w1423 w1427]
              tunnel: [w1422 w1426] -> w1415
              tunnel: w1411 -> [_ w1425]
              tunnel: w1410 -> [w1421 _]
              frame False {
                n656 = call-poly <vilib>:"Delacor_lib_QMH_Enqueue Message (poly).vi"("error in"=w1423, "Message"="Record Action", "Message Queue in"=w1421) -> ("error out"=w1422:errorcluster)  [unwired: 7 in, 1 out]
              }
              frame True {
                n657 = call "Initialize File.vi"("wait for reply (T)"=FALSE, "error in"=w1427, "file name"=w1425) -> ("error out"=w1426:errorcluster)  [unwired: 6 in, 2 out]
              }
            }
            n658 = Merge Errors(w1415) -> (w1420:errorcluster)
          }
          frame "Settings Updated" {
            # "Display Trig Values"
            # "Display En Ch Names"
            # "Update LSL and Trig Displays"
            # "Settings Module Updated Data"
            n659 = Variant To Data(error in=w1441, type=T26 {"Signal Type"=enum."Sine Wave", "Calibration Array"=[], "Log File Base Path"=path "", "EEG Channels"={"16 EEG Channels"=[], "Gain"=24}, "Soft Trig enum"=enum."Disable Soft Trigger", "Montage selection"={"Montages Ref"=refnum, "Selected Montage Number"=0, "Montages Names"=[]}, "LSL En enum"=enum."LSL Disabled"} ("Settings 2"), Variant=w1440) -> (data=w1438:T26, error out=w1432:errorcluster)
            n660 = Unbundle By Name(w1438) -> ("EEG Channels.16 EEG Channels"=w1437:T31, "Soft Trig enum"=w1435:T33, "LSL En enum"=w1434:enum16{"LSL Disabled", "LSL Enabled"})
            n661 = call "En Setting for Trig and LSL.vi"("LSL En enum"=w1434, "Soft Trig enum"=w1435, "Data Cluster in"=w1433) -> ("Data Cluster out"=w1431:T9)  [unwired: 8 in]
            n662 = call "Display Channel Names (En Only).vi"("Data Cluster"=w1431, "16 EEG Channels"=w1437) -> ("En MAP"=w1429:u16)  [unwired: 9 in]
            n663 = call "Display Soft Trigger Status.vi"("Soft Trig enum"=w1435) -> ("String"=→"En/Dis Trig":string)  [unwired: 10 in]
            n664 = Bundle By Name(cluster=w1431, "Measurement UI Displays.En MAP"=w1429) -> (w1430:T9)
          }
          frame "Impedance Start" {
            # "Starts Impedance Measurement with Ground Loop"
            n665 = call "Start GND Loop acquiring.vi"("error in"=w1443) -> ("error out"=w1442:errorcluster)  [unwired: 10 in]
            n666 = Bundle By Name(cluster=w1446, "Acq State"=Acquisition_State."RUNNING") -> (w1444:T9)
            n667 = call-poly <vilib>:"Delacor_lib_QMH_Enqueue Message (poly).vi"("error in"=w1442, "Message"="Impedance Started Interlocks", "Message Queue in"=w1447) -> ("error out"=w1448:errorcluster)  [unwired: 7 in, 1 out]
            n668 = Merge Errors(w1448) -> (w1450:errorcluster)
          }
          frame "Gnd Imp to Imp mode" {
            # "Shift from Gnd loop Impedance to Impedance Mode"
            n669 = Variant To Data(error in=w1455, type=TRUE, Variant=w1452) -> (data=w1451:bool, error out=w1454:errorcluster)
            n670 = case shown="False" w1451 {
              tunnel: [w1461 w1464] -> w1456
              tunnel: w1454 -> [w1462 w1463]
              frame False {
                n671 = call "Start GND Loop acquiring.vi"("error in"=w1462) -> ("error out"=w1461:errorcluster)  [unwired: 10 in]
              }
              frame True {
                n672 = call "Start IMP Acquiring.vi"("error in"=w1463) -> ("error out"=w1464:errorcluster)  [unwired: 10 in]
              }
            }
            n673 = Bundle By Name(cluster=w1459, "Acq State"=Acquisition_State."RUNNING", "Imp Mode"=w1451) -> (w1457:T9)
            n674 = Merge Errors(w1456) -> (w1460:errorcluster)
          }
          frame "Start EOC Demo" {
            # "Starts EOC Demo"
            n675 = call "Set Eyes OC Montage.vi"("error in"=w1468) -> ("error out"=w1467:errorcluster)  [unwired: 10 in]
            n676 = call-poly <userlib>:"MGI Wait.vi"("ms"=u32 2, "Error In"=w1467) -> ("Error Out"=w1466:errorcluster)  [unwired: 5 in]
            n677 = call "Start EOC Acquiring.vi"("error in"=w1466) -> ("error out"=w1471:errorcluster)  [unwired: 10 in]
            n678 = Bundle By Name(cluster=w1474, "Acq State"=Acquisition_State."RUNNING", "EOC Demo Data.Running Buffer"=dbl[] [0.0, 0.0, 0.0, 0.0, 0.0, 0.0, 0.0, 0.0, 0.0, 0.0, 0.0, 0.0, 0.0, 0.0, 0.0, 0.0, 0.0, 0.0, 0.0, 0.0, 0.0, 0.0, 0.0, 0.0, 0.0, 0.0, 0.0, 0.0, 0.0, 0.0, 0.0, 0.0, 0.0, 0.0, 0.0, 0.0, 0.0, 0.0, 0.0, 0.0, 0.0, 0.0, 0.0, 0.0, 0.0, 0.0, 0.0, 0.0, 0.0, 0.0, 0.0, 0.0, 0.0, 0.0, 0.0, 0.0, 0.0, 0.0, 0.0, 0.0, 0.0, 0.0, 0.0, 0.0, 0.0, 0.0, 0.0, 0.0, 0.0, 0.0, 0.0, 0.0, 0.0, 0.0, 0.0, 0.0, 0.0, 0.0, 0.0, 0.0, 0.0, 0.0, 0.0, 0.0, 0.0, 0.0, 0.0, 0.0, 0.0, 0.0, 0.0, 0.0, 0.0, 0.0, 0.0, 0.0, 0.0, 0.0, 0.0, 0.0, 0.0, 0.0, 0.0, 0.0, 0.0, 0.0, 0.0, 0.0, 0.0, 0.0, 0.0, 0.0, 0.0, 0.0, 0.0, 0.0, 0.0, 0.0, 0.0, 0.0, 0.0, 0.0, 0.0, 0.0, 0.0, 0.0, 0.0, 0.0, 0.0, 0.0, 0.0, 0.0, 0.0, 0.0, 0.0, 0.0, 0.0, 0.0, 0.0, 0.0, 0.0, 0.0, 0.0, 0.0, 0.0, 0.0, 0.0, 0.0, 0.0, 0.0, 0.0, 0.0, 0.0, 0.0, 0.0, 0.0, 0.0, 0.0, 0.0, 0.0, 0.0, 0.0, 0.0, 0.0, 0.0, 0.0, 0.0, 0.0, 0.0, 0.0, 0.0, 0.0, 0.0, 0.0, 0.0, 0.0, 0.0, 0.0, 0.0, 0.0, 0.0, 0.0, 0.0, 0.0, 0.0, 0.0, 0.0, 0.0, 0.0, 0.0, 0.0, 0.0, 0.0, 0.0, 0.0, 0.0, 0.0, 0.0, 0.0, 0.0, 0.0, 0.0, 0.0, 0.0, 0.0, 0.0, 0.0, 0.0, 0.0, 0.0, 0.0, 0.0, 0.0, 0.0, 0.0, 0.0, 0.0, 0.0, 0.0, 0.0, 0.0, 0.0, 0.0, 0.0, 0.0, 0.0, 0.0, 0.0, 0.0, 0.0, 0.0, 0.0, 0.0, 0.0, 0.0, 0.0, 0.0, 0.0, 0.0, 0.0, 0.0, 0.0, 0.0, 0.0, 0.0, 0.0, 0.0, 0.0, 0.0, 0.0, 0.0, 0.0, 0.0, 0.0, 0.0, 0.0, 0.0, 0.0, 0.0, 0.0, 0.0, 0.0, 0.0, 0.0, 0.0, 0.0, 0.0, 0.0, 0.0, 0.0, 0.0, 0.0, 0.0, 0.0, 0.0, 0.0, 0.0, 0.0, 0.0, 0.0, 0.0, 0.0, 0.0, 0.0, 0.0, 0.0, 0.0, 0.0, 0.0, 0.0, 0.0, 0.0, 0.0, 0.0, 0.0, 0.0, 0.0, 0.0, 0.0, 0.0, 0.0, 0.0, 0.0, 0.0, 0.0, 0.0, 0.0, 0.0, 0.0, 0.0, 0.0, 0.0, 0.0, 0.0, 0.0, 0.0, 0.0, 0.0, 0.0, 0.0, 0.0, 0.0, 0.0, 0.0, 0.0, 0.0, 0.0, 0.0, 0.0, 0.0, 0.0, 0.0, 0.0, 0.0, 0.0, 0.0, 0.0, 0.0, 0.0, 0.0, 0.0, 0.0, 0.0, 0.0, 0.0, 0.0, 0.0, 0.0, 0.0, 0.0, 0.0, 0.0, 0.0, 0.0, 0.0, 0.0, 0.0, 0.0, 0.0, 0.0, 0.0, 0.0, 0.0, 0.0, 0.0, 0.0, 0.0, 0.0, 0.0, 0.0, 0.0, 0.0, 0.0, 0.0, 0.0, 0.0, 0.0, 0.0, 0.0, 0.0, 0.0, 0.0, 0.0, 0.0, 0.0, 0.0, 0.0, 0.0, 0.0, 0.0, 0.0, 0.0, 0.0, 0.0, 0.0, 0.0, 0.0, 0.0, 0.0, 0.0, 0.0, 0.0, 0.0, 0.0, 0.0, 0.0, 0.0, 0.0, 0.0, 0.0, 0.0, 0.0, 0.0, 0.0, 0.0, 0.0, 0.0, 0.0, 0.0, 0.0, 0.0, 0.0, 0.0, 0.0, 0.0, 0.0, 0.0, 0.0, 0.0, 0.0, 0.0, 0.0, 0.0, 0.0, 0.0, 0.0, 0.0, 0.0, 0.0, 0.0, 0.0, 0.0, 0.0, 0.0, 0.0, 0.0, 0.0, 0.0, 0.0, 0.0, 0.0, 0.0, 0.0, 0.0, 0.0, 0.0, 0.0, 0.0, 0.0, 0.0, 0.0, 0.0, 0.0, 0.0, 0.0, 0.0, 0.0, 0.0, 0.0, 0.0, 0.0, 0.0, 0.0, 0.0, 0.0, 0.0, 0.0, 0.0, 0.0, 0.0, 0.0, 0.0, 0.0, 0.0, 0.0, 0.0, 0.0, 0.0, 0.0, 0.0, 0.0, 0.0, 0.0, 0.0, 0.0, 0.0, 0.0, 0.0, 0.0, 0.0, 0.0, 0.0, 0.0, 0.0, 0.0, 0.0, 0.0, 0.0, 0.0, 0.0, 0.0, 0.0, 0.0, 0.0, 0.0, 0.0, 0.0, 0.0, 0.0, 0.0, 0.0, 0.0, 0.0, 0.0, 0.0, 0.0, 0.0, 0.0, 0.0, 0.0, 0.0, 0.0, 0.0, 0.0, 0.0, 0.0, 0.0, 0.0, 0.0, 0.0, 0.0, 0.0, 0.0, 0.0, 0.0, 0.0, 0.0, 0.0, 0.0, 0.0, 0.0, 0.0, 0.0, 0.0, 0.0, 0.0, 0.0, 0.0, 0.0, 0.0, 0.0, 0.0, 0.0, 0.0, 0.0, 0.0, 0.0, 0.0, 0.0, 0.0, 0.0, 0.0, 0.0, 0.0, 0.0, 0.0, 0.0, 0.0, 0.0, 0.0, 0.0, 0.0, 0.0, 0.0, 0.0, 0.0, 0.0, 0.0, 0.0, 0.0, 0.0, 0.0, 0.0, 0.0, 0.0, 0.0, 0.0, 0.0, 0.0, 0.0, 0.0, 0.0, 0.0, 0.0, 0.0, 0.0, 0.0, 0.0, 0.0, 0.0, 0.0, 0.0, 0.0, 0.0, 0.0, 0.0, 0.0, 0.0, 0.0, 0.0, 0.0, 0.0, 0.0, 0.0, 0.0, 0.0, 0.0, 0.0, 0.0, 0.0, 0.0, 0.0, 0.0, 0.0, 0.0, 0.0, 0.0, 0.0, 0.0, 0.0, 0.0, 0.0, 0.0, 0.0, 0.0, 0.0, 0.0, 0.0, 0.0, 0.0, 0.0, 0.0, 0.0, 0.0, 0.0, 0.0, 0.0, 0.0, 0.0, 0.0, 0.0, 0.0, 0.0, 0.0, 0.0, 0.0, 0.0, 0.0, 0.0, 0.0, 0.0, 0.0, 0.0, 0.0, 0.0, 0.0, 0.0, 0.0, 0.0, 0.0, 0.0, 0.0, 0.0, 0.0, 0.0, 0.0, 0.0, 0.0, 0.0, 0.0, 0.0, 0.0, 0.0, 0.0, 0.0, 0.0, 0.0, 0.0, 0.0, 0.0, 0.0, 0.0, 0.0, 0.0, 0.0, 0.0, 0.0, 0.0, 0.0, 0.0, 0.0, 0.0, 0.0, 0.0, 0.0, 0.0, 0.0, 0.0, 0.0, 0.0, 0.0, 0.0, 0.0, 0.0, 0.0, 0.0, 0.0, 0.0, 0.0, 0.0, 0.0, 0.0, 0.0, 0.0, 0.0, 0.0, 0.0, 0.0, 0.0, 0.0, 0.0, 0.0, 0.0, 0.0, 0.0, 0.0, 0.0, 0.0, 0.0, 0.0, 0.0, 0.0, 0.0, 0.0, 0.0, 0.0, 0.0, 0.0, 0.0, 0.0, 0.0, 0.0, 0.0, 0.0, 0.0, 0.0, 0.0, 0.0, 0.0, 0.0, 0.0, 0.0, 0.0, 0.0, 0.0, 0.0, 0.0, 0.0, 0.0, 0.0, 0.0, 0.0, 0.0, 0.0, 0.0, 0.0, 0.0, 0.0, 0.0, 0.0, 0.0, 0.0, 0.0, 0.0, 0.0, 0.0, 0.0, 0.0, 0.0, 0.0, 0.0, 0.0, 0.0, 0.0, 0.0, 0.0, 0.0, 0.0, 0.0, 0.0, 0.0, 0.0, 0.0, 0.0, 0.0, 0.0, 0.0, 0.0, 0.0, 0.0, 0.0, 0.0, 0.0, 0.0, 0.0, 0.0, 0.0, 0.0, 0.0, 0.0, 0.0, 0.0, 0.0, 0.0, 0.0, 0.0, 0.0, 0.0, 0.0, 0.0, 0.0, 0.0, 0.0, 0.0, 0.0, 0.0, 0.0, 0.0, 0.0, 0.0, 0.0, 0.0, 0.0, 0.0, 0.0, 0.0, 0.0, 0.0, 0.0, 0.0, 0.0, 0.0, 0.0, 0.0, 0.0, 0.0, 0.0, 0.0, 0.0, 0.0, 0.0, 0.0, 0.0, 0.0, 0.0, 0.0, 0.0, 0.0, 0.0, 0.0, 0.0, 0.0, 0.0, 0.0, 0.0, 0.0, 0.0, 0.0, 0.0, 0.0, 0.0, 0.0, 0.0, 0.0, 0.0, 0.0, 0.0, 0.0, 0.0, 0.0, 0.0, 0.0, 0.0, 0.0, 0.0, 0.0, 0.0, 0.0, 0.0, 0.0, 0.0, 0.0, 0.0, 0.0, 0.0, 0.0, 0.0, 0.0, 0.0, 0.0, 0.0, 0.0, 0.0, 0.0, 0.0, 0.0, 0.0, 0.0, 0.0, 0.0, 0.0, 0.0, 0.0, 0.0, 0.0, 0.0, 0.0, 0.0, 0.0, 0.0, 0.0, 0.0, 0.0, 0.0, 0.0, 0.0, 0.0, 0.0, 0.0, 0.0, 0.0, 0.0, 0.0, 0.0, 0.0, 0.0, 0.0, 0.0, 0.0, 0.0, 0.0, 0.0, 0.0, 0.0, 0.0, 0.0, 0.0, 0.0, 0.0, 0.0, 0.0, 0.0, 0.0, 0.0, 0.0, 0.0, 0.0, 0.0, 0.0, 0.0, 0.0, 0.0, 0.0, 0.0, 0.0, 0.0, 0.0, 0.0, 0.0, 0.0, 0.0, 0.0, 0.0, 0.0, 0.0, 0.0, 0.0, 0.0, 0.0, 0.0], "EOC Demo Data.Index of R.Buffer"=u8 0) -> (w1472:T9)
            n679 = call-poly <vilib>:"Delacor_lib_QMH_Enqueue Message (poly).vi"("error in"=w1471, "Message"="EOC Started Interlocks", "Message Queue in"=w1475) -> ("error out"=w1476:errorcluster)  [unwired: 7 in, 1 out]
            n680 = Merge Errors(w1476) -> (w1478:errorcluster)
          }
          frame "Start CNV Demo" {
            # "Wait for command from Helper Loop to Start Filling"
            # "CNV Demo Started."
            n681 = call "Wake-up CNV Demo Loop.vi"("error in"=w1483) -> ("error out"=w1482:errorcluster)  [unwired: 10 in]
            n682 = Bundle By Name(cluster=w1486, "CNV Demo Data.Run Sum CNV"=dbl[] [] ("CNV Demo Controls and Data.Rebuild Vector"), "CNV Demo Data.CNV Iter"=u16 0 ("CNV Demo Controls and Data.CNV Iter"), "Acq State"=Acquisition_State."RUNNING", "CNV Demo Data.CNV Buffer Action"=T25."Stop Buffer Fill" ("CNV Demo Controls and Data.CNV Buffer Action")) -> (w1484:T9)
            n683 = call-poly <vilib>:"Delacor_lib_QMH_Enqueue Message (poly).vi"("error in"=w1482, "Message"="CNV Started Interlocks", "Message Queue in"=w1487) -> ("error out"=w1488:errorcluster)  [unwired: 7 in, 1 out]
            n684 = Merge Errors(w1488) -> (w1490:errorcluster)
          }
          frame "Stop CNV Demo" {
            # "CNV Demo Stopped."
            n685 = call "Sleep CNV Demo Loop.vi"("error in"=w1492) -> ("error out"=w1491:errorcluster)  [unwired: 10 in]
            n686 = Bundle By Name(cluster=w1495, "Acq State"=Acquisition_State."IDLE") -> (w1493:T9)
            n687 = call-poly <vilib>:"Delacor_lib_QMH_Enqueue Message (poly).vi"("error in"=w1491, "Message"="CNV Stopped Interlocks", "Message Queue in"=w1496) -> ("error out"=w1497:errorcluster)  [unwired: 7 in, 1 out]
            n688 = Merge Errors(w1497) -> (w1499:errorcluster)
          }
          frame "Start Rec Impedance" {
            # "Start Impedance for Ref or Rec conditions"
            n689 = Variant To Data(error in=w1505, type=TRUE, Variant=w1504) -> (data=w1502:bool, error out=w1501:errorcluster)
            n690 = case shown="True" w1502 {
              tunnel: w1501 -> [w1509 w1511]
              tunnel: [w1508 w1510] -> w1500
              frame False {
                n691 = call "Start GND Loop acquiring.vi"("error in"=w1509) -> ("error out"=w1508:errorcluster)  [unwired: 10 in]
              }
              frame True {
                n692 = call "Command_ImpedanceData.vi"("error in"=w1511) -> ("error out"=w1510:errorcluster)  [unwired: 10 in]
              }
            }
            n693 = Merge Errors(w1500) -> (w1507:errorcluster)
          }
          frame "Trigger Action" {
            # "Send the Keyboard Marker\nto LSL Stream"
            # "Send Soft Trigger (Keyboard) to Acquisition System"
            n694 = Variant To Data(error in=w1521, type=i16 0 ("Char"), Variant=w1520) -> (data=w1512:i16, error out=w1514:errorcluster)
            n695 = Unbundle By Name(w1518) -> ("En/Dis Trig"=w1516:refnum<vi>, "Soft Trigger En?"=w1517:bool)
            n696 = call "KeyBoard Trigger.vi"("error in"=w1514, "Keyboard Trig"=w1512) -> ("error out"=w1513:errorcluster)  [unwired: 9 in]
            n697 = case shown="True" w1517 {
              tunnel: w1516 -> [_ w1531]
              tunnel: [w1522 w1528] -> w1515
              tunnel: w1513 -> [w1522 w1527]
              tunnel: w1512 -> [_ w1526]
              frame False {
              }
              frame True {
                w1524 = "\""
                w1525 = "\n"
                n698 = Build Array(w1526) -> (w1536:i16[])
                n699 = To Unsigned Byte Integer(number=w1536) -> (unsigned 8bit integer=w1535:u8[])
                n700 = Byte Array To String(unsigned byte array=w1535) -> (string=w1532:string)
                n701 = Concatenate Strings("Soft Trigger" ("string"), w1525, "ENABLED" ("string"), w1525, w1525, w1524, w1532, w1524) -> (w1529:string)
                n702 = call "Soft Trigger.vi"("error in"=w1527, "Value"=w1526) -> ("error out"=w1523:errorcluster)  [unwired: 9 in]
                n703 = invoke class="Str" method="Reinit To Default"(reference=w1531) -> (reference out=w1530:refnum<vi>)  [unwired: 2 in, 2 out]
                n704 = Merge Errors(w1523) -> (w1528:errorcluster)
                n705 = invoke class="Str" method="Append String"(reference=w1530, "string"=w1529) -> ()  [unwired: 2 in, 4 out]
              }
            }
          }
          frame "Graph Mouse Action" {
            # "Zoom In/Out selected graphs"
            # "Mouse click to Zoom in/out clicked graph"
            n706 = Variant To Data(error in=w1546, type="", Variant=w1545) -> (data=w1542:string, error out=w1539:errorcluster)
            n707 = call "Zoom in-out Graphs to mouse selection.vi"("String"=w1542, "Data Cluster in"=w1541) -> ("Clear Graph ?"=w1537:bool, "Data Cluster out"=w1543:T9)  [unwired: 8 in]
            n708 = case shown="False" w1537 {
              tunnel: w1540 -> [_ w1551]
              tunnel: w1539 -> [w1547 w1549]
              tunnel: [w1547 w1548] -> w1538
              frame False {
              }
              frame True {
                n709 = call-poly <vilib>:"Delacor_lib_QMH_Enqueue Message (poly).vi"("error in"=w1549, "Message"="Clear All Charts", "Message Queue in"=w1551) -> ("error out"=w1548:errorcluster)  [unwired: 7 in, 1 out]
              }
            }
          }
          frame "---Exit and Error Handling---" {
            # "Separator - The following cases handle errors and exit messages."
          }
          frame "Error" {
            # "Error - Check the error message data and respond accordingly. This message is sent by the \"Error Handler\" VIs at the end of each loop in this application."
            n710 = property on="Property Node" class="Module Admin"(reference=w1555) -> ("Accessors:External Launch"=w1554:bool)  [unwired: 1 in, 2 out]
            n711 = Variant To Data(error in=w1563, type=errorcluster {"status"=FALSE, "code"=0, "source"=""} ("error constant"), Variant=w1557) -> (data=w1564:errorcluster, error out=w1561:errorcluster)
            n712 = call "Error Reported.vi"("Error"=w1564) -> ()  [unwired: 10 in, 1 out]
            n713 = case shown="False" w1554 {
              tunnel: [w1569 _] -> w1560
              tunnel: w1556 -> [w1567 _]
              tunnel: w1564 -> [w1568 _]
              frame False {
                # "If the module is running standalone, then pop up an error dialog and call the \"Exit\" message."
                n714 = call <vilib>:"Simple Error Handler.vi"("error in (no error)"=w1568) -> ()  [unwired: 4 in, 5 out]
                n715 = call-poly <vilib>:"Delacor_lib_QMH_Enqueue Message (poly).vi"("Priority Message? (F)"=TRUE, "Message"="Exit", "Message Queue in"=w1567) -> ("error out"=w1569:errorcluster)  [unwired: 7 in, 1 out]
              }
              frame True {
                # "If the module was launched externally, calling the Error Reported broadcast VI is the only action performed by the \"Error\" message. The module's caller can then process the error appropriately."
              }
            }
            n716 = Merge Errors(w1561, w1560) -> (w1559:errorcluster)
            n717 = local write "error out"(w1559) -> ()
          }
          frame "Exit" {
            w1582 = 91  # 91: not all Exit messages will have an argument
            # "Exit - Exit the application. (conditional)"
            n718 = Variant To Data(error in=w1587, type=T13 {"Origin"="", "Exit via Stop Module Req?"=FALSE, "Wait for Module to stop?"=FALSE} ("Stop Argument"), Variant=w1583) -> (data=w1580:T13, error out=w1585:errorcluster)
            n719 = Unbundle By Name(w1576) -> ("Acq State"=w1575:T10)
            n720 = call <vilib>:"Clear Errors.vi"("error in (no error)"=w1585, "specific error code to clear (0: all)"=w1582) -> ("error out"=w1586:errorcluster)  [unwired: 4 in, 1 out]
            n721 = case shown="\"IDLE\", Default" w1575 {
              tunnel: w1586 -> [w1589 w1606]
              tunnel: w1584 -> [_ w1603]
              tunnel: w1580 -> [_ w1602]
              tunnel: w1579 -> [_ w1600]
              tunnel: [w1589 w1591] -> w1578
              tunnel: w1577 -> [_ w1599]
              tunnel: [FALSE w1598] -> w1574
              tunnel: w1573 -> [_ w1596]
              tunnel: w1572 -> [_ w1595]
              tunnel: w1571 -> [_ w1594]
              tunnel: w1570 -> [_ w1593]
              frame "RUNNING" {
                # "Ignore Event during Acquisition"
              }
              frame "IDLE", Default {
                w1598 = TRUE  # Stop the VI
                w1597 = TRUE ("Wait for Module to Stop? (F)")
                # "Release the message queue reference"
                n722 = control-ref of="This VI"() -> (w1601:refnum<vi>)
                n723 = call "Module Name--constant.vi"() -> ("Module Name"=w1592:string)  [unwired: 11 in]
                n724 = call "Handle Exit.vi"("Stop Argument"=w1602, "Admin in"=w1600, "VI reference"=w1601) -> ("error out"=w1604:errorcluster)  [unwired: 7 in, 1 out]
                n725 = call-dynamic "Delacor_lib_QMH_Release Message Queue.vi"("error in"=w1606, "Message Queue"=w1603) -> ("error out"=w1605:errorcluster)  [unwired: 9 in]
                n726 = Merge Errors(w1605, w1604) -> (w1591:errorcluster)
                n727 = call <vilib>:"Clear Errors.vi"("error in (no error)"=w1591) -> ("error out"=w1590:errorcluster)  [unwired: 5 in, 1 out]
                n728 = case shown="False" w1596 {
                  tunnel: w1597 -> [w1618 _]
                  tunnel: w1592 -> [w1617 _]
                  tunnel: w1590 -> [w1616 _]
                  frame False {
                    n729 = call "Stop Module.vi"("error in"=w1616, "Wait for Module to Stop? (F)"=w1618, "Origin"=w1617) -> ()  [unwired: 8 in, 1 out]
                  }
                  frame True {
                  }
                }
                n730 = case shown="False" w1595 {
                  tunnel: w1597 -> [w1615 _]
                  tunnel: w1592 -> [w1614 _]
                  tunnel: w1590 -> [w1613 _]
                  frame False {
                    n731 = call "Stop Module.vi"("error in"=w1613, "Wait for Module to Stop? (F)"=w1615, "Origin"=w1614) -> ()  [unwired: 8 in, 1 out]
                  }
                  frame True {
                  }
                }
                n732 = case shown="False" w1599 {
                  tunnel: w1590 -> [w1621 _]
                  tunnel: w1597 -> [w1620 _]
                  tunnel: w1592 -> [w1619 _]
                  frame False {
                    n733 = call "Stop Module.vi"("error in"=w1621, "Wait for Module to Stop? (F)"=w1620, "Origin"=w1619) -> ()  [unwired: 8 in, 1 out]
                  }
                  frame True {
                  }
                }
                n734 = case shown="False" w1594 {
                  tunnel: w1597 -> [w1612 _]
                  tunnel: w1592 -> [w1611 _]
                  tunnel: w1590 -> [w1610 _]
                  frame False {
                    n735 = call "Stop Module.vi"("error in"=w1610, "Wait for Module to Stop? (F)"=w1612, "Origin"=w1611) -> ()  [unwired: 8 in, 1 out]
                  }
                  frame True {
                  }
                }
                n736 = case shown="False" w1593 {
                  tunnel: w1597 -> [w1609 _]
                  tunnel: w1592 -> [w1608 _]
                  tunnel: w1590 -> [w1607 _]
                  frame False {
                    n737 = call "Stop Module.vi"("error in"=w1607, "Wait for Module to Stop? (F)"=w1609, "Origin"=w1608) -> ()  [unwired: 8 in, 1 out]
                  }
                  frame True {
                  }
                }
              }
            }
            n738 = call "Error Reported.vi"("Error"=w1578) -> ()  [unwired: 10 in, 1 out]
          }
          frame Default {
            # "'Default' case only runs if there is a message that isn't defined in any of the other cases.  Output a programming error."
            n739 = call "Module Name--constant.vi"() -> ("Module Name"=w1622:string)  [unwired: 11 in]
            n740 = xnode ("Error Ring")("parameter 0"=w1623, "parameter 1"=w1622) -> ("error out"=w1627:errorcluster)
            n741 = Merge Errors(w1625, w1627) -> (w1626:errorcluster)
          }
        }
        n742 = call-dynamic "Delacor_lib_QMH_Error Handler - Message Handling Loop.vi"("error in"=w501, "Message Queue in"=w492) -> ("dup error in"=w498:errorcluster)  [unwired: 8 in, 1 out]
      }
      n743 = while "DQMH_HELPER_LOOP" {
        shift-right: [w186] -> _
        shift-left: -1 -> [w185]
        shift-right: [w183] -> w66
        shift-left: w65 -> [w184]
        tunnel: w70 -> [w180]
        stop <- w182 stop-if-true
        w179 = "File Name Query Loop"  # DQMH_HELPER_LOOP_NAME
        # "File Name Query Loop"
        n744 = event "DQMH_HELPER_EVENT_STRUCTURE" shown="[2] <CML UI Request Events.Private.Wake-Up File Name Query Loop>: User Event" {
          selector: w184 -> [_ _ _ _ _]
          dyn-events: [_ _ _ _ _] -> w183
          timeout: w185 -> [_ _ _ _ _]
          tunnel: w185 -> [w187 w190 w196 w198 w209]
          tunnel: [w187 w190 w196 w198 w209] -> w186
          tunnel: [_ TRUE _ _ _] -> w182
          tunnel: [_ errorcluster {"status"=FALSE, "code"=0, "source"=""} ("error constant") w192 w197 w200] -> w181
          tunnel: w180 -> [_ _ w194 _ _]
          event Timeout {
            n745 = event-data() -> ()  [unwired: 1 in, 1 out]
          }
          event User Event {
            n746 = event-data() -> ()  [unwired: 1 in, 1 out]
          }
          event User Event {
            # "Keep the Module Sleeping !!!\nNeeded to Call Dialogue Asynchronously"
            # "This module called the \"Private.Wake-Up File Name Query Loop\" private request."
            n747 = event-data() -> ()  [unwired: 1 in, 1 out]
            n748 = call "File Name Message.vi"() -> ("error out"=w193:errorcluster, "File Name Out"=w191:cluster{string, bool})  [unwired: 10 in]
            n749 = call-poly <vilib>:"Delacor_lib_QMH_Enqueue Message (poly).vi"("error in"=w193, "Message Data"=w191, "Message"="Get File Name", "Message Queue in"=w194) -> ("error out"=w192:errorcluster)  [unwired: 6 in, 1 out]
          }
          event User Event {
            # "This module called the \"Private.Menu -- About Display Box\" private request."
            n750 = event-data() -> ()  [unwired: 1 in, 1 out]
            n751 = call "Menu -- About Display.vi"() -> ("error out"=w197:errorcluster)  [unwired: 11 in]
          }
          event User Event {
            w207 = T34 2 items=["User Home"=0, "User Desktop"=1, "User Documents"=2, "User Application Data"=3, "User Preferences"=4, "User Temporary"=5, "Public Documents"=6, "Public Application Data"=7, "Public Preferences"=8, "Public Cache"=13, "System Core Libraries"=9, "System Installed Libraries"=10, "Application Files"=11, "Boot Volume Root"=12] ("system directory type")
            # "This module called the \"Private.Wake-Up Copy MATLAB files\" private request."
            n752 = event-data() -> ()  [unwired: 1 in, 1 out]
            n753 = disable-structure "Conditional Disable Structure" shown="RUN_TIME_ENGINE==True&&OS==Win" {
              disable-tunnel: [w211 w215] -> w199
              frame condition #0 (active) {
                n754 = call <vilib>:"Application Directory.vi"() -> ("Application Directory"=w214:path)
                n755 = Build Path(base path=w214, name or relative path="TestFiles") -> (appended path=w210:path)
                n756 = Build Path(base path=w210, name or relative path="wibci2eeglab.zip") -> (appended path=w211:path)
              }
              frame condition #1 {
                n757 = call <vilib>:"Application Directory.vi"() -> ("Application Directory"=w219:path)
                n758 = Build Path(base path=w219, name or relative path="data") -> (appended path=w217:path)
                n759 = Build Path(base path=w217, name or relative path="wibci2eeglab.zip") -> (appended path=w215:path)
              }
            }
            n760 = call <vilib>:"Get System Directory.vi"("system directory type"=w207) -> ("system directory"=w206:path)  [unwired: 10 in]
            n761 = call "File Dialog"("start path"=w206) -> ("selected path"=w204:path, "error out"=w201:errorcluster)  [unwired: 11 in, 2 out]
            n762 = call <vilib>:"Check if File or Folder Exists.vi"("path"=w204) -> ("file or folder exists?"=w205:bool)  [unwired: 8 in, 2 out]
            n763 = Strip Path(path=w204) -> (stripped path=w203:path)  [unwired: 1 out]
            n764 = Select(t=w204, s=w205, f=w203) -> (s? t:f=w202:path)
            n765 = call <userlib>:"Copy with Options__ogtk.vi"("error in (no error)"=w201, "Replace Mode (Never)"=enum16{"Never", "Always", "If Newer"}."Never", "target path"=w202, "source path"=w199) -> ("error out"=w200:errorcluster)  [unwired: 6 in, 1 out]
          }
        }
        n766 = call-dynamic "Delacor_lib_QMH_Error Handler - Helper Loop.vi"("Error Debug"=w179, "error in"=w181, "Message Queue in"=w180) -> ()  [unwired: 7 in, 2 out]
      }
      n767 = while "DQMH_HELPER_LOOP" {
        shift-right: [w86] -> _
        shift-left: -1 -> [w85]
        shift-right: [w83] -> w62
        shift-left: w61 -> [w84]
        tunnel: w70 -> [w80]
        shift-right: [w77] -> _
        shift-left: T8 {"Visual Cue Tab"=refnum, "Display CNV Tab"=refnum, "Visual Cue Graph"=refnum, "CNV Runner"={"fixed array"=[], "Loop Counter"=0}, "CNV Graph"=refnum} ("CNV demo Helper Loop Data") -> [w78]
        stop <- w82 stop-if-true
        w79 = "CNV Demo UI Loop"  # DQMH_HELPER_LOOP_NAME
        # "CNV Demo UI Loop"
        n768 = event "DQMH_HELPER_EVENT_STRUCTURE" shown="[3] <CML UI Request Events.Private.Sleep CNV Demo Loop>: User Event" {
          selector: w84 -> [_ _ _ _]
          dyn-events: [_ _ _ _] -> w83
          timeout: w85 -> [_ _ _ _]
          tunnel: w85 -> [w97 w146 _ _]
          tunnel: [w97 w146 0 -1] -> w86
          tunnel: [_ TRUE _ _] -> w82
          tunnel: [_ errorcluster {"status"=FALSE, "code"=0, "source"=""} ("error constant") w152 w168] -> w81
          tunnel: w80 -> [w88 _ _ _]
          tunnel: w78 -> [w96 w143 w164 w177]
          tunnel: [w95 w143 w153 w177] -> w77
          event Timeout {
            n769 = event-data() -> ()  [unwired: 1 in, 1 out]
            n770 = Unbundle By Name(w96) -> ("CNV Runner.Loop Counter"=w93:i32, "CNV Runner.fixed array"=w94:i32[], "Visual Cue Tab"=w91:refnum<vi>)
            n771 = property class="TabCtl (strict)"(reference=w91) -> (reference out=w89:refnum<vi>, "Value"=w90:enum32{"Visual Cue Graph", "Ready", "Rest"})  [unwired: 1 in, 1 out]
            n772 = case shown="\"Ready\"" w90 {
              tunnel: w94 -> [w102 _ _]
              tunnel: w93 -> [w101 w115 w129]
              tunnel: [w100 w114 w128] -> w92
              tunnel: w89 -> [w99 w113 w127]
              tunnel: w88 -> [w98 w112 w126]
              frame "Visual Cue Graph" {
                n773 = case shown="2501" w101 {
                  selector: w101 -> [_ w107]
                  tunnel: w102 -> [_ w110]
                  tunnel: [0 ("CNV Runner.Loop Counter") w108] -> w100
                  tunnel: w99 -> [w104 _]
                  tunnel: w98 -> [_ _]
                  frame 2501 {
                    n774 = property class="TabCtl (strict)"(reference=w104, "Value"=enum32{"Visual Cue Graph", "Ready", "Rest"}."Rest") -> ()  [unwired: 1 in, 2 out]
                  }
                  frame 1, Default {
                    n775 = call "Visual Cue Builder.vi"("fixed array"=w110, "Loop Counter"=w107) -> ("Trigger Point"=w106:bool, "Array"=→"Visual Cue":i32[][])  [unwired: 8 in]
                    n776 = case shown="True" w106 {
                      frame False {
                      }
                      frame True {
                        n777 = call "Soft Trigger.vi"("Value"=i8 100) -> ()  [unwired: 10 in, 1 out]
                      }
                    }
                    n778 = Increment(x=w107) -> (x+1=w108:i32)
                  }
                }
              }
              frame "Ready" {
                n779 = case shown="0, Default" w115 {
                  selector: w115 -> [w117 w119 _]
                  tunnel: [w116 w118 0 ("CNV Runner.Loop Counter")] -> w114
                  tunnel: w113 -> [_ _ w124]
                  tunnel: w112 -> [_ w120 _]
                  frame 0, Default {
                    n780 = Increment(x=w117) -> (x+1=w116:i32)
                  }
                  frame 1500 {
                    n781 = Increment(x=w119) -> (x+1=w118:i32)
                    n782 = call-poly <vilib>:"Delacor_lib_QMH_Enqueue Message (poly).vi"("Priority Message? (F)"=TRUE, "Message"="Start Buff Fill", "Message Queue in"=w120) -> ()  [unwired: 7 in, 2 out]
                  }
                  frame 2001 {
                    n783 = property class="TabCtl (strict)"(reference=w124, "Value"=enum32{"Visual Cue Graph", "Ready", "Rest"}."Visual Cue Graph") -> ()  [unwired: 1 in, 2 out]
                  }
                }
              }
              frame "Rest", Default {
                n784 = case shown="1501" w129 {
                  selector: w129 -> [w131 w139 _]
                  tunnel: [w130 w138 0 ("CNV Runner.Loop Counter")] -> w128
                  tunnel: w127 -> [_ _ w141]
                  tunnel: w126 -> [_ w137 _]
                  frame 0, Default {
                    n785 = Increment(x=w131) -> (x+1=w130:i32)
                  }
                  frame 1000 {
                    n786 = call-poly <vilib>:"Delacor_lib_QMH_Enqueue Message (poly).vi"("Priority Message? (F)"=TRUE, "Message"="Stop Buff Fill", "Message Queue in"=w137) -> ("error out"=w135:errorcluster, "Message Queue out"=w136:refnum<class "Delacor_lib_QMH_Message Queue.lvclass">)  [unwired: 7 in]
                    n787 = Increment(x=w139) -> (x+1=w138:i32)
                    n788 = call-poly <vilib>:"Delacor_lib_QMH_Enqueue Message (poly).vi"("error in"=w135, "Message"="Analyze Buff", "Message Queue in"=w136) -> ()  [unwired: 7 in, 2 out]
                  }
                  frame 1501 {
                    n789 = property class="TabCtl (strict)"(reference=w141, "Value"=enum32{"Visual Cue Graph", "Ready", "Rest"}."Ready") -> ()  [unwired: 1 in, 2 out]
                  }
                }
              }
            }
            n790 = Bundle By Name(cluster=w96, "CNV Runner.Loop Counter"=w92) -> (w95:T8)
            n791 = Wait Until Next ms Multiple(millisecond multiple=u32 1) -> ()  [unwired: 1 out]
          }
          event User Event {
            n792 = event-data() -> ()  [unwired: 1 in, 1 out]
          }
          event User Event {
            # "This module called the \"Private.Wake-up CNV Demo Loop\" private request."
            n793 = event-data() -> ()  [unwired: 1 in, 1 out]
            n794 = control-ref of="CNV Graph"() -> (w151:refnum<vi>)
            n795 = control-ref of="Visual Cue Tab"() -> (w166:refnum<vi>)
            n796 = control-ref of="Visual Cue"() -> (w162:refnum<vi>)
            n797 = control-ref of="Display CNV Tab"() -> (w165:refnum<vi>)
            n798 = Bundle By Name(cluster=w164, "Visual Cue Tab"=w166, "Display CNV Tab"=w165, "Visual Cue Graph"=w162, "CNV Graph"=w151, "CNV Runner.Loop Counter"=u16 0, "CNV Runner.fixed array"=i32[] array[10000 elements] ("appended array")) -> (w153:T8)
            n799 = Unbundle By Name(w153) -> ("Visual Cue Tab"=w161:refnum<vi>, "Display CNV Tab"=w159:refnum<vi>, "Visual Cue Graph"=w157:refnum<vi>, "CNV Graph"=w156:refnum<vi>)
            n800 = invoke class="WFGraph (strict)" method="Reinit To Default"(reference=w157) -> (error out=w150:errorcluster)  [unwired: 2 in, 2 out]
            n801 = invoke class="WFGraph (strict)" method="Reinit To Default"(reference=w156) -> ()  [unwired: 2 in, 3 out]
            n802 = property class="TabCtl (strict)"(reference=w159, "Value"=enum32{"Empty", "Graph"}."Graph") -> ()  [unwired: 1 in, 2 out]
            n803 = property class="TabCtl (strict)"(reference=w161, "Value"=enum32{"Visual Cue Graph", "Ready", "Rest"}."Ready") -> ()  [unwired: 1 in, 2 out]
            n804 = call "Set CNV Montage.vi"("error in"=w150) -> ("error out"=w149:errorcluster)  [unwired: 10 in]
            n805 = call-poly <userlib>:"MGI Wait.vi"("ms"=u32 2, "Error In"=w149) -> ("Error Out"=w148:errorcluster)  [unwired: 5 in]
            n806 = call "Start CNV Acquiring.vi"("error in"=w148) -> ("error out"=w152:errorcluster)  [unwired: 10 in]
          }
          event User Event {
            # "This module called the \"Private.Sleep CNV Demo Loop\" private request."
            n807 = event-data() -> ()  [unwired: 1 in, 1 out]
            n808 = Unbundle By Name(w177) -> ("Visual Cue Tab"=w174:refnum<vi>, "Display CNV Tab"=w173:refnum<vi>)
            n809 = property class="TabCtl (strict)"(reference=w173, "Value"=enum32{"Empty", "Graph"}."Empty") -> ()  [unwired: 1 in, 2 out]
            n810 = property class="TabCtl (strict)"(reference=w174, "Value"=enum32{"Visual Cue Graph", "Ready", "Rest"}."Rest") -> (error out=w167:errorcluster)  [unwired: 1 in, 1 out]
            n811 = call "Command_GoToIdle.vi"("error in"=w167) -> ("error out"=w172:errorcluster)  [unwired: 10 in]
            n812 = call-poly <userlib>:"MGI Wait.vi"("ms"=u32 5, "Error In"=w172) -> ("Error Out"=w170:errorcluster)  [unwired: 5 in]
            n813 = call "Stop Logging.vi"("error in (no error)"=w170) -> ("error out"=w169:errorcluster)  [unwired: 10 in]
            n814 = call "Stop Acquiring.vi"("error in (no error)"=w169) -> ("error out"=w168:errorcluster)  [unwired: 10 in]
          }
        }
        n815 = call-dynamic "Delacor_lib_QMH_Error Handler - Helper Loop.vi"("Error Debug"=w79, "error in"=w81, "Message Queue in"=w80) -> ()  [unwired: 7 in, 2 out]
      }
      n816 = Unregister For Events(event registration refnum=w66) -> ()  [unwired: 1 in, 1 out]
      n817 = Unregister For Events(event registration refnum=w62) -> ()  [unwired: 1 in, 1 out]
    }
    frame Error {
      w1640 = TRUE ("Wait for Module to Stop? (F)")
      # "Synchronize Caller Events.vi will inform Start Module.vi that the module has launched and will let the code calling Start Module.vi register for broadcasts and would permit the caller receive the broadcast that an error occurred at launch time."
      n818 = call-dynamic "Delacor_lib_QMH_Release Message Queue.vi"("error in"=w1637, "Message Queue"=w1638) -> ("error out"=w1636:errorcluster)  [unwired: 9 in]
      n819 = call "Synchronize Caller Events.vi"("Singleton Module Admin in"=w1641) -> ("error out"=w1646:errorcluster)  [unwired: 9 in, 1 out]
      n820 = call "Module Name--constant.vi"() -> ("Module Name"=w1644:string)  [unwired: 11 in]
      n821 = call "Module Name--constant.vi"() -> ("Module Name"=w1639:string)  [unwired: 11 in]
      n822 = call "Stop Module.vi"("Wait for Module to Stop? (F)"=w1640, "Origin"=w1639) -> ()  [unwired: 9 in, 1 out]
      n823 = call "Stop Module.vi"("Wait for Module to Stop? (F)"=w1640, "Origin"=w1639) -> ()  [unwired: 9 in, 1 out]
      n824 = call "Stop Module.vi"("Wait for Module to Stop? (F)"=w1640, "Origin"=w1639) -> ()  [unwired: 9 in, 1 out]
      n825 = Format Into String(format string="An error occurred during initialization. %s is no longer running.", w1644) -> (resulting string=w1642:string)  [unwired: 2 in, 1 out]
      n826 = Merge Errors(w1636, w1646) -> (w1647:errorcluster)
      n827 = call "Error Reported.vi"("Additional Information"=w1642, "Error"=w1647) -> ()  [unwired: 9 in, 1 out]
    }
  }
  n828 = Merge Errors(w39, w42) -> (w38:errorcluster)
  n829 = call "Close Module.vi"("error in (no error)"=w38, "Module Admin in"=w28) -> ("error out"=w40:errorcluster, "External Launch"=w22:bool, "Module Admin out"=w23:refnum<class "Delacor_lib_QMH_Module Admin.lvclass">)  [unwired: 7 in]
  n830 = Unregister For Events(event registration refnum=w27, error in=w40) -> (error out=w37:errorcluster)
  "error out" <- w37
  n831 = case "External Launch?" shown="True" w22 {
    tunnel: w37 -> [_ w1648]
    frame False {
    }
    frame True {
      n832 = case shown="No Error" w1648 {
        frame No Error {
          n833 = invoke class="VI" method="FP.Close"() -> ()  [unwired: 3 in, 3 out]
        }
        frame Error {
          n834 = invoke on="Invoke Node" class="VI" method="FP.Open"("Activate"=TRUE ("Activate?")) -> ()  [unwired: 4 in, 5 out]
        }
      }
    }
  }
  n835 = local write "Module Admin"(w23) -> ()
